vi "IRF measurement.vi"() -> ()   [LabVIEW 2019]
doc: "Main VI for FLS imaging system."
uses:
  <vilib>/event_ctls.llb/usereventprio.ctl
  <instrlib>/niScope/Acquire/Fetch/niScope Multi Fetch Binary 16.vi
  <instrlib>/niScope/Controls/niScope trigger source.ctl
  LaguerreDeconLib/DeconEngineClass/LaguerreDeconEngineClass.lvclass
  SubVI/GlobalVariables.vi
  SubVI/LabJack/LJ Pin Setting.ctl
  <vilib>/Utility/error.llb/DialogType.ctl
  <vilib>/Analysis/NI_AALBase.lvlib
  <vilib>/Utility/miscctls.llb/LVMinMaxIncTypeDef.ctl
  <vilib>/Analysis/baseanly.llb/Mean (DBL).vi
  <vilib>/Utility/miscctls.llb/LVPointTypeDef.ctl
  <vilib>/Instr/_visa.llb/VISA Configure Serial Port (Instr).vi
  SubVI/DigitizerConfiguration/FLImDAQ.ctl
panel:
  out "Record Backlog":i32
  out "Fetch Record #":i32
  out "error out 2":errorcluster caption="error out"
  out "error out":errorcluster
  out "Sync Success?":bool
  out "Disclamer":picture
  out "Calibration #":i8
  out "BG #":i8
  in  "TCP Connect":bool
  out "Help":string
  in  "355nm Laser toggle":bool caption="355nm 750Hz"
  in  "Cali&iRF alignment":bool
  in  "Background":bool
  in  "Aiming beam toggle":bool caption="445nm 15Hz 20mA"
  in  "Auto gain ch3":bool=TRUE
  in  "Auto gain ch2":bool=TRUE
  in  "Auto gain ch1":bool=TRUE
  out "Run #":i8
  in  "StopButton":bool caption="Stop"
  out "Aquisition Status:":bool
  in  "StartButton":bool caption="Start"
  in  "Gain 3":dbl min=0.0 max=4.6 step=0.1
  in  "Gain 2":dbl min=0.0 max=4.6 step=0.1
  in  "Gain 1":dbl min=0.0 max=4.6 step=0.1 format="%#_4g"
  in  "Video Source":enum32{"Camera", "FrameGrabber"}(radio)
  out "Case #":string
  out "System Hardware Connection Status":T1
  out "Channel 3":dbl[][](graph)
  out "Channel 2":dbl[][](graph)
  out "Channel 1":dbl[][](graph)
  in  "Tab Control":T2(tab)
  out "Aq L?":bool
  out "ML?":bool
  out "display loop timing(ms)":u32
  out "Aquisition loop timing(ms)":u32
  out "DisplayLoop":i32
  out "processing loop":i32
  out "processing loop timing(ms)":dbl
  in  "V target(1.5)":dbl=1.3 format="%#_13g"
  out "laser EM lamp V":dbl format="%0.6f"
  in  "Show BG":bool
  out "SysConfigCluster":T3
  out "LJ Pinout":T4={"Ch1 Bias"="DAC0", "Ch2 Bias"="DAC1", "Ch3 Bias"="DAC2", "355 PWM"="FIO0", "AimingBeam PWM"="FIO2", "Laser Ready"="FIO3", "Interlock"="FIO1", "Laser Start/Stop"="FIO1", "Red LED"="FIO1", "Green LED"="DIO3", "Foot Pedal"="DIO15"}
  out "FLImDAQ":T5={"Digitizer 1"="", "Digitizer 2"="", "Channel"=enum."Channel 0", "trigger source"="VAL_EXTERNAL", "trigger level"=0.5, "trigger delay"=1.35e-07, "min sample rate"=12500000000.0, "min record length"=2500, "vertical range"=1.0, "vertical offset"=-0.25, "Waveform to Avg"=2000} caption="FLIm DAQ Configuration" {"trigger delay" format="%^#.4e"; "trigger level" min=0.0 max=3.5 step=0.5 format="%.2f"; "vertical offset" format="%.4f"; "vertical range" format="%.2f"; "min sample rate" format="%#.2p"}
  out "Dig1 Temp":dbl
  out "Dig2 Temp":dbl
  in  "Sys Reconfig":bool
  out "syctimer data out":string
  out "processing Error Out":errorcluster
  out "aquisition loop Error Out":errorcluster
  out "V1":dbl[](array[numeric])
  out "V2":dbl[](array[numeric])
  out "V3":dbl[](array[numeric])
  out "V1 Size":i32
  out "V2 Size":i32
  out "V3 Size":i32
  out "data Size":i32[](array[numeric])
  out "State log":string
  in  "Quit":bool
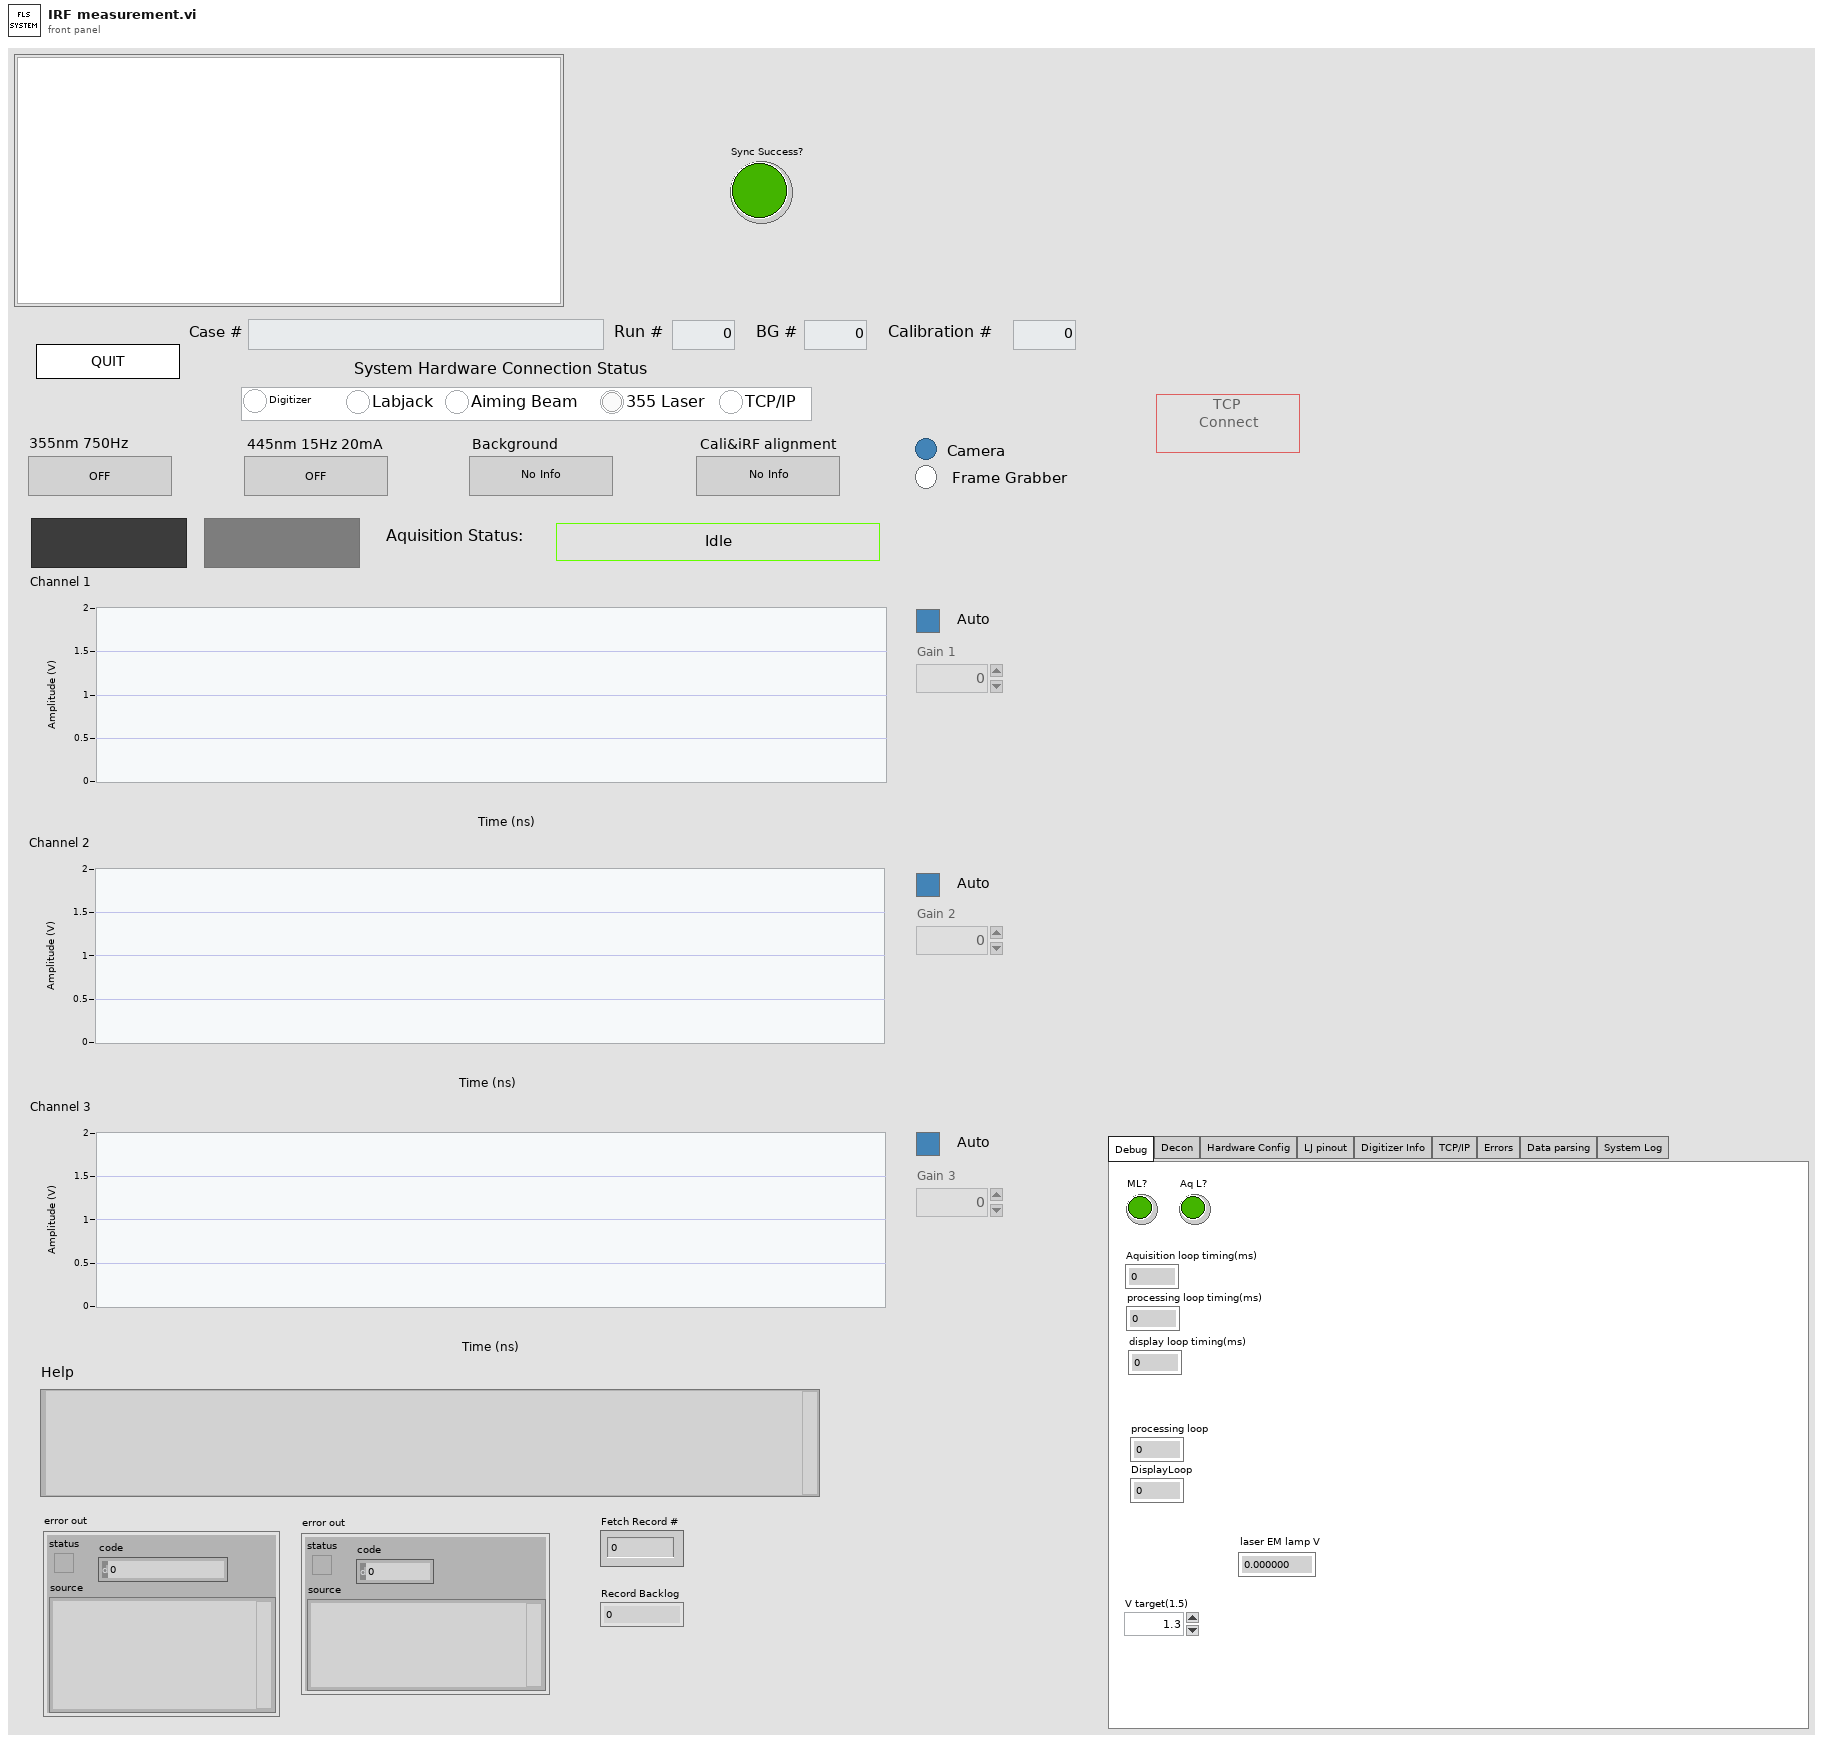
[diagram p1: front panel]
types:
  T1 = cluster{"Digitizer":bool, "Labjack":bool, "Aiming Beam":bool, "355 Laser":bool, "TCP/IP":bool}
  T2 = enum32{"Debug", "Decon", "Hardware Config", "LJ pinout", "Digitizer Info", "TCP/IP", "Errors", "Data parsing", "System Log"}
  T3 = cluster{"Ch1Enable?":bool, "Ch2Enable?":bool, "Ch3Enable?":bool, "Ch1AutoGain?":bool, "Ch2AutoGain?":bool, "Ch3AutoGain?":bool, "AimingBeamEnable?":bool}
  T4 = typedef "LJ Pin Setting.ctl" = cluster{"Ch1 Bias":string, "Ch2 Bias":string, "Ch3 Bias":string, "355 PWM":string, "AimingBeam PWM":string, "Laser Ready":string, "Interlock":string, "Laser Start/Stop":string, "Red LED":string, "Green LED":string, "Foot Pedal":string}
  T5 = typedef "FLImDAQ.ctl" = cluster{"Digitizer 1":refnum<k15>, "Digitizer 2":refnum<k15>, "Channel":enum16{"Channel 0", "Channel 1", "Channel 0&1"}, "trigger source":T6, "trigger level":dbl, "trigger delay":dbl, "min sample rate":dbl, "min record length":i32, "vertical range":dbl, "vertical offset":dbl, "Waveform to Avg":i32}
  T6 = typedef "niScope trigger source.ctl" = string
  T7 = enum8{"Enabled", "Disabled", "Disabled and Grayed Out"}
  T8 = typedef "LVPointTypeDef.ctl" = cluster{"Horizontal":i16, "Vertical":i16}
  T9 = cluster{"CH1":dbl[][], "CH2":dbl[][], "CH3":dbl[][]}
  T10 = cluster{"idx":i32, "CH1&2":dbl[][], "CH3":dbl[][]}
  T11 = enum16{"open", "open or create", "create or replace", "create", "open (read-only)"}
  T12 = enum32{"Invalid", "Standard", "Closed", "Hidden", "Minimized", "Maximized"}
  T13 = enum32{"invalid app kind", "Development System", "Run Time System", "Student Edition", "Embedded LabVIEW", "Evaluation", "Custom"}
  T14 = typedef "usereventprio.ctl" = enum32{"high priority", "normal priority"}
  T15 = enum16{"Standard", "Buffered", "CRLF", "Immediate"}
  T16 = cluster{"Core":cluster{"Current VI Reference":refnum<vi>, "Close Panel on Exit?":bool}, "SysConfigCluster":cluster{"Ch1Enable?":bool, "Ch2Enable?":bool, "Ch3Enable?":bool, "Ch1AutoGain?":bool, "Ch2AutoGain?":bool, "Ch3AutoGain?":bool, "AimingBeamEnable?":bool}, "System Status":cluster{"Digitizer":bool, "Labjack":bool, "Aiming Beam":bool, "355 Laser":bool, "TCP/IP":bool}, "IDs":cluster{"RunID":i8, "BG ID":i8, "Cali ID":i8}, "CaseID":string, "DefaultPath":path, "Pathes":cluster{"DataPath":path, "BG Path":path, "iRFPath":path, "CaliPath":path}, "FLImDAQ":cluster{"resource name":refnum<k15>, "resource name 2":refnum<k15>, "Channel":enum16{"Channel 0", "Channel 1", "Channel 0&1"}, "trigger source":T6, "trigger level":dbl, "trigger delay":dbl, "min sample rate":dbl, "min record length":i32, "vertical range":dbl, "vertical offset":dbl, "Waveform to Avg":i32}, "SysRunning?":bool, "AB Cluster":cluster{"Aiming Beam COM Port":refnum<visa-resource-name>, "Min Current":dbl, "Max Current":dbl, "Default Current":dbl, i32}, "LJ Pinout":T4, "355 PWM setting":cluster{"DIO_EF_CLOCK1_DIVISOR":i16, "DIO_EF_CLOCK1_ROLL_VALUE":i32, "DIO#_EF_INDEX":i16, "DIO#_EF_OPTIONS":i16, "DIO#_EF_CONFIG_A":i32}, "AB PWM setting":cluster{"DIO_EF_CLOCK1_DIVISOR":i16, "DIO_EF_CLOCK1_ROLL_VALUE":i32, "DIO#_EF_INDEX":i16, "DIO#_EF_OPTIONS":i16, "DIO#_EF_CONFIG_A":i32}, "Last Trigger":u32, "niTClk sessions":refnum<k20>[], "Laser start tic":u32, "TCP attempt count":i32, "Ch1Data":dbl[][], "Ch2Data":dbl[][], "Ch3Data":dbl[][], "V1":dbl[], "V2":dbl[], "V3":dbl[], "SlowTimer":u32, "FastTimer":u32, "listener ID":refnum<k5>, "TempPath":path, "LED vi reference":refnum<vi>}
  T17 = typedef "LVCursorListTypeDef.ctl" = cluster{"Name":string, "Color":u32, "Style":u8, "Point Style":u8, "Name Visible":bool, "Allow Drag":bool, "Cursor Mode":u32, "Plot":i32, "Index":i32, "Position":cluster{"X":dbl, "Y":dbl}, "X Scale":u32, "Y Scale":u32, "Watch Plots":i32[], "Watch All Plots":bool, "Plot Area":i32, "Label Offset":cluster{"X":dbl, "Y":dbl}}[]
  T18 = cluster{"Name":string, "Color":u32, "Style":u8, "Point Style":u8, "Name Visible":bool, "Allow Drag":bool, "Cursor Mode":u32, "Plot":i32, "Index":i32, "Position":cluster{"X":dbl, "Y":dbl}, "X Scale":u32, "Y Scale":u32, "Watch Plots":i32[], "Watch All Plots":bool, "Plot Area":i32, "Label Offset":cluster{"X":dbl, "Y":dbl}}
  T19 = cluster{"DataPath":path, "BG Path":path, "iRFPath":path, "CaliPath":path}
  T20 = cluster{"DIO_EF_CLOCK1_DIVISOR":i16, "DIO_EF_CLOCK1_ROLL_VALUE":i32, "DIO#_EF_INDEX":i16, "DIO#_EF_OPTIONS":i16, "DIO#_EF_CONFIG_A":i32}
  T21 = cluster{"Aiming Beam COM Port":refnum<visa-resource-name>, "Min Current":dbl, "Max Current":dbl, "Default Current":dbl, i32}
  T22 = cluster{"resource name":refnum<k15>, "resource name 2":refnum<k15>, "Channel":enum16{"Channel 0", "Channel 1", "Channel 0&1"}, "trigger source":T6, "trigger level":dbl, "trigger delay":dbl, "min sample rate":dbl, "min record length":i32, "vertical range":dbl, "vertical offset":dbl, "Waveform to Avg":i32}
  T23 = cluster{"Current VI Reference":refnum<vi>, "Close Panel on Exit?":bool}
  T24 = cluster{"1D Avg":dbl[], "1D Avg":dbl[], "1D Avg":dbl[]}
  T25 = typedef "DialogType.ctl" = u16
  T26 = cluster{"Ch1 iRF":dbl[], "Ch2 iRF":dbl[], "Ch3 iRF":dbl[]}
  T27 = typedef "LJ PWM Setting.ctl" = cluster{"DIO_EF_CLOCK1_DIVISOR":i16, "DIO_EF_CLOCK1_ROLL_VALUE":i32, "DIO#_EF_INDEX":i16, "DIO#_EF_OPTIONS":i16, "DIO#_EF_CONFIG_A":i32}
  T28 = typedef "AimingBeam.ctl" = cluster{"Aiming Beam COM Port":refnum<visa-resource-name>, "Min Current":dbl, "Max Current":dbl, "Default Current":dbl, "Frequency(Hz)":u32}
  T29 = typedef "LVMinMaxIncTypeDef.ctl" = cluster{"Minimum":dbl, "Maximum":dbl, "Increment":dbl}
  T30 = typedef "LVBoundsTypeDef.ctl" = cluster{"Width":u32, "Height":u32}
  T31 = typedef "imagedata.ctl" = cluster{"image type":i32, "image depth":i32, "image":u8[], "mask":u8[], "colors":u32[], "Rectangle":cluster{"left":i16, "top":i16, "right":i16, "bottom":i16}}
  T32 = cluster{"V1 out":dbl, "V2 out":dbl, "V3 out":dbl}
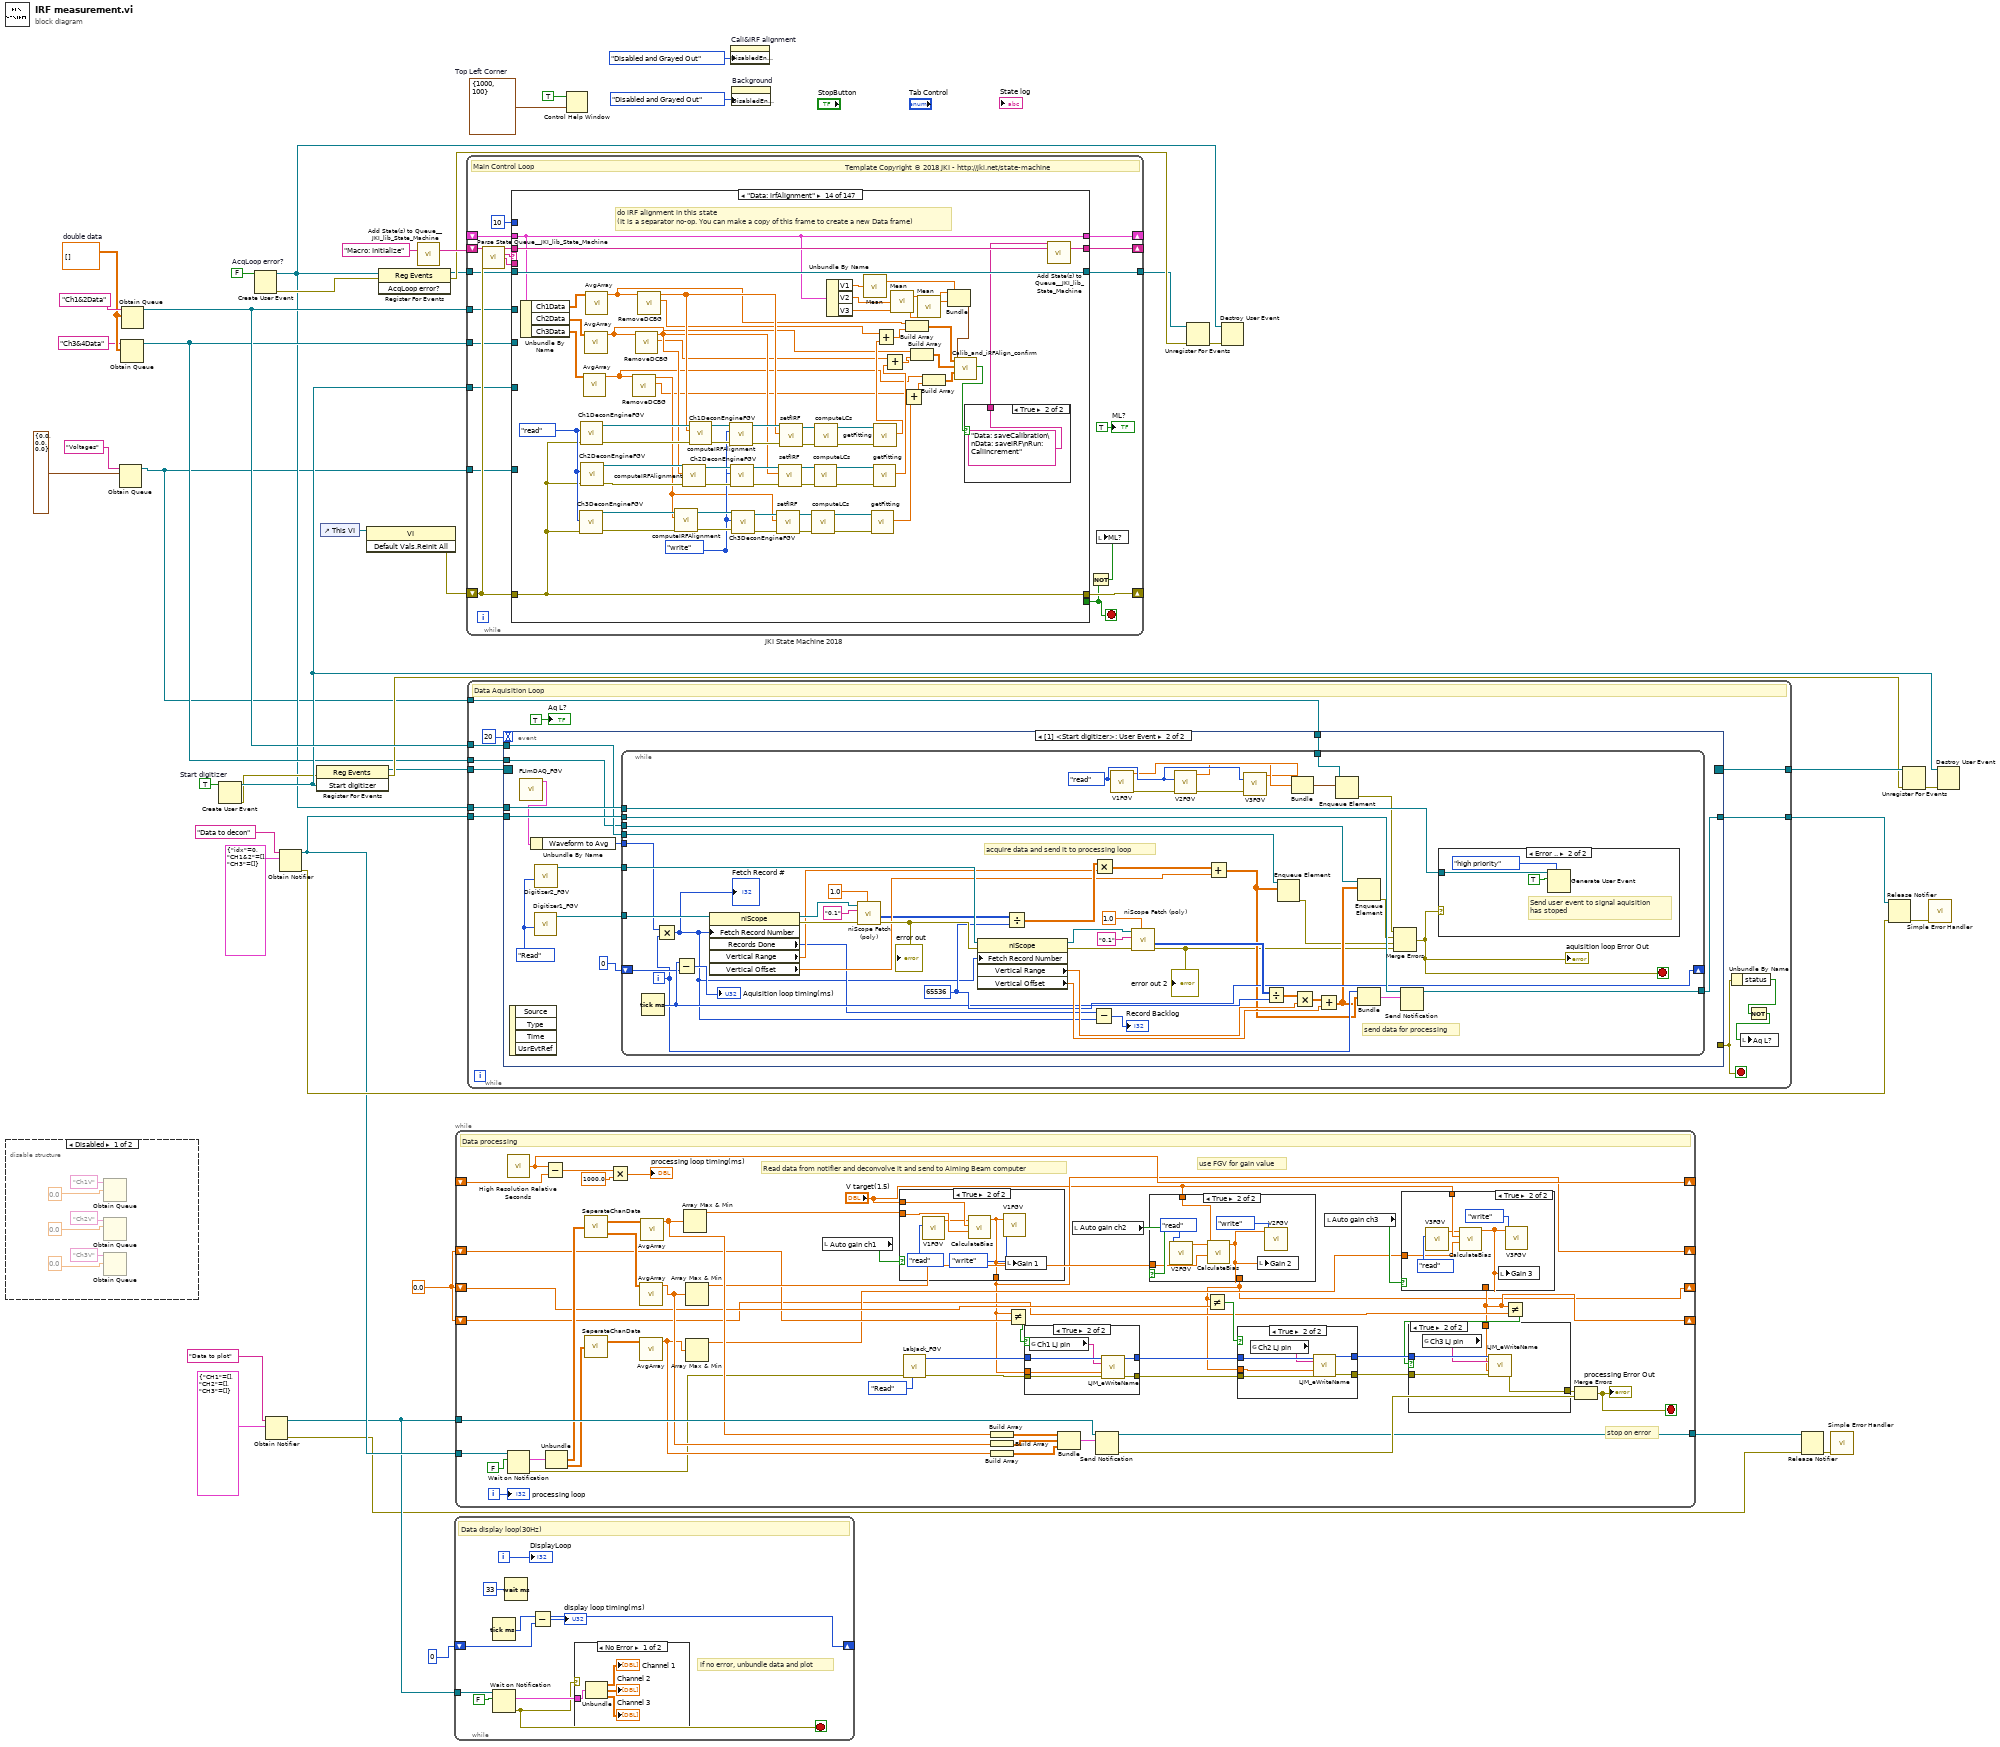
[diagram p0: block diagram]
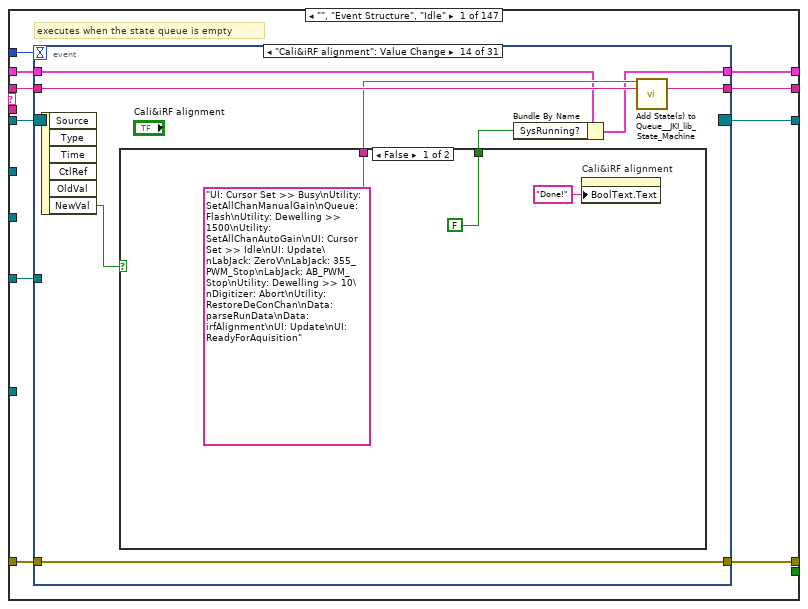
[diagram p3: hidden frame]
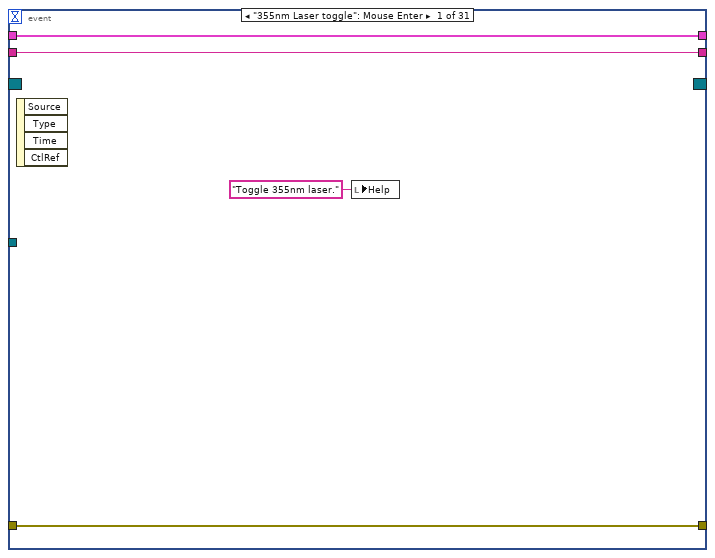
[diagram p4: hidden frame]
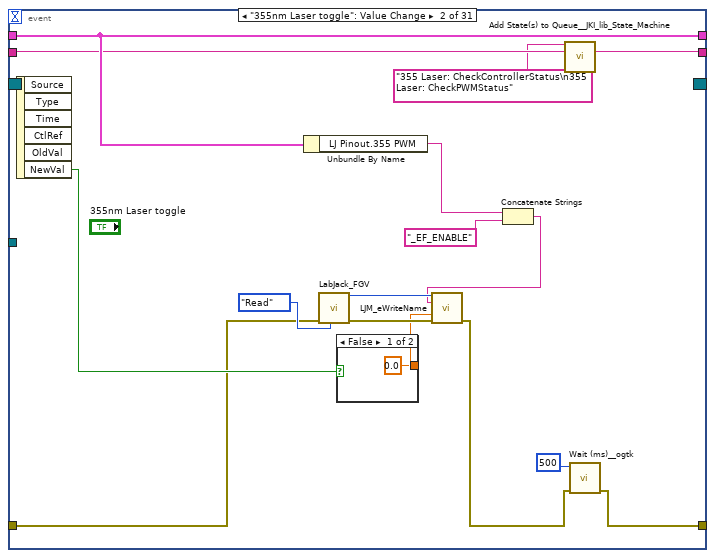
[diagram p5: hidden frame]
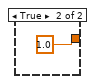
[diagram p6: hidden frame]
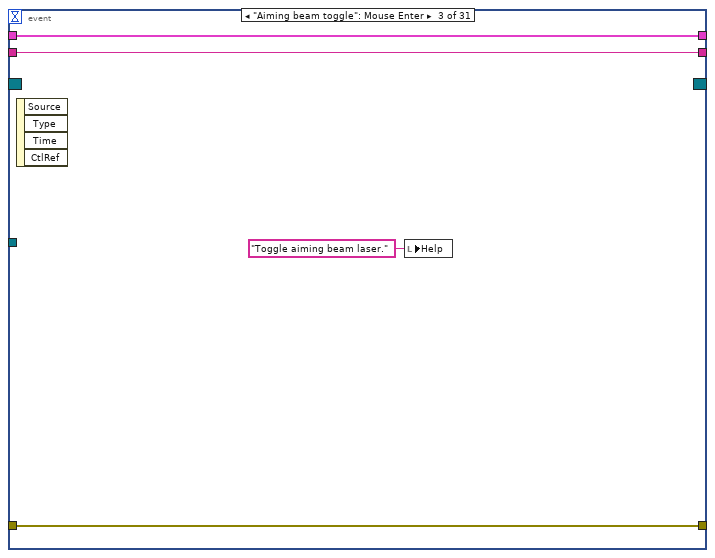
[diagram p7: hidden frame]
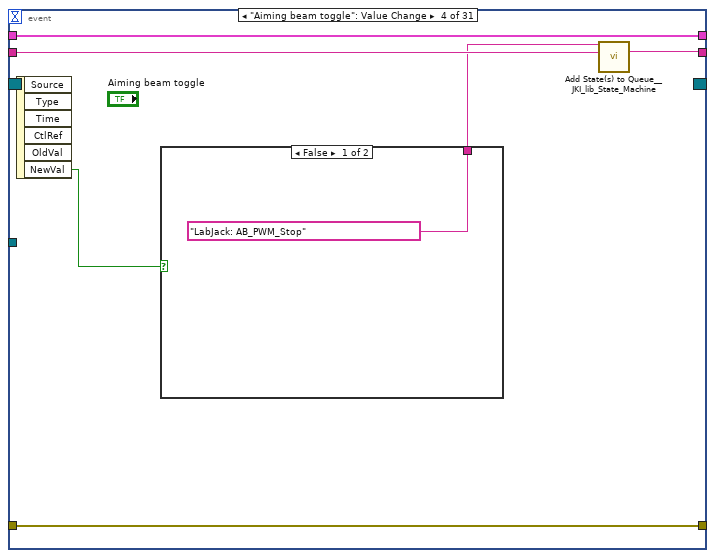
[diagram p8: hidden frame]
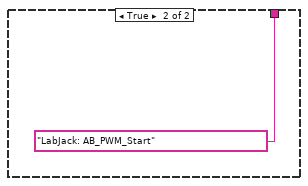
[diagram p9: hidden frame]
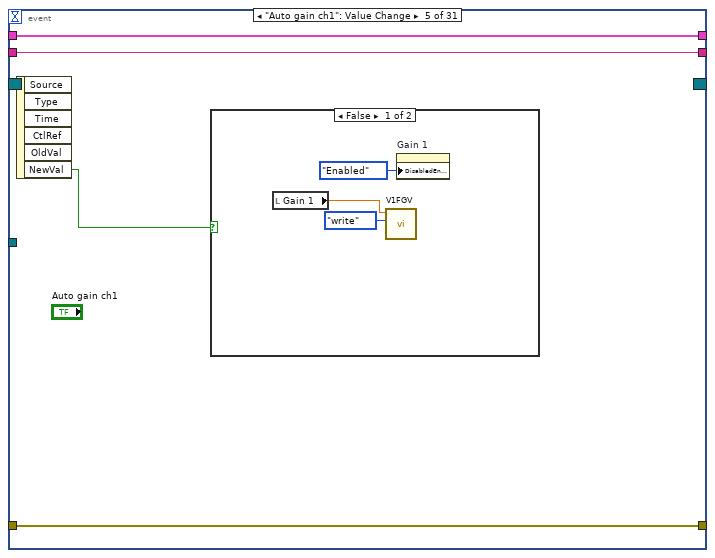
[diagram p10: hidden frame]
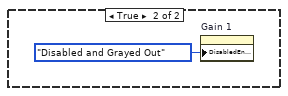
[diagram p11: hidden frame]
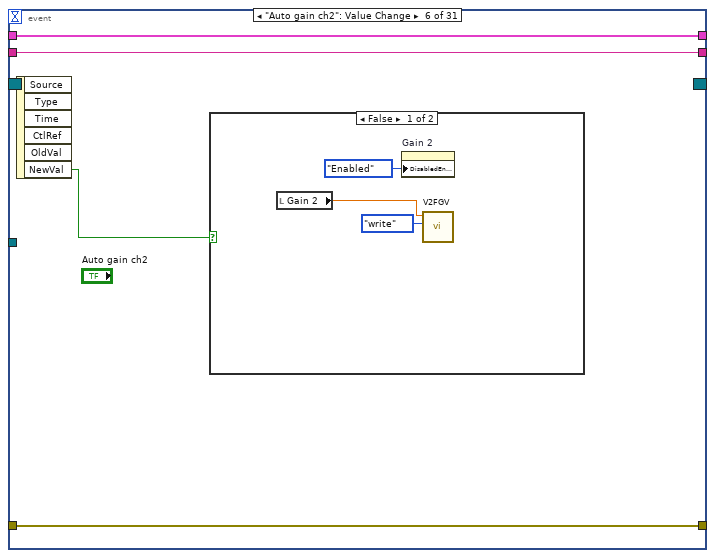
[diagram p12: hidden frame]
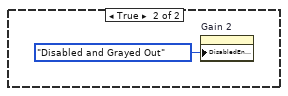
[diagram p13: hidden frame]
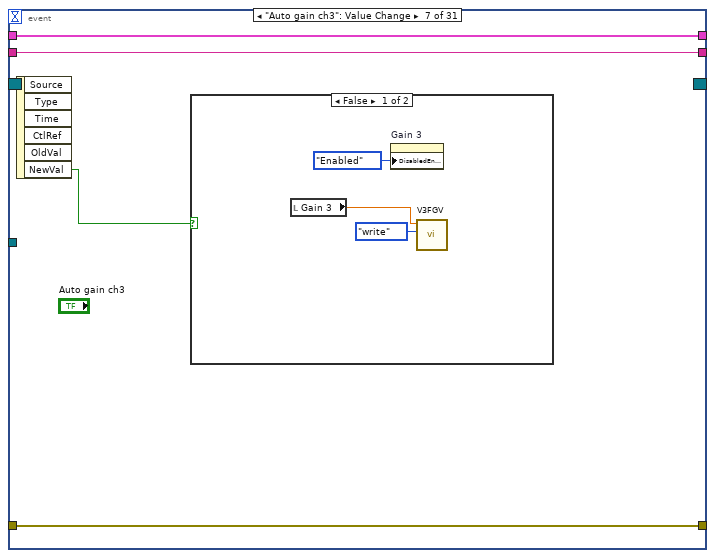
[diagram p14: hidden frame]
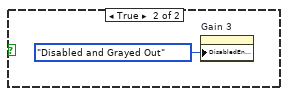
[diagram p15: hidden frame]
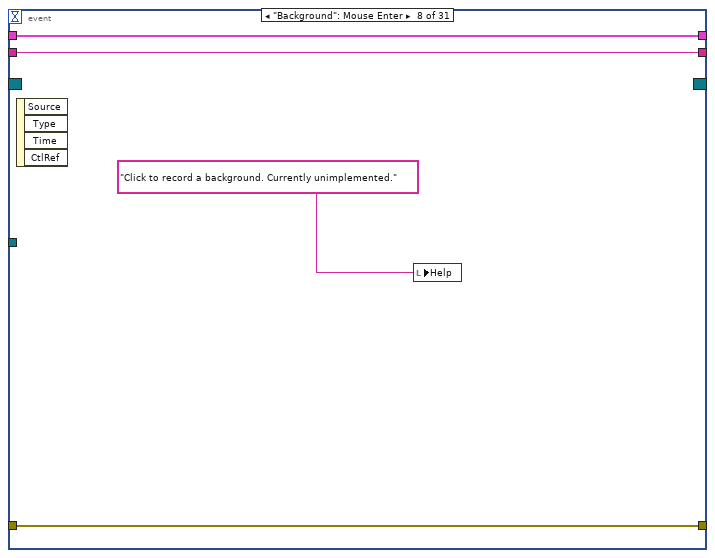
[diagram p16: hidden frame]
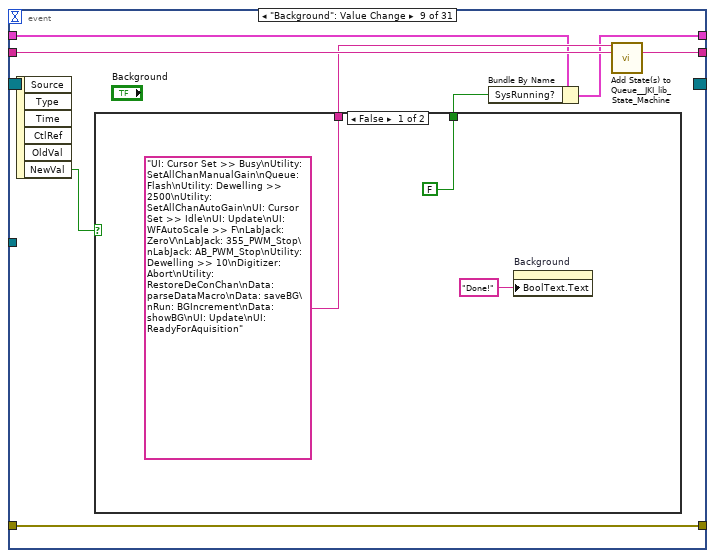
[diagram p17: hidden frame]
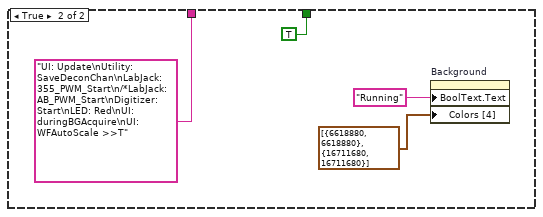
[diagram p18: hidden frame]
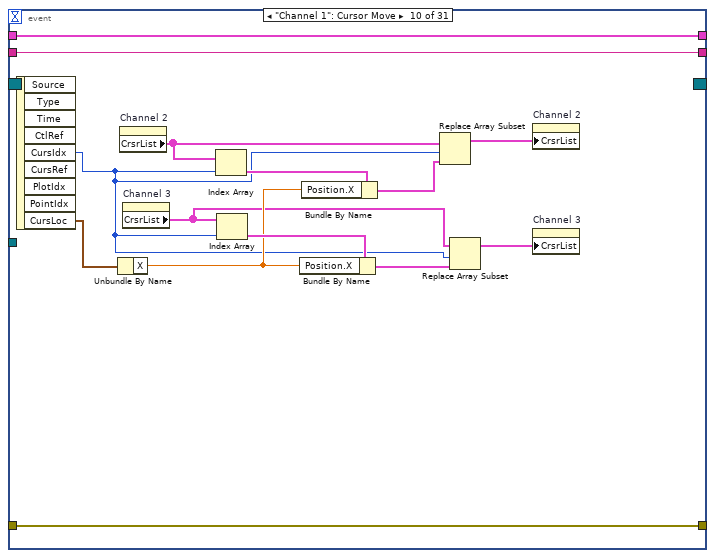
[diagram p19: hidden frame]
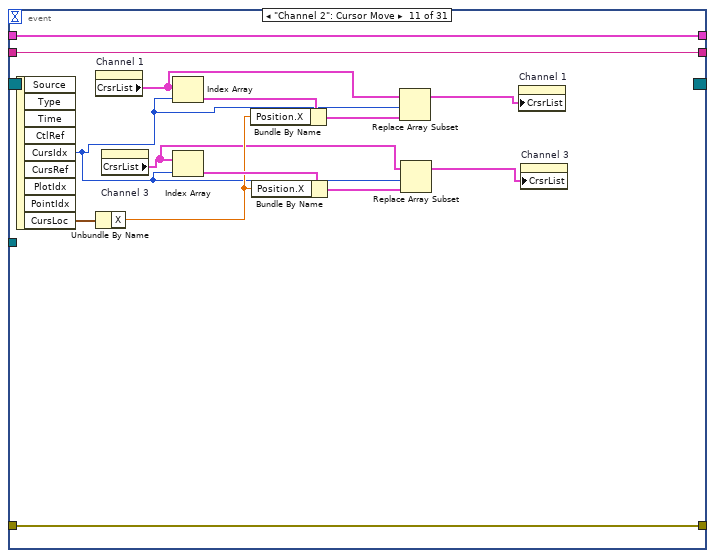
[diagram p20: hidden frame]
diagram:
  w3 = T8 {"Horizontal"=1000, "Vertical"=100}  # Top Left Corner
  w8 = 0.0
  w26 = FALSE  # AcqLoop error?
  w37 = TRUE  # Start digitizer
  w40 = dbl[][] []  # double data
  n1 = disable-structure shown="Disabled" {
    frame Disabled {
      n2 = Obtain Queue(name (unnamed)="Ch1V", element data type=0.0) -> ()  [unwired: 3 in, 3 out]
      n3 = Obtain Queue(name (unnamed)="Ch2V", element data type=0.0) -> ()  [unwired: 3 in, 3 out]
      n4 = Obtain Queue(name (unnamed)="Ch3V", element data type=0.0) -> ()  [unwired: 3 in, 3 out]
    }
    frame Enabled {
    }
  }
  n5 = Obtain Queue(name (unnamed)="Voltages", element data type=cluster{"V1":dbl, "V2":dbl, "V3":dbl} {"V1"=0.0, "V2"=0.0, "V3"=0.0}) -> (queue out=w5:refnum<queue>)  [unwired: 3 in, 2 out]
  n6 = Obtain Queue(name (unnamed)="Ch3&4Data", element data type=w40) -> (queue out=w14:refnum<queue>)  [unwired: 3 in, 2 out]
  n7 = Obtain Queue(name (unnamed)="Ch1&2Data", element data type=w40) -> (queue out=w38:refnum<queue>)  [unwired: 3 in, 2 out]
  n8 = Create User Event(user event datatype=w37) -> (user event=w25:refnum<user-event>, error out=w10:errorcluster)  [unwired: 1 in]
  n9 = Create User Event(user event datatype=w26) -> (user event=w9:refnum<user-event>, error out=w11:errorcluster)  [unwired: 1 in]
  n10 = Obtain Notifier(name (unnamed)="Data to plot", notification data type=T9 {"CH1"=[], "CH2"=[], "CH3"=[]}) -> (notifier out=w18:refnum<notifier>, error out=w15:errorcluster)  [unwired: 2 in, 1 out]
  n11 = Obtain Notifier(name (unnamed)="Data to decon", notification data type=T10 {"idx"=0, "CH1&2"=[], "CH3"=[]}) -> (notifier out=w21:refnum<notifier>, error out=w31:errorcluster)  [unwired: 2 in, 1 out]
  n12 = register-events(error in=w10, w25) -> (reference out=w27:refnum<event-registration>, error out=w34:errorcluster)  [unwired: 1 in]
  n13 = control-ref of="This VI"() -> (w42:refnum<vi>)
  n14 = invoke class="VI" method="Default Vals.Reinit All"(reference=w42) -> (error out=w28:errorcluster)  [unwired: 2 in, 2 out]
  n15 = register-events(error in=w11, w9) -> (reference out=w13:refnum<event-registration>, error out=w23:errorcluster)  [unwired: 1 in]
  n16 = call <vilib>:"Add State(s) to Queue__JKI_lib_State_Machine.vi"("State(s) in (\"\")"="Macro: Initialize") -> ("States Out"=w44:string)  [unwired: 14 in]
  n17 = while {
    tunnel: w18 -> [w59]
    shift-right: [w53] -> _
    shift-left: u32 0 ("millisecond timer value") -> [w57]
    i -> [w51]
    stop <- w52 stop-if-true
    # "if no error, unbundle data and plot"
    # "Data display loop(30Hz)"
    n18 = Tick Count (ms)() -> (millisecond timer value=w53:u32)
    n19 = Wait on Notification(notifier=w59, ignore previous (F)=FALSE) -> (notification=w54:T9, error out=w52:errorcluster)  [unwired: 2 in, 2 out]
    n20 = Wait (ms)(milliseconds to wait=u32 33) -> ()  [unwired: 1 out]
    n21 = Subtract(x=w53, y=w57) -> (x-y=→"display loop timing(ms)":u32)
    n22 = case shown="No Error" w52 {
      tunnel: w54 -> [w63 _]
      frame No Error {
        n23 = Unbundle(w63) -> ("CH1"=→"Channel 1":dbl[][], "CH2"=→"Channel 2":dbl[][], "CH3"=→"Channel 3":dbl[][])
      }
      frame Error {
      }
    }
    "DisplayLoop" <- w51
  }
  n24 = while {
    tunnel: w21 -> [w113]
    shift-right: [w66] -> _
    shift-left: w8 -> [w73]
    tunnel: w18 -> [w105]
    tunnel: [w102] -> w17
    shift-right: [w101] -> _
    shift-left: _ -> [w100]
    shift-right: [w67] -> _
    shift-left: w8 -> [w74]
    shift-right: [w68] -> _
    shift-left: w8 -> [w70]
    i -> [w81]
    stop <- w64 stop-if-true
    # "use FGV for gain value"
    # "stop on error"
    # "Read data from notifier and deconvolve it and send to Aiming Beam computer"
    # "Data processing"
    n25 = call <vilib>:"High Resolution Relative Seconds.vi"() -> ("relative seconds"=w101:dbl)
    n26 = Wait on Notification(notifier=w113, ignore previous (F)=FALSE) -> (notification=w111:T10, error out=w84:errorcluster)  [unwired: 2 in, 2 out]
    n27 = Subtract(x=w101, y=w100) -> (x-y=w99:dbl)
    n28 = Unbundle(w111) -> ("CH1&2"=w83:dbl[][], "CH3"=w82:dbl[][])  [unwired: 1 out]
    n29 = call "SeperateChanData.vi"("Input (Ch1&2)"=w83) -> ("Ch1"=w85:dbl[][], "Ch2"=w90:dbl[][])
    n30 = call "SeperateChanData.vi"("Input (Ch1&2)"=w82) -> ("Ch1"=w110:dbl[][])  [unwired: 1 out]
    n31 = Multiply(x=w99, y=1000.0) -> (x*y=→"processing loop timing(ms)":dbl)
    n32 = call "AvgArray.vi"("2D array"=w90) -> ("1D Avg"=w96:dbl[])  [unwired: 10 in]
    n33 = call "AvgArray.vi"("2D array"=w110) -> ("1D Avg"=w89:dbl[])  [unwired: 10 in]
    n34 = call "AvgArray.vi"("2D array"=w85) -> ("1D Avg"=w103:dbl[])  [unwired: 10 in]
    n35 = Array Max & Min(array=w103) -> (max value=w77:dbl)  [unwired: 3 out]
    n36 = Array Max & Min(array=w96) -> (max value=w75:dbl)  [unwired: 3 out]
    n37 = Array Max & Min(array=w89) -> (max value=w71:dbl)  [unwired: 3 out]
    n38 = local read "Auto gain ch1"() -> (w80:bool)
    n39 = case shown="True" w80 {
      tunnel: [w152 w156] -> w66
      tunnel: w77 -> [_ w158]
      tunnel: "V target(1.5)" -> [_ w157]
      frame False {
        n40 = call "V1FGV.vi"("action"=enum16{"write", "read"}."read") -> ("V1 out"=w152:dbl)  [unwired: 9 in, 1 out]
      }
      frame True {
        n41 = call "V1FGV.vi"("action"=enum16{"write", "read"}."read") -> ("V1 out"=w154:dbl)  [unwired: 9 in, 1 out]
        n42 = call "CalculateBias.vi"("GainV Last"=w158, "Sig Current(V)"=w157, "GainV current"=w154) -> ("V new"=w156:dbl)  [unwired: 8 in]
        n43 = call "V1FGV.vi"("action"=enum16{"write", "read"}."write", "V1 in"=w156) -> ()  [unwired: 8 in, 2 out]
        n44 = local write "Gain 1"(w156) -> ()
      }
    }
    n45 = call "LabJack_FGV.vi"("Operation(Read)"=enum16{"Write", "Read"}."Read" ("Operation"), "error in (no error)"=w84) -> ("error out"=w109:errorcluster, "Read data"=w108:i32)  [unwired: 8 in]
    n46 = Build Array(w103) -> (w88:dbl[][])
    n47 = Build Array(w96) -> (w87:dbl[][])
    n48 = Build Array(w89) -> (w86:dbl[][])
    n49 = Not Equal?(x=w66, y=w73) -> (x != y?=w76:bool)
    n50 = case shown="True" w76 {
      tunnel: w109 -> [w129 w135]
      tunnel: w108 -> [w128 w134]
      tunnel: [w129 w133] -> w95
      tunnel: [w128 w132] -> w92
      tunnel: w66 -> [_ w130]
      frame False {
      }
      frame True {
        n51 = global read "GlobalVariables.vi" "Ch1 LJ pin"() -> (w131:string)
        n52 = call <vilib>:"LJM_eWriteName.vi"("Handle In"=w134, "Name"=w131, "Value"=w130, "error in"=w135) -> ("Handle Out"=w132:i32, "error out"=w133:errorcluster)  [unwired: 10 in]
      }
    }
    n53 = Bundle(w88, w87, w86) -> (w106:cluster{dbl[][], dbl[][], dbl[][]})  [unwired: 1 in]
    n54 = local read "Auto gain ch2"() -> (w79:bool)
    n55 = Send Notification(notification=w106, notifier=w105) -> (notifier out=w102:refnum<notifier>, error out=w104:errorcluster)  [unwired: 1 in]
    n56 = case shown="True" w79 {
      tunnel: [w144 w146] -> w67
      tunnel: w75 -> [_ w151]
      tunnel: "V target(1.5)" -> [_ w150]
      frame False {
        n57 = call "V2FGV.vi"("action"=enum16{"write", "read"}."read") -> ("V2 out"=w144:dbl)  [unwired: 9 in, 1 out]
      }
      frame True {
        n58 = call "V2FGV.vi"("action"=enum16{"write", "read"}."read") -> ("V2 out"=w148:dbl)  [unwired: 9 in, 1 out]
        n59 = call "CalculateBias.vi"("GainV Last"=w151, "Sig Current(V)"=w150, "GainV current"=w148) -> ("V new"=w146:dbl)  [unwired: 8 in]
        n60 = local write "Gain 2"(w146) -> ()
        n61 = call "V2FGV.vi"("action"=enum16{"write", "read"}."write", "V2 in"=w146) -> ()  [unwired: 8 in, 2 out]
      }
    }
    n62 = Not Equal?(x=w67, y=w74) -> (x != y?=w72:bool)
    n63 = case shown="True" w72 {
      tunnel: w95 -> [w120 w127]
      tunnel: [w120 w126] -> w94
      tunnel: w92 -> [w121 w125]
      tunnel: [w121 w124] -> w91
      tunnel: w67 -> [_ w122]
      frame False {
      }
      frame True {
        n64 = global read "GlobalVariables.vi" "Ch2 LJ pin"() -> (w123:string)
        n65 = call <vilib>:"LJM_eWriteName.vi"("Handle In"=w125, "Name"=w123, "Value"=w122, "error in"=w127) -> ("Handle Out"=w124:i32, "error out"=w126:errorcluster)  [unwired: 10 in]
      }
    }
    n66 = local read "Auto gain ch3"() -> (w78:bool)
    n67 = case shown="True" w78 {
      tunnel: w71 -> [_ w142]
      tunnel: "V target(1.5)" -> [_ w141]
      tunnel: [w136 w138] -> w68
      frame False {
        n68 = call "V3FGV.vi"("action"=enum16{"write", "read"}."read") -> ("V3 out"=w136:dbl)  [unwired: 9 in, 1 out]
      }
      frame True {
        n69 = call "V3FGV.vi"("action"=enum16{"write", "read"}."read") -> ("V3 out"=w140:dbl)  [unwired: 9 in, 1 out]
        n70 = call "CalculateBias.vi"("GainV Last"=w142, "Sig Current(V)"=w141, "GainV current"=w140) -> ("V new"=w138:dbl)  [unwired: 8 in]
        n71 = local write "Gain 3"(w138) -> ()
        n72 = call "V3FGV.vi"("action"=enum16{"write", "read"}."write", "V3 in"=w138) -> ()  [unwired: 8 in, 2 out]
      }
    }
    n73 = Not Equal?(x=w68, y=w70) -> (x != y?=w69:bool)
    n74 = case shown="True" w69 {
      tunnel: w94 -> [w114 w119]
      tunnel: [w114 w118] -> w93
      tunnel: w91 -> [_ w117]
      tunnel: w68 -> [_ w115]
      frame False {
      }
      frame True {
        n75 = global read "GlobalVariables.vi" "Ch3 LJ pin"() -> (w116:string)
        n76 = call <vilib>:"LJM_eWriteName.vi"("Handle In"=w117, "Name"=w116, "Value"=w115, "error in"=w119) -> ("error out"=w118:errorcluster)  [unwired: 10 in, 1 out]
      }
    }
    n77 = Merge Errors(w93, w104) -> (w64:errorcluster)
    "processing Error Out" <- w64
    "processing loop" <- w81
  }
  n78 = while "JKI State Machine 2018" {
    shift-right: [w173] -> _
    shift-left: _ -> [w172]
    shift-right: [w175] -> _
    shift-left: w28 -> [w170]
    shift-right: [w174] -> _
    shift-left: w44 -> [w176]
    tunnel: w38 -> [w169]
    tunnel: w14 -> [w168]
    tunnel: w25 -> [w167]
    tunnel: w13 -> [w166]
    tunnel: [w165] -> w12
    tunnel: w5 -> [w161]
    stop <- w164 stop-if-true
    # "Template Copyright © 2018 JKI - http://jki.net/state-machine"
    # "Main Control Loop"
    n79 = call <vilib>:"Parse State Queue__JKI_lib_State_Machine.vi"("State Queue"=w176, "Error In (no error)"=w170) -> ("Remaining States"=w178:string, "Current State"=w160:string, "Arguments"=w177:string)  [unwired: 11 in]
    n80 = case shown="\"Data: irfAlignment\"" w160 {
      selector: w160 -> [_ _ _ _ _ _ _ _ _ _ _ _ _ _ _ _ _ w846 _ _ _ _ _ _ _ _ _ _ _ _ _ _ _ _ _ _ _ _ _ _ _ _ _ _ _ _ _ _ _ _ _ _ _ _ _ _ _ _ _ _ _ _ _ _ _ _ _ _ _ _ _ _ _ _ _ _ _ _ _ _ _ _ _ _ _ _ _ _ _ _ _ _ _ _ _ _ _ _ _ _ _ _ _ _ _ _ _ _ _ _ _ _ _ _ _ _ _ _ _ _ _ _ _ _ _ _ _ _ _ _ _ _ _ _ _ _ _ _ _ _ _ _ _ _ _ _ _]
      tunnel: w178 -> [w188 w464 w497 w503 w529 w555 w579 w602 w618 w653 w681 w716 w721 w788 w830 w839 w844 w850 w875 w883 w906 w911 w920 w926 w949 w964 w976 w985 w1007 w1016 w1038 w1045 w1059 w1079 w1102 w1128 w1166 w1171 w1177 w1204 w1231 w1258 w1263 w1268 w1286 w1336 w1358 w1374 w1386 w1402 w1407 w1419 w1461 w1472 w1510 w1521 w1527 w1538 w1550 w1581 w1612 w1625 w1638 w1652 w1666 w1671 w1680 w1687 w1695 w1720 w1735 w1750 w1765 w1770 w1775 w1784 w1796 w1801 w1809 w1817 w1825 w1833 w1838 w1847 w1864 w1880 w1900 w1921 w1929 w1934 w1942 w1950 w1955 w1981 w2014 w2054 w2070 w2084 w2096 w2106 w2119 w2139 w2149 w2165 w2175 w2185 w2195 w2205 w2215 w2225 w2235 w2240 w2247 w2254 w2264 w2282 w2300 w2308 w2315 w2323 w2328 w2335 w2341 w2347 w2355 w2368 w2375 w2387 w2457 w2468 w2489 w2497 w2503 w2509 w2524 w2569 w2577 w2583 w2588 w2596 w2604 w2612 w2617 w2622 w2627 w2640 w2653]
      tunnel: w177 -> [_ _ _ _ _ _ _ _ _ _ _ _ _ _ _ _ _ _ _ _ _ _ _ _ _ _ _ _ _ w1013 _ _ _ _ _ _ _ _ _ _ _ _ _ _ _ _ _ _ _ _ _ _ _ _ _ _ _ _ w1548 _ _ _ _ _ _ _ _ _ w1688 _ _ _ _ _ _ _ _ _ _ _ _ _ _ _ _ _ _ _ _ _ _ _ _ _ _ _ _ _ _ _ _ _ _ _ _ _ _ _ _ _ _ _ _ _ w2255 _ _ _ _ _ _ _ _ _ _ _ w2370 w2381 _ _ _ w2493 _ _ _ _ _ _ _ w2591 _ _ _ _ _ _ _]
      tunnel: w172 -> [w186 w461 _ w500 w521 w545 w570 w594 w614 w650 w671 w713 w718 w746 w827 w834 w841 w848 w868 w880 w904 w908 w916 w923 w946 w961 w966 w979 w1005 w1014 w1025 w1042 w1047 w1066 w1091 w1120 w1162 w1168 w1174 w1181 w1209 w1235 w1260 w1265 w1279 w1326 w1355 w1359 w1383 w1399 w1404 w1408 w1450 w1465 w1489 w1519 w1524 w1531 w1546 w1564 w1595 w1620 w1633 w1644 w1657 w1668 w1675 w1681 w1692 w1708 w1723 w1739 w1754 w1767 w1772 w1782 w1794 w1798 w1803 w1810 w1820 w1828 w1835 w1844 w1849 w1867 w1895 w1903 w1926 w1931 w1935 w1943 w1952 w1961 w2012 w2050 w2060 w2082 w2094 w2104 w2117 w2135 w2141 w2161 w2173 w2183 w2193 w2203 w2213 w2223 w2233 w2237 w2244 w2251 w2261 w2280 w2297 w2305 w2312 w2320 w2325 w2333 w2339 w2344 w2353 w2365 w2373 w2383 w2454 w2465 w2473 w2494 w2500 w2506 w2517 w2565 w2574 w2580 w2585 w2593 w2601 w2609 w2614 w2619 w2624 w2637 w2650]
      tunnel: [w185 w462 w495 w501 w518 w553 w568 w591 w616 w631 w658 w694 w719 w781 w796 w835 w842 w852 w872 errorcluster {"status"=FALSE, "code"=0, "source"=""} ("error out") w903 w909 w918 w924 w947 w962 w970 w982 w997 w1010 w1026 w1043 w1057 w1077 w1100 w1119 w1164 w1169 w1175 w1182 w1210 w1236 w1261 w1266 w1276 w1317 w1349 w1363 w1384 w1390 w1405 w1411 w1441 w1463 w1477 w1513 w1525 w1536 w1540 w1555 w1586 w1615 w1628 w1643 w1656 w1669 w1673 w1683 w1690 w1710 w1725 w1740 w1755 w1768 w1773 w1776 w1791 w1799 w1807 w1815 w1823 w1831 w1836 w1840 w1852 w1875 w1894 w1915 w1924 w1932 w1940 w1948 w1953 w1963 w2009 w2052 w2058 w2072 w2088 w2098 w2107 w2137 w2140 w2155 w2167 w2178 w2187 w2198 w2207 w2217 w2227 w2238 w2245 w2252 w2262 w2279 w2298 w2306 w2313 w2321 w2326 w2331 w2338 w2345 w2351 w2366 w2371 w2384 w2455 w2464 w2475 w2495 w2501 w2507 w2513 w2559 w2575 w2581 w2586 w2594 w2602 w2610 w2615 w2620 w2625 w2638 w2651] -> w175
      tunnel: w170 -> [w184 w462 w495 w501 w519 w553 w568 w591 w616 w619 w667 w683 w719 w781 w798 w836 w842 w851 w872 w876 w903 w909 w918 w924 w947 w962 w971 w981 w993 w1009 w1027 w1043 w1057 w1077 w1100 w1118 w1164 w1169 w1175 w1186 w1214 w1240 w1261 w1266 w1274 w1320 w1348 w1362 w1384 w1392 w1405 w1410 w1444 w1470 w1482 w1512 w1525 w1533 w1543 w1554 w1585 w1614 w1627 w1642 w1655 w1669 w1672 w1684 w1689 w1709 w1724 w1741 w1756 w1768 w1773 w1778 w1786 w1799 w1807 w1815 w1823 w1831 w1836 w1841 w1859 w1874 w1893 w1914 w1923 w1932 w1940 w1948 w1953 w1979 w2009 w2052 w2057 w2071 w2087 w2097 w2112 w2137 w2144 w2154 w2166 w2177 w2186 w2197 w2206 w2216 w2226 w2238 w2245 w2252 w2262 w2279 w2298 w2306 w2313 w2321 w2326 w2331 w2338 w2345 w2351 w2366 w2372 w2385 w2455 w2464 w2487 w2495 w2501 w2507 w2519 w2558 w2575 w2581 w2586 w2594 w2602 w2610 w2615 w2620 w2625 w2638 w2651]
      tunnel: [w187 w463 w496 w502 w528 w554 w578 w601 w617 w652 w680 w715 w720 w787 w829 w838 w843 w849 w874 w882 w905 w910 w919 w925 w948 w963 w975 w984 w1006 w1015 w1037 w1044 w1058 w1078 w1101 w1127 w1165 w1170 w1176 w1203 w1230 w1257 w1262 w1267 w1285 w1335 w1357 w1373 w1385 w1401 w1406 w1418 w1460 w1471 w1509 w1520 w1526 w1537 w1549 w1580 w1611 w1624 w1637 w1651 w1665 w1670 w1679 w1686 w1694 w1719 w1734 w1749 w1764 w1769 w1774 w1783 w1795 w1800 w1808 w1816 w1824 w1832 w1837 w1846 w1863 w1879 w1899 w1920 w1928 w1933 w1941 w1949 w1954 w1980 w2013 w2053 w2069 w2083 w2095 w2105 w2118 w2138 w2148 w2164 w2174 w2184 w2194 w2204 w2214 w2224 w2234 w2239 w2246 w2253 w2263 w2281 w2299 w2307 w2314 w2322 w2327 w2334 w2340 w2346 w2354 w2367 w2374 w2386 w2456 w2467 w2488 w2496 w2502 w2508 w2523 w2568 w2576 w2582 w2587 w2595 w2603 w2611 w2616 w2621 w2626 w2639 w2652] -> w174
      tunnel: [_ _ _ _ _ _ _ _ _ _ _ _ _ _ _ _ _ _ _ _ TRUE _ _ _ _ _ _ _ _ _ _ _ _ _ _ _ _ _ _ _ _ _ _ _ _ _ _ _ _ _ _ _ _ _ _ _ _ _ _ _ _ _ _ _ _ _ _ _ _ _ _ _ _ _ _ _ _ _ _ _ _ _ _ _ _ _ _ _ _ _ _ _ _ _ _ _ _ _ _ _ _ _ _ _ _ _ _ _ _ _ _ _ _ _ _ _ _ _ _ _ _ _ _ _ _ _ _ _ _ _ _ _ _ _ _ _ _ _ _ _ _ _ _ _ _ _ _] -> w164
      tunnel: [w183 w461 w469 w500 w522 w545 w570 w594 w614 w650 w671 w713 w718 w746 w827 w834 w841 w848 w873 w880 w904 w908 w916 w923 w946 w961 w967 w980 w1005 w1014 w1025 w1042 w1048 w1067 w1092 w1121 w1163 w1168 w1174 w1181 w1209 w1235 w1260 w1265 w1279 w1327 w1355 w1360 w1383 w1400 w1404 w1409 w1450 w1469 w1489 w1519 w1524 w1534 w1546 w1564 w1595 w1620 w1633 w1644 w1657 w1668 w1676 w1681 w1692 w1708 w1723 w1739 w1754 w1767 w1772 w1782 w1794 w1798 w1804 w1811 w1821 w1829 w1835 w1845 w1850 w1873 w1882 w1916 w1927 w1931 w1936 w1944 w1952 w1962 w2012 w2050 w2060 w2082 w2094 w2104 w2117 w2135 w2142 w2161 w2173 w2183 w2193 w2203 w2213 w2223 w2233 w2237 w2244 w2251 w2261 w2280 w2297 w2305 w2312 w2320 w2325 w2333 w2339 w2344 w2353 w2365 w2373 w2383 w2454 w2465 w2474 w2494 w2500 w2506 w2518 w2565 w2574 w2580 w2585 w2593 w2601 w2609 w2614 w2619 w2624 w2637 w2650] -> w173
      tunnel: 10 ("Timeout") -> [w182 _ _ _ _ _ _ _ _ _ _ _ _ _ _ _ _ _ _ _ _ _ _ _ _ _ _ _ _ _ _ _ _ _ _ _ _ _ _ _ _ _ _ _ _ _ _ _ _ _ _ _ _ _ _ _ _ _ _ _ _ _ _ _ _ _ _ _ _ _ _ _ _ _ _ _ _ _ _ _ _ _ _ _ _ _ _ _ _ _ _ _ _ _ _ _ _ _ _ _ _ _ _ _ _ _ _ _ _ _ _ _ _ _ _ _ _ _ _ _ _ _ _ _ _ _ _ _ _ _ _ _ _ _ _ _ _ _ _ _ _ _ _ _ _ _ _]
      tunnel: w169 -> [_ _ _ _ w526 _ _ _ _ _ _ _ _ _ _ _ _ _ _ _ _ _ _ _ _ _ _ _ _ _ _ _ _ _ _ _ _ _ _ _ _ _ _ _ _ _ _ _ _ _ _ _ _ _ _ _ _ _ _ _ _ _ _ _ _ _ _ _ _ _ _ _ _ _ _ w1779 w1790 _ _ _ _ _ _ _ _ _ _ _ _ _ _ _ _ _ _ _ _ _ _ _ _ _ _ _ _ _ _ _ _ _ _ _ _ _ _ _ _ _ _ _ _ _ _ _ _ _ _ _ _ _ _ _ _ _ _ _ _ _ _ _ _ _ _ _ _ _ _]
      tunnel: w168 -> [_ _ _ _ w525 _ _ _ _ _ _ _ _ _ _ _ _ _ _ _ _ _ _ _ _ _ _ _ _ _ _ _ _ _ _ _ _ _ _ _ _ _ _ _ _ _ _ _ _ _ _ _ _ _ _ _ _ _ _ _ _ _ _ _ _ _ _ _ _ _ _ _ _ _ _ w1780 w1789 _ _ _ _ _ _ _ _ _ _ _ _ _ _ _ _ _ _ _ _ _ _ _ _ _ _ _ _ _ _ _ _ _ _ _ _ _ _ _ _ _ _ _ _ _ _ _ _ _ _ _ _ _ _ _ _ _ _ _ _ _ _ _ _ _ _ _ _ _ _]
      tunnel: w167 -> [w181 _ _ _ _ _ _ _ _ _ _ _ _ _ _ _ _ _ _ _ _ _ _ _ _ _ _ _ _ _ _ _ _ _ _ _ _ _ _ _ _ _ _ _ _ _ w1351 _ _ _ _ _ _ _ _ _ _ _ _ _ _ _ _ _ _ _ _ _ _ _ _ _ _ _ _ _ _ _ _ _ _ _ _ _ _ _ _ _ _ _ _ _ _ _ _ _ _ _ _ _ _ _ _ _ _ _ _ _ _ _ _ _ _ _ _ _ _ _ _ _ _ _ _ _ _ _ _ _ _ _ _ _ _ _ _ _ _ _ _ _ _ _ _ _ _ _ _]
      tunnel: w166 -> [w180 w460 w480 w499 w527 w552 w577 w600 w615 w651 w679 w714 w717 w786 w828 w833 w840 w845 w860 w879 w902 w907 w917 w922 w938 w960 w965 w977 w992 w1008 w1036 w1041 w1056 w1076 w1099 w1117 w1161 w1167 w1173 w1180 w1208 w1234 w1259 w1264 w1269 w1297 w1356 w1372 w1382 w1387 w1403 w1417 w1459 w1462 w1508 w1511 w1523 w1530 w1539 w1551 w1582 w1613 w1626 w1641 w1654 w1667 w1678 w1685 w1693 w1718 w1733 w1736 w1751 w1766 w1771 w1781 w1788 w1797 w1806 w1814 w1818 w1826 w1834 w1839 w1848 w1868 w1883 w1904 w1922 w1930 w1938 w1946 w1951 w1959 w2011 w2051 w2068 w2081 w2093 w2103 w2116 w2136 w2143 w2163 w2172 w2182 w2192 w2202 w2212 w2222 w2232 w2236 w2243 w2250 w2260 w2278 w2296 w2304 w2311 w2316 w2324 w2330 w2337 w2343 w2349 w2360 w2369 w2380 w2453 w2466 w2477 w2490 w2498 w2504 w2516 w2567 w2572 w2578 w2584 w2592 w2600 w2608 w2613 w2618 w2623 w2636 w2649]
      tunnel: [w179 w460 w480 w499 w527 w552 w577 w600 w615 w651 w679 w714 w717 w786 w828 w833 w840 w845 w860 w879 w902 w907 w917 w922 w938 w960 w965 w977 w992 w1008 w1036 w1041 w1056 w1076 w1099 w1117 w1161 w1167 w1173 w1180 w1208 w1234 w1259 w1264 w1269 w1297 w1356 w1372 w1382 w1387 w1403 w1417 w1459 w1462 w1508 w1511 w1523 w1530 w1539 w1551 w1582 w1613 w1626 w1641 w1654 w1667 w1678 w1685 w1693 w1718 w1733 w1736 w1751 w1766 w1771 w1781 w1788 w1797 w1806 w1814 w1818 w1826 w1834 w1839 w1848 w1868 w1883 w1904 w1922 w1930 w1938 w1946 w1951 w1959 w2011 w2051 w2068 w2081 w2093 w2103 w2116 w2136 w2143 w2163 w2172 w2182 w2192 w2202 w2212 w2222 w2232 w2236 w2243 w2250 w2260 w2278 w2296 w2304 w2311 w2316 w2324 w2330 w2337 w2343 w2349 w2360 w2369 w2380 w2453 w2466 w2477 w2490 w2498 w2504 w2516 w2567 w2572 w2578 w2584 w2592 w2600 w2608 w2613 w2618 w2623 w2636 w2649] -> w165
      tunnel: w161 -> [_ _ _ _ w520 _ _ _ _ _ _ _ _ _ _ _ _ _ _ _ _ _ _ _ _ _ _ _ _ _ _ _ _ _ _ _ _ _ _ _ _ _ _ _ _ _ _ _ _ _ _ _ _ _ _ _ _ _ _ _ _ _ _ _ _ _ _ _ _ _ _ _ _ _ _ _ w1787 _ _ _ _ _ _ _ _ _ _ _ _ _ _ _ _ _ _ _ _ _ _ _ _ _ _ _ _ _ _ _ _ _ _ _ _ _ _ _ _ _ _ _ _ _ _ _ _ _ _ _ _ _ _ _ _ _ _ _ _ _ _ _ _ _ _ _ _ _ _]
      frame "", "Event Structure", "Idle" {
        # "executes when the state queue is empty"
        n81 = event shown="[13] \"Cali&iRF alignment\": Value Change" {
          selector: w180 -> [_ _ _ _ _ _ _ _ _ _ _ _ _ _ _ _ _ _ _ _ _ _ _ _ _ _ _ _ _ _ _]
          dyn-events: [_ _ _ _ _ _ _ _ _ _ _ _ _ _ _ _ _ _ _ _ _ _ _ _ _ _ _ _ _ _ _] -> w179
          timeout: w182 -> [_ _ _ _ _ _ _ _ _ _ _ _ _ _ _ _ _ _ _ _ _ _ _ _ _ _ _ _ _ _ _]
          tunnel: w188 -> [w192 w198 w214 w217 w226 w232 w240 w250 w257 w279 w293 w307 w311 w318 w331 w336 w341 w346 w349 w355 w365 w372 w380 w396 w408 w415 w419 w423 w430 w438 w454]
          tunnel: [w192 w197 w214 w216 w226 w232 w240 w250 w256 w279 w293 w307 w311 w317 w331 w336 w341 w345 w348 w355 w366 w372 w381 w396 w409 w415 w419 w422 w431 w437 w455] -> w187
          tunnel: w186 -> [w190 w201 w212 w219 w225 w233 w241 w248 w252 w277 w291 w305 w309 w313 w329 w334 w339 w342 w350 w353 w361 w370 w373 w394 w403 w413 w417 w424 w429 w435 w452]
          tunnel: [w191 w194 w213 w220 w224 w231 w239 w249 w258 w278 w292 w306 w310 w319 w330 w335 w340 w344 w351 w354 w362 w371 w379 w395 w404 w414 w418 w425 w432 w436 w453] -> w185
          tunnel: w184 -> [w191 w199 w213 w220 w224 w231 w239 w249 w258 w278 w292 w306 w310 w319 w330 w335 w340 w344 w351 w354 w362 w371 w379 w395 w407 w414 w418 w425 w432 w436 w453]
          tunnel: [w190 w201 w212 w219 w225 w233 w241 w248 w253 w277 w291 w305 w309 w314 w329 w334 w339 w342 w350 w353 w363 w370 w374 w394 w410 w413 w417 w424 w429 w435 w452] -> w183
          tunnel: w181 -> [_ _ _ _ _ _ _ _ _ _ _ _ _ _ _ _ _ _ _ _ _ _ _ _ _ _ _ _ _ _ _]
          event "355nm Laser toggle": Mouse Enter {
            n82 = event-data() -> ()  [unwired: 1 in, 4 out]
            n83 = local write "Help"("Toggle 355nm laser." ("Help")) -> ()
          }
          event "355nm Laser toggle": Value Change {
            n84 = event-data() -> ("NewVal"=w200:bool)  [unwired: 1 in, 5 out]
            n85 = Unbundle By Name(w201) -> ("LJ Pinout.355 PWM"=w205:string)
            n86 = call "LabJack_FGV.vi"("Operation(Read)"=enum16{"Write", "Read"}."Read" ("Operation"), "error in (no error)"=w199) -> ("error out"=w206:errorcluster, "Read data"=w207:i32)  [unwired: 8 in]
            n87 = case shown="False" w200 {
              tunnel: [0.0 ("Value") 1.0 ("Value")] -> w203
              frame False {
              }
              frame True {
              }
            }
            n88 = Concatenate Strings(w205, "_EF_ENABLE" ("string")) -> (w202:string)
            n89 = call <vilib>:"LJM_eWriteName.vi"("Handle In"=w207, "Name"=w202, "Value"=w203, "error in"=w206) -> ("error out"=w195:errorcluster)  [unwired: 10 in, 1 out]
            n90 = call <vilib>:"Add State(s) to Queue__JKI_lib_State_Machine.vi"("State(s) in Front (\"\")"="355 Laser: CheckControllerStatus\n355 Laser: CheckPWMStatus" ("State(s) in Front (\"\")"), "State(s) in (\"\")"=w198) -> ("States Out"=w197:string)  [unwired: 13 in]
            n91 = call <userlib>:"Wait (ms)__ogtk.vi"("error in (no error)"=w195, "milliseconds to wait"=u32 500) -> ("error out"=w194:errorcluster)  [unwired: 8 in, 1 out]
          }
          event "Aiming beam toggle": Mouse Enter {
            n92 = event-data() -> ()  [unwired: 1 in, 4 out]
            n93 = local write "Help"("Toggle aiming beam laser." ("Help")) -> ()
          }
          event "Aiming beam toggle": Value Change {
            n94 = event-data() -> ("NewVal"=w218:bool)  [unwired: 1 in, 5 out]
            n95 = case shown="False" w218 {
              tunnel: ["LabJack: AB_PWM_Stop" ("State(s) in Front (\"\")") "LabJack: AB_PWM_Start" ("State(s) in Front (\"\")")] -> w215
              frame False {
              }
              frame True {
              }
            }
            n96 = call <vilib>:"Add State(s) to Queue__JKI_lib_State_Machine.vi"("State(s) in Front (\"\")"=w215, "State(s) in (\"\")"=w217) -> ("States Out"=w216:string)  [unwired: 13 in]
          }
          event "Auto gain ch1": Value Change {
            n97 = event-data() -> ("NewVal"=w223:bool)  [unwired: 1 in, 5 out]
            n98 = case shown="False" w223 {
              frame False {
                n99 = local read "Gain 1"() -> (w227:dbl)
                n100 = call "V1FGV.vi"("action"=enum16{"write", "read"}."write", "V1 in"=w227) -> ()  [unwired: 8 in, 2 out]
                n101 = property on="Gain 1" class="DigNum (strict)"("DisabledEnum"=T7."Enabled" ("Disabled")) -> ()  [unwired: 2 in, 2 out]
              }
              frame True {
                n102 = property on="Gain 1" class="DigNum (strict)"("DisabledEnum"=T7."Disabled and Grayed Out" ("Disabled")) -> ()  [unwired: 2 in, 2 out]
              }
            }
          }
          event "Auto gain ch2": Value Change {
            n103 = event-data() -> ("NewVal"=w234:bool)  [unwired: 1 in, 5 out]
            n104 = case shown="False" w234 {
              frame False {
                n105 = local read "Gain 2"() -> (w235:dbl)
                n106 = property on="Gain 2" class="DigNum (strict)"("DisabledEnum"=T7."Enabled" ("Disabled")) -> ()  [unwired: 2 in, 2 out]
                n107 = call "V2FGV.vi"("action"=enum16{"write", "read"}."write", "V2 in"=w235) -> ()  [unwired: 8 in, 2 out]
              }
              frame True {
                n108 = property on="Gain 2" class="DigNum (strict)"("DisabledEnum"=T7."Disabled and Grayed Out" ("Disabled")) -> ()  [unwired: 2 in, 2 out]
              }
            }
          }
          event "Auto gain ch3": Value Change {
            n109 = event-data() -> ("NewVal"=w242:bool)  [unwired: 1 in, 5 out]
            n110 = case shown="False" w242 {
              frame False {
                n111 = local read "Gain 3"() -> (w243:dbl)
                n112 = property on="Gain 3" class="DigNum (strict)"("DisabledEnum"=T7."Enabled" ("Disabled")) -> ()  [unwired: 2 in, 2 out]
                n113 = call "V3FGV.vi"("action"=enum16{"write", "read"}."write", "V3 in"=w243) -> ()  [unwired: 8 in, 2 out]
              }
              frame True {
                n114 = property on="Gain 3" class="DigNum (strict)"("DisabledEnum"=T7."Disabled and Grayed Out" ("Disabled")) -> ()  [unwired: 2 in, 2 out]
              }
            }
          }
          event "Background": Mouse Enter {
            n115 = event-data() -> ()  [unwired: 1 in, 4 out]
            n116 = local write "Help"("Click to record a background. Currently unimplemented." ("Help")) -> ()
          }
          event "Background": Value Change {
            n117 = event-data() -> ("NewVal"=w254:bool)  [unwired: 1 in, 5 out]
            n118 = case shown="False" w254 {
              tunnel: ["UI: Cursor Set >> Busy\nUtility: SetAllChanManualGain\nQueue: Flash\nUtility: Dewelling >> 2500\nUtility: SetAllChanAutoGain\nUI: Cursor Set >> Idle\nUI: Update\nUI: WFAutoScale >> F\nLabJack: ZeroV\nLabJack: 355_PWM_Stop\nLabJack: AB_PWM_Stop\nUtility: Dewelling >> 10\nDigitizer: Abort\nUtility: RestoreDeConChan\nData: parseDataMacro\nData: saveBG\nRun: BGIncrement\nData: showBG\nUI: Update\nUI: ReadyForAquisition" "UI: Update\nUtility: SaveDeconChan\nLabJack: 355_PWM_Start\n/*LabJack: AB_PWM_Start\nDigitizer: Start\nLED: Red\nUI: duringBGAcquire\nUI: WFAutoScale >>T"] -> w255
              tunnel: [FALSE TRUE] -> w251
              frame False {
                n119 = property on="Background" class="Bool (strict)"("BoolText.Text"="Done!" ("Boolean Text.Text")) -> ()  [unwired: 2 in, 2 out]
              }
              frame True {
                n120 = property on="Background" class="Bool (strict)"("BoolText.Text"="Running" ("Boolean Text.Text"), "Colors [4]"=cluster{u32, u32}[] [{6618880, 6618880}, {16711680, 16711680}]) -> ()  [unwired: 2 in, 2 out]
              }
            }
            n121 = Bundle By Name(cluster=w252, "SysRunning?"=w251) -> (w253:T16)
            n122 = call <vilib>:"Add State(s) to Queue__JKI_lib_State_Machine.vi"("State(s) in Front (\"\")"=w255, "State(s) in (\"\")"=w257) -> ("States Out"=w256:string)  [unwired: 13 in]
          }
          event "Channel 1": Cursor Move {
            n123 = event-data() -> ("CursIdx"=w268:i32, "CursLoc"=w275:cluster{"X":dbl, "Y":dbl})  [unwired: 1 in, 7 out]
            n124 = Unbundle By Name(w275) -> ("X"=w273:dbl)
            n125 = property on="Channel 2" class="WFGraph (strict)"() -> ("CrsrList"=w272:T17)  [unwired: 2 in, 2 out]
            n126 = property on="Channel 3" class="WFGraph (strict)"() -> ("CrsrList"=w269:T17)  [unwired: 2 in, 2 out]
            n127 = Index Array(array=w272, index=w268) -> (element=w276:T18)
            n128 = Index Array(array=w269, index=w268) -> (element=w274:T18)
            n129 = Bundle By Name(cluster=w274, "Position.X"=w273) -> (w267:T18)
            n130 = Bundle By Name(cluster=w276, "Position.X"=w273) -> (w271:T18)
            n131 = Replace Array Subset(array=w272, new element=w271, index=w268) -> (w270:T17)
            n132 = Replace Array Subset(array=w269, new element=w267, index=w268) -> (w266:T17)
            n133 = property on="Channel 2" class="WFGraph (strict)"("CrsrList"=w270) -> ()  [unwired: 2 in, 2 out]
            n134 = property on="Channel 3" class="WFGraph (strict)"("CrsrList"=w266) -> ()  [unwired: 2 in, 2 out]
          }
          event "Channel 2": Cursor Move {
            n135 = event-data() -> ("CursIdx"=w284:i32, "CursLoc"=w290:cluster{"X":dbl, "Y":dbl})  [unwired: 1 in, 7 out]
            n136 = property on="Channel 1" class="WFGraph (strict)"() -> ("CrsrList"=w282:T17)  [unwired: 2 in, 2 out]
            n137 = Unbundle By Name(w290) -> ("X"=w287:dbl)
            n138 = property on="Channel 3" class="WFGraph (strict)"() -> ("CrsrList"=w285:T17)  [unwired: 2 in, 2 out]
            n139 = Index Array(array=w282, index=w284) -> (element=w289:T18)
            n140 = Index Array(array=w285, index=w284) -> (element=w288:T18)
            n141 = Bundle By Name(cluster=w289, "Position.X"=w287) -> (w286:T18)
            n142 = Bundle By Name(cluster=w288, "Position.X"=w287) -> (w283:T18)
            n143 = Replace Array Subset(array=w282, new element=w286, index=w284) -> (w281:T17)
            n144 = Replace Array Subset(array=w285, new element=w283, index=w284) -> (w280:T17)
            n145 = property on="Channel 1" class="WFGraph (strict)"("CrsrList"=w281) -> ()  [unwired: 2 in, 2 out]
            n146 = property on="Channel 3" class="WFGraph (strict)"("CrsrList"=w280) -> ()  [unwired: 2 in, 2 out]
          }
          event "Channel 3": Cursor Move {
            n147 = event-data() -> ("CursIdx"=w297:i32, "CursLoc"=w304:cluster{"X":dbl, "Y":dbl})  [unwired: 1 in, 7 out]
            n148 = Unbundle By Name(w304) -> ("X"=w301:dbl)
            n149 = property on="Channel 1" class="WFGraph (strict)"() -> ("CrsrList"=w300:T17)  [unwired: 2 in, 2 out]
            n150 = property on="Channel 2" class="WFGraph (strict)"() -> ("CrsrList"=w298:T17)  [unwired: 2 in, 2 out]
            n151 = Index Array(array=w300, index=w297) -> (element=w303:T18)
            n152 = Index Array(array=w298, index=w297) -> (element=w302:T18)
            n153 = Bundle By Name(cluster=w303, "Position.X"=w301) -> (w299:T18)
            n154 = Bundle By Name(cluster=w302, "Position.X"=w301) -> (w296:T18)
            n155 = Replace Array Subset(array=w300, new element=w299, index=w297) -> (w295:T17)
            n156 = Replace Array Subset(array=w298, new element=w296, index=w297) -> (w294:T17)
            n157 = property on="Channel 1" class="WFGraph (strict)"("CrsrList"=w295) -> ()  [unwired: 2 in, 2 out]
            n158 = property on="Channel 2" class="WFGraph (strict)"("CrsrList"=w294) -> ()  [unwired: 2 in, 2 out]
          }
          event "Cali&iRF alignment": Mouse Enter {
            n159 = event-data() -> ()  [unwired: 1 in, 4 out]
            n160 = local write "Help"("Click to run system intensity calibration and irf alignment" ("Help")) -> ()
          }
          event "Cali&iRF alignment": Value Change {
            n161 = event-data() -> ("NewVal"=w315:bool)  [unwired: 1 in, 5 out]
            n162 = case shown="False" w315 {
              tunnel: ["UI: Cursor Set >> Busy\nUtility: SetAllChanManualGain\nQueue: Flash\nUtility: Dewelling >> 1500\nUtility: SetAllChanAutoGain\nUI: Cursor Set >> Idle\nUI: Update\nLabJack: ZeroV\nLabJack: 355_PWM_Stop\nLabJack: AB_PWM_Stop\nUtility: Dewelling >> 10\nDigitizer: Abort\nUtility: RestoreDeConChan\nData: parseRunData\nData: irfAlignment\nUI: Update\nUI: ReadyForAquisition" "UI: Update\nUtility: SaveDeconChan\nLabJack: 355_PWM_Start\n/*LabJack: AB_PWM_Start\nDigitizer: Start\nLED: Red\nUI: duringIRFAlign"] -> w316
              tunnel: [FALSE TRUE] -> w312
              frame False {
                n163 = property on="Cali&iRF alignment" class="Bool (strict)"("BoolText.Text"="Done!" ("Boolean Text.Text")) -> ()  [unwired: 2 in, 2 out]
              }
              frame True {
                n164 = property on="Cali&iRF alignment" class="Bool (strict)"("BoolText.Text"="Running" ("Boolean Text.Text"), "Colors [4]"=cluster{u32, u32}[] [{6618880, 6618880}, {16711680, 16711680}]) -> ()  [unwired: 2 in, 2 out]
              }
            }
            n165 = Bundle By Name(cluster=w313, "SysRunning?"=w312) -> (w314:T16)
            n166 = call <vilib>:"Add State(s) to Queue__JKI_lib_State_Machine.vi"("State(s) in Front (\"\")"=w316, "State(s) in (\"\")"=w318) -> ("States Out"=w317:string)  [unwired: 13 in]
          }
          event "Gain 1": Value Change {
            n167 = event-data() -> ()  [unwired: 1 in, 6 out]
            n168 = call "V1FGV.vi"("action"=enum16{"write", "read"}."write", "V1 in"="Gain 1") -> ()  [unwired: 8 in, 2 out]
          }
          event "Gain 2": Value Change {
            n169 = event-data() -> ()  [unwired: 1 in, 6 out]
            n170 = call "V2FGV.vi"("action"=enum16{"write", "read"}."write", "V2 in"="Gain 2") -> ()  [unwired: 8 in, 2 out]
          }
          event "Gain 3": Value Change {
            n171 = event-data() -> ()  [unwired: 1 in, 6 out]
            n172 = call "V3FGV.vi"("action"=enum16{"write", "read"}."write", "V3 in"="Gain 3") -> ()  [unwired: 8 in, 2 out]
          }
          event "Quit": Value Change {
            # "Exit Button Value Change (pressed) Event\n(when pressed.  quite)"
            n173 = event-data() -> ()  [unwired: 1 in, 1 out]
            n174 = call <vilib>:"Add State(s) to Queue__JKI_lib_State_Machine.vi"("State(s) in Front (\"\")"="LED: Off\nMacro: Exit", "State(s) in (\"\")"=w346) -> ("States Out"=w345:string)  [unwired: 13 in]
          }
          event "Show BG": Value Change {
            n175 = event-data() -> ()  [unwired: 1 in, 6 out]
            n176 = call <vilib>:"Add State(s) to Queue__JKI_lib_State_Machine.vi"("State(s) in Front (\"\")"="Data: showBG" ("State(s) in Front (\"\")"), "State(s) in (\"\")"=w349) -> ("States Out"=w348:string)  [unwired: 13 in]
          }
          event "StartButton": Mouse Enter {
            n177 = event-data() -> ()  [unwired: 1 in, 4 out]
            n178 = local write "Help"("Press to start aquisition." ("Help")) -> ()
          }
          event "StartButton": Value Change {
            # "start PWM before acquisition"
            # "Initialize both digitizer aquisition and\n send user event to trigger aquisition loop"
            n179 = event-data() -> ()  [unwired: 1 in, 6 out]
            n180 = Unbundle By Name(w361) -> ("System Status.TCP/IP"=w360:bool)
            n181 = case shown="True" w360 {
              tunnel: ["" "TCP: sendRunNum\nTCP: sendVideoSource\nTCP: startRun"] -> w358
              frame False {
              }
              frame True {
              }
            }
            n182 = local write "StartButton"(FALSE ("StartButton")) -> ()
            n183 = Bundle By Name(cluster=w361, "SysRunning?"=TRUE) -> (w363:T16)
            n184 = call <vilib>:"Add State(s) to Queue__JKI_lib_State_Machine.vi"("State(s) in Front (\"\")"="UI: Update\nLabJack: 355_PWM_Start\n/*LabJack: AB_PWM_Start\nDigitizer: Start\nUI: DuringAquisition\nLED: Red", "State(s) in (\"\")"=w358) -> ("States Out"=w357:string)  [unwired: 13 in]
            n185 = call <vilib>:"Add State(s) to Queue__JKI_lib_State_Machine.vi"("State(s) in Front (\"\")"=w357, "State(s) in (\"\")"=w365) -> ("States Out"=w366:string)  [unwired: 13 in]
          }
          event "StopButton": Mouse Enter {
            n186 = event-data() -> ()  [unwired: 1 in, 4 out]
            n187 = local write "Help"("Press to stop data aquisition." ("Help")) -> ()
          }
          event "StopButton": Value Change {
            # "if system is running, send stop command, if not do nothing."
            # "stop aquisition\nupdate UI"
            n188 = event-data() -> ()  [unwired: 1 in, 6 out]
            n189 = Unbundle By Name(w373) -> ("SysRunning?"=w375:bool, "System Status.TCP/IP"=w378:bool)
            n190 = case shown="True" w375 {
              tunnel: w378 -> [_ w390]
              tunnel: ["" w389] -> w377
              tunnel: w373 -> [w382 w386]
              tunnel: [w382 w385] -> w374
              frame False {
              }
              frame True {
                n191 = case shown="True" w390 {
                  tunnel: ["" "TCP: stopRun"] -> w388
                  frame False {
                  }
                  frame True {
                  }
                }
                n192 = Bundle By Name(cluster=w386, "SysRunning?"=FALSE) -> (w385:T16)
                n193 = call <vilib>:"Add State(s) to Queue__JKI_lib_State_Machine.vi"("State(s) in Front (\"\")"=w388, "State(s) in (\"\")"="UI: Cursor Set >> Busy\nUI: Update\nUI: ReadyForAquisition\nLabJack: 355_PWM_Stop\n/*LabJack: AB_PWM_Stop\nDigitizer: Abort\nData: parseDataMacro\nData: saveRunData\nUI: Cursor Set>>Idle") -> ("States Out"=w389:string)  [unwired: 13 in]
              }
            }
            n194 = local write "StopButton"(FALSE ("StopButton")) -> ()
            n195 = call <vilib>:"Add State(s) to Queue__JKI_lib_State_Machine.vi"("State(s) in Front (\"\")"=w377, "State(s) in (\"\")"=w380) -> ("States Out"=w381:string)  [unwired: 13 in]
          }
          event "Sys Reconfig": Mouse Enter {
            n196 = event-data() -> ()  [unwired: 1 in, 4 out]
            n197 = local write "Help"("Click to reconfig digitizer settings." ("Help")) -> ()
          }
          event "Sys Reconfig": Value Change {
            # "everytime the user change data aquisition setting, need to reinitilize decon engine and realign iRF.\ncheck whether data length has changed, if changed, reinitialize Decon engine\nreset BG ready, need a new BG"
            # "update DAQ FGV"
            n198 = event-data() -> ()  [unwired: 1 in, 6 out]
            n199 = call "SystemConfigEditorV6.vi"("error in"=w407) -> ("error out"=w405:errorcluster, "FLImDAQ out"=w400:T5)  [unwired: 1 in]
            n200 = Unbundle By Name(w403) -> ("FLImDAQ.min record length"=w402:i32)
            n201 = Unbundle By Name(w400) -> ("min record length"=w401:i32)
            n202 = call "FLImDAQ_FGV.vi"(6:enum16{"Write", "Read"}."Write" ("Operation"), "error in (no error)"=w405, "Write data"=w400) -> ("error out"=w404:errorcluster, "Read data"=w399:T5)  [unwired: 7 in]
            n203 = Equal?(x=w402, y=w401) -> (x = y?=w398:bool)
            n204 = case shown="False" w398 {
              tunnel: ["UI: Cursor Set >> Busy\nDigitizer: Config\nDeconEngine: InitializeCh1\nDeconEngine: InitializeCh2\nDeconEngine: InitializeCh3\nUI: CaliAndiRFNotReady\n/*UI iRF not ready\nUI: Update\nUI: Cursor Set >> Idle" "UI: Cursor Set >> Busy\nDigitizer: Config\nUI: Update\nUI: Cursor Set >> Idle"] -> w397
              frame False {
              }
              frame True {
              }
            }
            n205 = Bundle By Name(cluster=w403, "FLImDAQ"=w399) -> (w410:T16)
            n206 = call <vilib>:"Add State(s) to Queue__JKI_lib_State_Machine.vi"("State(s) in Front (\"\")"=w397, "State(s) in (\"\")"=w408) -> ("States Out"=w409:string)  [unwired: 13 in]
          }
          event "System Hardware Connection Status", "StartButton", "StopButton", "355nm Laser toggle", "Aiming beam toggle", "Cali&iRF alignment", "Background", "Sys Reconfig": Mouse Leave {
            n207 = event-data() -> ()  [unwired: 1 in, 4 out]
            n208 = invoke on="Help" class="Str" method="Reinit To Default"() -> ()  [unwired: 3 in, 3 out]
          }
          event "System Hardware Connection Status.Digitizer": Mouse Enter {
            n209 = event-data() -> ()  [unwired: 1 in, 4 out]
            n210 = local write "Help"("Status of hardware connections. TCP/IP is optional." ("Help")) -> ()
          }
          event "TCP Connect": Value Change {
            n211 = event-data() -> ("NewVal"=w420:bool)  [unwired: 1 in, 5 out]
            n212 = case shown="False" w420 {
              tunnel: ["TCP: Close\nUI: Update" ("State(s) in Front (\"\")") "TCP: Initialize\nTCP: SendSettingMacro\nUI: Update" ("State(s) in Front (\"\")")] -> w421
              frame False {
              }
              frame True {
              }
            }
            n213 = call <vilib>:"Add State(s) to Queue__JKI_lib_State_Machine.vi"("State(s) in Front (\"\")"=w421, "State(s) in (\"\")"=w423) -> ("States Out"=w422:string)  [unwired: 13 in]
          }
          event User Event {
            # "if aquisition loop is error out. Stop digitizer, update front panel indicator, stop both laser and parse and save data"
            n214 = event-data() -> ()  [unwired: 1 in, 5 out]
            n215 = property on="StopButton" class="Bool (strict)"("Val(Sgnl)"=TRUE ("Value (Signaling)")) -> ()  [unwired: 2 in, 2 out]
            n216 = call <vilib>:"Add State(s) to Queue__JKI_lib_State_Machine.vi"("State(s) in (\"\")"=w430) -> ("States Out"=w431:string)  [unwired: 14 in]
          }
          event Panel Close? {
            # "Discard the event because we'll close the front panel ourselves in Macro: Exit"
            # "Close Panel button (pressed) Event\n(this executes Macro: Exit to terminate the VI)"
            n217 = event-data() -> ()  [unwired: 1 in, 1 out]
            n218 = event-data("Discard?"=TRUE) -> ()  [unwired: 1 in, 1 out]
            n219 = call <vilib>:"Add State(s) to Queue__JKI_lib_State_Machine.vi"("State(s) in Front (\"\")"="Macro: Exit", "State(s) in (\"\")"=w438) -> ("States Out"=w437:string)  [unwired: 13 in]
          }
          event Timeout {
            # "check system status every 2s"
            n220 = event-data() -> ()  [unwired: 1 in, 1 out]
            n221 = Unbundle By Name(w452) -> ("SlowTimer"=w451:u32, "FastTimer"=w439:u32)
            n222 = Tick Count (ms)() -> (millisecond timer value=w440:u32)
            n223 = Subtract(x=w440, y=w451) -> (x-y=w445:u32)
            n224 = Subtract(x=w440, y=w439) -> (x-y=w441:u32)
            n225 = Greater?(x=w445, y=u32 2000) -> (0:w446:bool)
            n226 = Greater?(x=w441, y=u32 100) -> (0:w443:bool)
            n227 = case shown="True" w446 {
              tunnel: ["" "SystemStatus: SlowSysStatusMacro" ("State(s) in Front (\"\")")] -> w447
              frame False {
              }
              frame True {
              }
            }
            n228 = case shown="True" w443 {
              tunnel: ["" "SystemStatus: FastSysStatusMacro" ("State(s) in Front (\"\")")] -> w442
              frame False {
              }
              frame True {
              }
            }
            n229 = call <vilib>:"Add State(s) to Queue__JKI_lib_State_Machine.vi"("State(s) in Front (\"\")"="LabJack: checkPedal" ("State(s) in Front (\"\")"), "State(s) in (\"\")"=w447, "State(s) at Back (\"\")"=w442) -> ("States Out"=w449:string)  [unwired: 12 in]
            n230 = call <vilib>:"Add State(s) to Queue__JKI_lib_State_Machine.vi"("State(s) in Front (\"\")"=w449, "State(s) in (\"\")"=w454) -> ("States Out"=w455:string)  [unwired: 13 in]
          }
        }
      }
      frame "---------- Data ----------" {
        # "Do not put any code in this frame.\n(It is a separator no-op. You can make a copy of this frame to create a new Data frame)"
        n231 = call <vilib>:"Add State(s) to Queue__JKI_lib_State_Machine.vi"("State(s) in (\"\")"=w464) -> ("States Out"=w463:string)  [unwired: 14 in]
      }
      frame "Data: Initialize" {
        w465 = cluster{"RunID":i8, "BG ID":i8, "Cali ID":i8} {"RunID"=1, "BG ID"=1, "Cali ID"=1}  # IDs
        w466 = refnum<vi> refnum  # LED vi reference
        w467 = path ""  # TempPath
        w468 = T19 {"DataPath"=path "", "BG Path"=path "", "iRFPath"=path "", "CaliPath"=path ""}  # Pathes
        w470 = dbl[] []  # V3
        w471 = dbl[] []  # V2
        w472 = dbl[] []  # V1
        w474 = u32 0  # FastTimer
        w475 = u32 0  # SlowTimer
        w476 = dbl[][] []  # Ch3Data
        w477 = dbl[][] []  # Ch2Data
        w478 = dbl[][] []  # Ch1Data
        w481 = T1 {"Digitizer"=FALSE, "Labjack"=FALSE, "Aiming Beam"=FALSE, "355 Laser"=FALSE, "TCP/IP"=FALSE}  # System Status
        w482 = T20 {"DIO_EF_CLOCK1_DIVISOR"=16, "DIO_EF_CLOCK1_ROLL_VALUE"=25000, "DIO#_EF_INDEX"=0, "DIO#_EF_OPTIONS"=1, "DIO#_EF_CONFIG_A"=6250}  # AB PWM setting
        w483 = T4 {"Ch1 Bias"="TDA11", "Ch2 Bias"="DAC10", "Ch3 Bias"="DAC0", "355 PWM"="FIO0", "AimingBeam PWM"="FIO2", "Laser Ready"="FIO3", "Interlock"="FIO1", "Laser Start/Stop"="FIO1", "Red LED"="FIO1", "Green LED"="FIO1", "Foot Pedal"="DIO15"}  # LJ Pinout
        w484 = 0  # TCP attempt count
        w485 = u32 0  # Laser start tic
        w486 = refnum<k20>[] []  # niTClk sessions
        w487 = u32 0  # Last Trigger
        w488 = T20 {"DIO_EF_CLOCK1_DIVISOR"=16, "DIO_EF_CLOCK1_ROLL_VALUE"=25000, "DIO#_EF_INDEX"=0, "DIO#_EF_OPTIONS"=1, "DIO#_EF_CONFIG_A"=6250}  # 355 PWM setting
        w489 = T21 {"Aiming Beam COM Port"="COM3", "Min Current"=0.0, "Max Current"=63.0, "Default Current"=20.0, 0}  # AB Cluster
        w490 = T22 {"resource name"="", "resource name 2"="", "Channel"=enum."Channel 0", "trigger source"="VAL_EXTERNAL", "trigger level"=0.5, "trigger delay"=1.35e-07, "min sample rate"=12500000000.0, "min record length"=2500, "vertical range"=1.0, "vertical offset"=-0.25, "Waveform to Avg"=2000}  # FLImDAQ
        w491 = FALSE  # SysRunning?
        w479 = path ""  # DefaultPath
        w492 = ""  # CaseID
        w493 = T3 {"Ch1Enable?"=FALSE, "Ch2Enable?"=FALSE, "Ch3Enable?"=FALSE, "Ch1AutoGain?"=FALSE, "Ch2AutoGain?"=FALSE, "Ch3AutoGain?"=FALSE, "AimingBeamEnable?"=FALSE}  # SysConfigCluster
        w494 = T23 {"Current VI Reference"=refnum, "Close Panel on Exit?"=FALSE}  # Core
        # "Initialize the shift-register data, here.\n(data names are defined by what you wire into the bundle function)"
        n232 = Bundle("Core"=w494, "SysConfigCluster"=w493, "System Status"=w481, "IDs"=w465, "CaseID"=w492, "DefaultPath"=w479, "Pathes"=w468, "FLImDAQ"=w490, "SysRunning?"=w491, "AB Cluster"=w489, "LJ Pinout"=w483, "355 PWM setting"=w488, "AB PWM setting"=w482, "Last Trigger"=w487, "niTClk sessions"=w486, "Laser start tic"=w485, "TCP attempt count"=w484, "Ch1Data"=w478, "Ch2Data"=w477, "Ch3Data"=w476, "V1"=w472, "V2"=w471, "V3"=w470, "SlowTimer"=w475, "FastTimer"=w474, "listener ID"=refnum<k5> refnum, "TempPath"=w467, "LED vi reference"=w466) -> (w469:T16)  [unwired: 1 in]
        n233 = call <vilib>:"Add State(s) to Queue__JKI_lib_State_Machine.vi"("State(s) in (\"\")"=w497) -> ("States Out"=w496:string)  [unwired: 14 in]
      }
      frame "Data: parseDataMacro" {
        # "Sometimes it takes some time to parse run data"
        # "Parse data macro.\n(Set curse busy, parse data, then set cursor idle)"
        n234 = call <vilib>:"Add State(s) to Queue__JKI_lib_State_Machine.vi"("State(s) in Front (\"\")"="UI: Cursor Set >> Busy\nData: parseRunData\nUI: Cursor Set >> Idle" ("State(s) in Front (\"\")"), "State(s) in (\"\")"=w503) -> ("States Out"=w502:string)  [unwired: 13 in]
      }
      frame "Data: parseRunData" {
        # "flash queue"
        # "Ch3&4"
        # "Ch1&2"
        # "Flash data from queue and save it in structure\n()"
        n235 = Flush Queue(queue=w526, error in (no error)=w519) -> (remaining elements=w524:cluster{"double data":dbl[][]}[], error out=w517:errorcluster)  [unwired: 1 out]
        n236 = Flush Queue(queue=w520, error in (no error)=w519) -> (remaining elements=w514:cluster{"V1":dbl, "V2":dbl, "V3":dbl}[], error out=w515:errorcluster)  [unwired: 1 out]
        n237 = Flush Queue(queue=w525, error in (no error)=w519) -> (remaining elements=w523:cluster{"double data":dbl[][]}[], error out=w516:errorcluster)  [unwired: 1 out]
        n238 = for {
          tunnel: w523 -> [w536] mode=indexing
          tunnel: [w535] -> w504 mode=concatenating
          n239 = Unbundle By Name(w536) -> ("double data"=w534:dbl[][])
          n240 = call "SeperateChanData.vi"("Input (Ch1&2)"=w534) -> ("Ch1"=w535:dbl[][])  [unwired: 1 out]
        }
        n241 = for {
          tunnel: w514 -> [w533] mode=indexing
          tunnel: [w532] -> w509 mode=indexing
          tunnel: [w531] -> w508 mode=indexing
          tunnel: [w530] -> w507 mode=indexing
          n242 = Unbundle By Name(w533) -> ("V1"=w532:dbl, "V2"=w531:dbl, "V3"=w530:dbl)
        }
        "V1" <- w509
        "V2" <- w508
        "V3" <- w507
        n243 = for {
          tunnel: w524 -> [w540] mode=indexing
          tunnel: [w538] -> w506 mode=concatenating
          tunnel: [w537] -> w505 mode=concatenating
          n244 = Unbundle By Name(w540) -> ("double data"=w539:dbl[][])
          n245 = call "SeperateChanData.vi"("Input (Ch1&2)"=w539) -> ("Ch1"=w538:dbl[][], "Ch2"=w537:dbl[][])
        }
        n246 = Array Size(array=w509) -> (size(s)=→"V1 Size":i32)
        n247 = Array Size(array=w508) -> (size(s)=→"V2 Size":i32)
        n248 = Array Size(array=w507) -> (size(s)=→"V3 Size":i32)
        n249 = Bundle By Name(cluster=w521, "Ch1Data"=w506, "Ch2Data"=w505, "Ch3Data"=w504, "V1"=w509, "V2"=w508, "V3"=w507) -> (w522:T16)
        n250 = Array Size(array=w504) -> (size(s)=→"data Size":i32[])
        n251 = Merge Errors(w517, w516, w515) -> (w518:errorcluster)
        n252 = call <vilib>:"Add State(s) to Queue__JKI_lib_State_Machine.vi"("State(s) in (\"\")"=w529) -> ("States Out"=w528:string)  [unwired: 14 in]
      }
      frame "Data: loadLastUseiRF" {
        # "Load last use iRF.\n()"
        n253 = Unbundle By Name(w545) -> ("TempPath"=w544:path)
        n254 = Build Path(base path=w544, name or relative path="iRF.tdms") -> (appended path=w550:path)
        n255 = TDMS Open(11:w550) -> (0:w548:errorcluster, 3:w549:refnum<k34>)  [unwired: 6 in]
        n256 = TDMS Read(0:w549, 11:w548, 12:dbl[][] []) -> (4:w542:refnum<k34>, 10:w546:dbl[][], 15:w541:errorcluster)  [unwired: 5 in, 3 out]
        n257 = case shown="No Error" w541 {
          tunnel: w546 -> [w558 _]
          tunnel: ["UI: CaliAndiRFLoaded" ("State(s) in Front (\"\")") ""] -> w543
          frame No Error {
            n258 = Index Array(array=w558, index (row)=0) -> (element=w561:dbl[])  [unwired: 1 in]
            n259 = Index Array(array=w558, index (row)=1) -> (element=w560:dbl[])  [unwired: 1 in]
            n260 = Index Array(array=w558, index (row)=2) -> (element=w559:dbl[])  [unwired: 1 in]
            n261 = Bundle(w561, w560, w559) -> (w557:cluster{dbl[], dbl[], dbl[]})  [unwired: 1 in]
            n262 = global write "GlobalVariables.vi" "LastUseiRF"(w557) -> ()
          }
          frame Error {
          }
        }
        n263 = TDMS Close(8:w541, 11:w542) -> ()  [unwired: 2 out]
        n264 = call <vilib>:"Add State(s) to Queue__JKI_lib_State_Machine.vi"("State(s) in Front (\"\")"=w543, "State(s) in (\"\")"=w555) -> ("States Out"=w554:string)  [unwired: 13 in]
      }
      frame "Data: loadLastUseCali" {
        # "Load last use calibration.\n()"
        n265 = Unbundle By Name(w570) -> ("TempPath"=w569:path)
        n266 = Build Path(base path=w569, name or relative path="Calibration.tdms") -> (appended path=w575:path)
        n267 = TDMS Open(11:w575) -> (0:w573:errorcluster, 3:w574:refnum<k34>)  [unwired: 6 in]
        n268 = TDMS Read(0:w574, 11:w573, 12:dbl[][] []) -> (4:w566:refnum<k34>, 10:w571:dbl[][], 15:w567:errorcluster)  [unwired: 5 in, 3 out]
        n269 = TDMS Close(8:w567, 11:w566) -> ()  [unwired: 2 out]
        n270 = case shown="Error .." w567 {
          tunnel: w571 -> [w584 _]
          frame No Error {
            n271 = Index Array(array=w584, index (row)=0) -> (element=w583:dbl[])  [unwired: 1 in]
            n272 = Index Array(array=w584, index (row)=1) -> (element=w582:dbl[])  [unwired: 1 in]
            n273 = Index Array(array=w584, index (row)=2) -> (element=w580:dbl[])  [unwired: 1 in]
            n274 = Bundle(w583, w582, w580) -> (w581:cluster{dbl[], dbl[], dbl[]})  [unwired: 1 in]
            n275 = global write "GlobalVariables.vi" "LastUseCaliData"(w581) -> ()
          }
          frame Error {
          }
        }
        n276 = call <vilib>:"Add State(s) to Queue__JKI_lib_State_Machine.vi"("State(s) in (\"\")"=w579) -> ("States Out"=w578:string)  [unwired: 14 in]
      }
      frame "Data: loadLastUseBG" {
        # "check data size here. If not the same as current setting, return error."
        # "Load last use BG.\n()"
        n277 = Unbundle By Name(w594) -> ("TempPath"=w593:path)
        n278 = Build Path(base path=w593, name or relative path="Background.tdms") -> (appended path=w598:path)
        n279 = TDMS Open(11:w598) -> (0:w596:errorcluster, 3:w597:refnum<k34>)  [unwired: 6 in]
        n280 = TDMS Read(0:w597, 11:w596, 12:dbl[][] []) -> (4:w589:refnum<k34>, 10:w592:dbl[][], 15:w588:errorcluster)  [unwired: 5 in, 3 out]
        n281 = TDMS Close(8:w588, 11:w589) -> ()  [unwired: 2 out]
        n282 = case shown="Error .." w588 {
          tunnel: w592 -> [w604 _]
          tunnel: ["UI: BGLoaded" ("State(s) in Front (\"\")") ""] -> w590
          frame No Error {
            w605 = enum16{"write", "read"}."write" ("action")
            # "If no error, check size match"
            n283 = Index Array(array=w604, index (row)=0) -> (element=w608:dbl[])  [unwired: 1 in]
            n284 = Index Array(array=w604, index (row)=1) -> (element=w607:dbl[])  [unwired: 1 in]
            n285 = Index Array(array=w604, index (row)=2) -> (element=w606:dbl[])  [unwired: 1 in]
            n286 = call "BG3FGV.vi"("action"=w605, "BG1 in"=w606) -> ()  [unwired: 8 in, 2 out]
            n287 = call "BG1FGV.vi"("action"=w605, "BG1 in"=w608) -> ()  [unwired: 8 in, 2 out]
            n288 = call "BG2FGV.vi"("action"=w605, "BG1 in"=w607) -> ()  [unwired: 8 in, 2 out]
          }
          frame Error {
            # "If error set BG all 0, update UI"
          }
        }
        n289 = call <vilib>:"Add State(s) to Queue__JKI_lib_State_Machine.vi"("State(s) in Front (\"\")"=w590, "State(s) in (\"\")"=w602) -> ("States Out"=w601:string)  [unwired: 13 in]
      }
      frame "Data: loadLastUseMacro" {
        # "Load last use BG and Cali and iRF.\n(It is a separator no-op. You can make a copy of this frame to create a new Data frame)"
        n290 = call <vilib>:"Add State(s) to Queue__JKI_lib_State_Machine.vi"("State(s) in Front (\"\")"="Data: loadLastUseBG\nData: loadLastUseCali\nData: loadLastUseiRF" ("State(s) in Front (\"\")"), "State(s) in (\"\")"=w618) -> ("States Out"=w617:string)  [unwired: 13 in]
      }
      frame "Data: saveCalibration" {
        w630 = T11."create or replace" ("operation (0:open)")
        w635 = string[] ["Ch1", "Ch2", "Ch3"] ("channel name(s) in (Untitled)")
        w634 = "Calibration" ("group name in (Untitled)")
        w620 = "Calibration" ("default name")
        # "Average data and save calibration file\n(It is a separator no-op. You can make a copy of this frame to create a new Data frame)"
        n291 = Unbundle By Name(w650) -> ("Ch1Data"=w649:dbl[][], "Ch2Data"=w648:dbl[][], "Ch3Data"=w647:dbl[][], "Pathes.CaliPath"=w622:path, "TempPath"=w642:path, "IDs.Cali ID"=w621:i8)
        n292 = Build Path(base path=w642, name or relative path=w620) -> (appended path=w639:path)
        n293 = Format Value(string ("")=w620, format string="%02d", value (0)=w621) -> (output string=w625:string)
        n294 = call "AvgArray.vi"("2D array"=w649) -> ("1D Avg"=w629:dbl[])  [unwired: 10 in]
        n295 = call "AvgArray.vi"("2D array"=w648) -> ("1D Avg"=w628:dbl[])  [unwired: 10 in]
        n296 = call "AvgArray.vi"("2D array"=w647) -> ("1D Avg"=w627:dbl[])  [unwired: 10 in]
        n297 = Build Path(base path=w622, name or relative path=w625) -> (appended path=w623:path)
        n298 = TDMS Open(8:w619, 10:w630, 11:w639) -> (0:w641:errorcluster, 3:w638:refnum<k34>)  [unwired: 4 in]
        n299 = TDMS Open(8:w619, 10:w630, 11:w623) -> (0:w645:errorcluster, 3:w646:refnum<k34>)  [unwired: 4 in]
        n300 = Build Array(w629, w628, w627) -> (w636:dbl[][])
        n301 = Bundle("1D Avg"=w629, "1D Avg"=w628, "1D Avg"=w627) -> (w626:T24)  [unwired: 1 in]
        n302 = TDMS Write(0:w638, 5:w634, 7:w635, 9:w636, 11:w641) -> (4:w637:refnum<k34>, 15:w640:errorcluster)  [unwired: 1 in, 2 out]
        n303 = TDMS Write(0:w646, 5:w634, 7:w635, 9:w636, 11:w645) -> (4:w644:refnum<k34>, 15:w643:errorcluster)  [unwired: 1 in, 2 out]
        n304 = global write "GlobalVariables.vi" "LastUseCaliData"(w626) -> ()
        n305 = TDMS Close(8:w640, 11:w637) -> (0:w632:errorcluster)  [unwired: 1 out]
        n306 = TDMS Close(8:w643, 11:w644) -> (0:w633:errorcluster)  [unwired: 1 out]
        n307 = Merge Errors(w633, w632) -> (w631:errorcluster)
        n308 = call <vilib>:"Add State(s) to Queue__JKI_lib_State_Machine.vi"("State(s) in (\"\")"=w653) -> ("States Out"=w652:string)  [unwired: 14 in]
      }
      frame "Data: saveiRF" {
        w678 = enum16{"write", "read"}."read" ("action")
        # "Get iRF from decon stracture and save it on disk.\n(It is a separator no-op. You can make a copy of this frame to create a new Data frame)"
        n309 = Unbundle By Name(w671) -> ("TempPath"=w670:path)
        n310 = call "Ch1DeconEngineFGV.vi"("action"=w678) -> ("Error Out"=w676:errorcluster, "Ch1DeconEngine out"=w677:refnum<class "LaguerreDeconEngineClass.lvclass">)  [unwired: 9 in]
        n311 = call "Ch2DeconEngineFGV.vi"("action"=w678) -> ("Error Out"=w674:errorcluster, "Ch2DeconEngine out"=w675:refnum<class "LaguerreDeconEngineClass.lvclass">)  [unwired: 9 in]
        n312 = call "Ch3DeconEngineFGV.vi"("action"=w678) -> ("Error Out"=w672:errorcluster, "Ch3DeconEngine out"=w673:refnum<class "LaguerreDeconEngineClass.lvclass">)  [unwired: 9 in]
        n313 = Build Path(base path=w670, name or relative path="iRF" ("default name")) -> (appended path=w668:path)
        n314 = call "getIRF.vi"("error in (no error)"=w676, "LaguerreDeconEngineClass in"=w677) -> ("iRF"=w657:dbl[])  [unwired: 7 in, 2 out]
        n315 = call "getIRF.vi"("error in (no error)"=w674, "LaguerreDeconEngineClass in"=w675) -> ("iRF"=w656:dbl[])  [unwired: 7 in, 2 out]
        n316 = call "getIRF.vi"("error in (no error)"=w672, "LaguerreDeconEngineClass in"=w673) -> ("iRF"=w655:dbl[])  [unwired: 7 in, 2 out]
        n317 = Build Array(w657, w656, w655) -> (w663:dbl[][])
        n318 = TDMS Open(8:w667, 10:T11."create or replace" ("operation (0:open)"), 11:w668) -> (0:w664:errorcluster, 3:w665:refnum<k34>)  [unwired: 4 in]
        n319 = Bundle("iRF"=w657, "iRF"=w656, "iRF"=w655) -> (w654:cluster{"iRF":dbl[], "iRF":dbl[], "iRF":dbl[]})  [unwired: 1 in]
        n320 = global write "GlobalVariables.vi" "LastUseiRF"(w654) -> ()
        n321 = TDMS Write(0:w665, 5:"iRF" ("group name in (Untitled)"), 7:string[] ["Ch1", "Ch2", "Ch3"] ("channel name(s) in (Untitled)"), 9:w663, 11:w664) -> (4:w660:refnum<k34>, 15:w659:errorcluster)  [unwired: 1 in, 2 out]
        n322 = TDMS Close(8:w659, 11:w660) -> (0:w658:errorcluster)  [unwired: 1 out]
        n323 = call <vilib>:"Add State(s) to Queue__JKI_lib_State_Machine.vi"("State(s) in (\"\")"=w681) -> ("States Out"=w680:string)  [unwired: 14 in]
      }
      frame "Data: saveBG" {
        w687 = "Background" ("name or relative path")
        w697 = T11."create or replace" ("operation (0:open)")
        w692 = string[] ["Ch1", "Ch2", "Ch3"] ("channel name(s) in (Untitled)")
        w690 = "Background" ("group name in (Untitled)")
        w710 = enum16{"write", "read"}."write" ("action")
        # "Save BG and pass it to FGV.\n(save BG to disk and set it to FGV)"
        n324 = Unbundle By Name(w713) -> ("Ch1Data"=w712:dbl[][], "Ch2Data"=w711:dbl[][], "Ch3Data"=w709:dbl[][], "Pathes.BG Path"=w682:path, "TempPath"=w685:path, "IDs.BG ID"=w688:i8)
        n325 = Format Value(string ("")=w687, format string="%02d", value (0)=w688) -> (output string=w686:string)
        n326 = Build Path(base path=w682, name or relative path=w686) -> (appended path=w684:path)
        n327 = Build Path(base path=w685, name or relative path=w687) -> (appended path=w693:path)
        n328 = call "AvgArray.vi"("2D array"=w712) -> ("1D Avg"=w706:dbl[])  [unwired: 10 in]
        n329 = call "AvgArray.vi"("2D array"=w711) -> ("1D Avg"=w705:dbl[])  [unwired: 10 in]
        n330 = call "AvgArray.vi"("2D array"=w709) -> ("1D Avg"=w704:dbl[])  [unwired: 10 in]
        n331 = TDMS Open(8:w683, 10:w697, 11:w684) -> (0:w707:errorcluster, 3:w708:refnum<k34>)  [unwired: 4 in]
        n332 = call "BG1FGV.vi"("action"=w710, "BG1 in"=w706) -> ()  [unwired: 8 in, 2 out]
        n333 = call "BG2FGV.vi"("action"=w710, "BG1 in"=w705) -> ()  [unwired: 8 in, 2 out]
        n334 = call "BG3FGV.vi"("action"=w710, "BG1 in"=w704) -> ()  [unwired: 8 in, 2 out]
        n335 = TDMS Open(8:w683, 10:w697, 11:w693) -> (0:w700:errorcluster, 3:w701:refnum<k34>)  [unwired: 4 in]
        n336 = Build Array(w706, w705, w704) -> (w691:dbl[][])
        n337 = TDMS Write(0:w708, 5:w690, 7:w692, 9:w691, 11:w707) -> (4:w703:refnum<k34>, 15:w702:errorcluster)  [unwired: 1 in, 2 out]
        n338 = TDMS Write(0:w701, 5:w690, 7:w692, 9:w691, 11:w700) -> (4:w699:refnum<k34>, 15:w698:errorcluster)  [unwired: 1 in, 2 out]
        n339 = TDMS Close(8:w702, 11:w703) -> (0:w696:errorcluster)  [unwired: 1 out]
        n340 = TDMS Close(8:w698, 11:w699) -> (0:w695:errorcluster)  [unwired: 1 out]
        n341 = Merge Errors(w696, w695) -> (w694:errorcluster)
        n342 = call <vilib>:"Add State(s) to Queue__JKI_lib_State_Machine.vi"("State(s) in (\"\")"=w716) -> ("States Out"=w715:string)  [unwired: 14 in]
      }
      frame "Data: showBG" {
        # "Show BG in seperate window.\n()"
        n343 = call "showBG.vi"() -> ()  [unwired: 12 in]
        n344 = call <vilib>:"Add State(s) to Queue__JKI_lib_State_Machine.vi"("State(s) in (\"\")"=w721) -> ("States Out"=w720:string)  [unwired: 14 in]
      }
      frame "Data: irfAlignment" {
        w768 = enum16{"write", "read"}."write" ("action")
        w782 = enum16{"write", "read"}."read" ("action")
        # "do iRF alignment in this state\n(It is a separator no-op. You can make a copy of this frame to create a new Data frame)"
        n345 = Unbundle By Name(w746) -> ("Ch1Data"=w785:dbl[][], "Ch2Data"=w784:dbl[][], "Ch3Data"=w783:dbl[][])
        n346 = call "Ch3DeconEngineFGV.vi"("Error In"=w781, "action"=w782) -> ("Error Out"=w775:errorcluster, "Ch3DeconEngine out"=w776:refnum<class "LaguerreDeconEngineClass.lvclass">)  [unwired: 8 in]
        n347 = call "Ch1DeconEngineFGV.vi"("Error In"=w781, "action"=w782) -> ("Error Out"=w779:errorcluster, "Ch1DeconEngine out"=w780:refnum<class "LaguerreDeconEngineClass.lvclass">)  [unwired: 8 in]
        n348 = call "Ch2DeconEngineFGV.vi"("Error In"=w781, "action"=w782) -> ("Error Out"=w777:errorcluster, "Ch2DeconEngine out"=w778:refnum<class "LaguerreDeconEngineClass.lvclass">)  [unwired: 8 in]
        n349 = call "AvgArray.vi"("2D array"=w783) -> ("1D Avg"=w722:dbl[])  [unwired: 10 in]
        n350 = call "AvgArray.vi"("2D array"=w784) -> ("1D Avg"=w723:dbl[])  [unwired: 10 in]
        n351 = call "AvgArray.vi"("2D array"=w785) -> ("1D Avg"=w724:dbl[])  [unwired: 10 in]
        n352 = call "RemoveDCBG.vi"("WF in"=w722) -> ("DC"=w727:dbl, "WF out"=w734:dbl[])  [unwired: 8 in, 1 out]
        n353 = call "RemoveDCBG.vi"("WF in"=w723) -> ("DC"=w729:dbl, "WF out"=w735:dbl[])  [unwired: 8 in, 1 out]
        n354 = call "RemoveDCBG.vi"("WF in"=w724) -> ("DC"=w732:dbl, "WF out"=w736:dbl[])  [unwired: 8 in, 1 out]
        n355 = call "computeIRFAlignment.vi"("error in (no error)"=w775, "fIRF temp"=w734, "LaguerreDeconEngineClass in"=w776) -> ("error out"=w773:errorcluster, "LaguerreDeconEngineClass out"=w774:refnum<class "LaguerreDeconEngineClass.lvclass">)  [unwired: 6 in, 1 out]
        n356 = call "computeIRFAlignment.vi"("error in (no error)"=w777, "fIRF temp"=w735, "LaguerreDeconEngineClass in"=w778) -> ("error out"=w769:errorcluster, "LaguerreDeconEngineClass out"=w770:refnum<class "LaguerreDeconEngineClass.lvclass">)  [unwired: 6 in, 1 out]
        n357 = call "computeIRFAlignment.vi"("error in (no error)"=w779, "fIRF temp"=w736, "LaguerreDeconEngineClass in"=w780) -> ("error out"=w771:errorcluster, "LaguerreDeconEngineClass out"=w772:refnum<class "LaguerreDeconEngineClass.lvclass">)  [unwired: 6 in, 1 out]
        n358 = call "Ch1DeconEngineFGV.vi"("Error In"=w771, "action"=w768, "Ch1DeconEngine in"=w772) -> ("Error Out"=w766:errorcluster, "Ch1DeconEngine out"=w767:refnum<class "LaguerreDeconEngineClass.lvclass">)  [unwired: 7 in]
        n359 = call "Ch2DeconEngineFGV.vi"("Error In"=w769, "action"=w768, "Ch2DeconEngine in"=w770) -> ("Error Out"=w756:errorcluster, "Ch2DeconEngine out"=w757:refnum<class "LaguerreDeconEngineClass.lvclass">)  [unwired: 7 in]
        n360 = call "Ch3DeconEngineFGV.vi"("Error In"=w773, "action"=w768, "Ch3DeconEngine in"=w774) -> ("Error Out"=w750:errorcluster, "Ch3DeconEngine out"=w751:refnum<class "LaguerreDeconEngineClass.lvclass">)  [unwired: 7 in]
        n361 = call "setfIRF.vi"("error in (no error)"=w750, "fIRF"=w734, "LaguerreDeconEngineClass in"=w751) -> ("error out"=w754:errorcluster, "LaguerreDeconEngineClass out"=w755:refnum<class "LaguerreDeconEngineClass.lvclass">)  [unwired: 7 in]
        n362 = call "setfIRF.vi"("error in (no error)"=w756, "fIRF"=w735, "LaguerreDeconEngineClass in"=w757) -> ("error out"=w760:errorcluster, "LaguerreDeconEngineClass out"=w761:refnum<class "LaguerreDeconEngineClass.lvclass">)  [unwired: 7 in]
        n363 = call "setfIRF.vi"("error in (no error)"=w766, "fIRF"=w736, "LaguerreDeconEngineClass in"=w767) -> ("error out"=w764:errorcluster, "LaguerreDeconEngineClass out"=w765:refnum<class "LaguerreDeconEngineClass.lvclass">)  [unwired: 7 in]
        n364 = call "computeLCs.vi"("error in (no error)"=w754, "LaguerreDeconClass in"=w755) -> ("error out"=w752:errorcluster, "LaguerreDeconClass out"=w753:refnum<class "LaguerreDeconEngineClass.lvclass">)  [unwired: 8 in]
        n365 = call "computeLCs.vi"("error in (no error)"=w760, "LaguerreDeconClass in"=w761) -> ("error out"=w758:errorcluster, "LaguerreDeconClass out"=w759:refnum<class "LaguerreDeconEngineClass.lvclass">)  [unwired: 8 in]
        n366 = call "computeLCs.vi"("error in (no error)"=w764, "LaguerreDeconClass in"=w765) -> ("error out"=w762:errorcluster, "LaguerreDeconClass out"=w763:refnum<class "LaguerreDeconEngineClass.lvclass">)  [unwired: 8 in]
        n367 = Unbundle By Name(w746) -> ("V1"=w745:dbl[], "V2"=w744:dbl[], "V3"=w743:dbl[])
        n368 = call-poly <vilib>:"Mean.vi"("X"=w745) -> ("mean"=w742:dbl)  [unwired: 1 out]
        n369 = call "getFitting.vi"("error in (no error)"=w752, "LaguerreDeconEngineClass in"=w753) -> ("Fitting"=w725:dbl[])  [unwired: 7 in, 2 out]
        n370 = call "getFitting.vi"("error in (no error)"=w758, "LaguerreDeconEngineClass in"=w759) -> ("Fitting"=w728:dbl[])  [unwired: 7 in, 2 out]
        n371 = call "getFitting.vi"("error in (no error)"=w762, "LaguerreDeconEngineClass in"=w763) -> ("Fitting"=w731:dbl[])  [unwired: 7 in, 2 out]
        n372 = Add(x=w732, y=w731) -> (x+y=w733:dbl[])
        n373 = Add(x=w729, y=w728) -> (x+y=w730:dbl[])
        n374 = call-poly <vilib>:"Mean.vi"("X"=w744) -> ("mean"=w741:dbl)  [unwired: 1 out]
        n375 = Add(x=w727, y=w725) -> (x+y=w726:dbl[])
        n376 = Build Array(w724, w733) -> (w749:dbl[][])
        n377 = Build Array(w723, w730) -> (w748:dbl[][])
        n378 = call-poly <vilib>:"Mean.vi"("X"=w743) -> ("mean"=w740:dbl)  [unwired: 1 out]
        n379 = Build Array(w722, w726) -> (w747:dbl[][])
        n380 = Bundle("mean"=w742, "mean"=w741, "mean"=w740) -> (w739:cluster{"mean":dbl, "mean":dbl, "mean":dbl})  [unwired: 1 in]
        n381 = call "Calib_and_iRFAlign_confirm.vi"("Cluster"=w739, "Ch3 Data"=w747, "Ch2 Data"=w748, "Ch1 Data"=w749) -> ("Save?"=w738:bool)  [unwired: 7 in]
        n382 = case shown="True" w738 {
          tunnel: ["" "Data: saveCalibration\nData: saveiRF\nRun: CaliIncrement"] -> w737
          frame False {
          }
          frame True {
          }
        }
        n383 = call <vilib>:"Add State(s) to Queue__JKI_lib_State_Machine.vi"("State(s) in Front (\"\")"=w737, "State(s) in (\"\")"=w788) -> ("States Out"=w787:string)  [unwired: 13 in]
      }
      frame "Data: saveRunData" {
        (unwired) i16 0 ("width (-)")
        # "Save FLIm data to disk.\n(Save to LV tdms file format)"
        n384 = Unbundle By Name(w827) -> ("Pathes.DataPath"=w826:path, "CaseID"=w794:string, "IDs.RunID"=w793:i8, "Ch1Data"=w820:dbl[][], "Ch2Data"=w816:dbl[][], "Ch3Data"=w812:dbl[][], "V1"=w808:dbl[], "V2"=w805:dbl[], "V3"=w803:dbl[])
        n385 = Format Value(string ("")=w794, format string="%02d", value (0)=w793) -> (output string=w791:string)
        n386 = Build Path(base path=w826, name or relative path=w791) -> (appended path=w825:path)
        n387 = TDMS Open(8:w798, 10:T11."open or create" ("operation (0:open)"), 11:w825) -> (0:w822:errorcluster, 3:w823:refnum<k34>)  [unwired: 4 in]
        n388 = TDMS Write(0:w823, 5:"CH1Data" ("group name in (Untitled)"), 9:w820, 11:w822) -> (4:w819:refnum<k34>, 15:w818:errorcluster)  [unwired: 2 in, 2 out]
        n389 = TDMS Write(0:w819, 5:"Ch2Data" ("group name in (Untitled)"), 9:w816, 11:w818) -> (4:w814:refnum<k34>, 15:w813:errorcluster)  [unwired: 2 in, 2 out]
        n390 = TDMS Write(0:w814, 5:"Ch3Data" ("group name in (Untitled)"), 9:w812, 11:w813) -> (4:w811:refnum<k34>, 15:w810:errorcluster)  [unwired: 2 in, 2 out]
        n391 = TDMS Write(0:w811, 5:"Ch1V" ("group name in (Untitled)"), 9:w808, 11:w810) -> (4:w797:refnum<k34>, 15:w807:errorcluster)  [unwired: 2 in, 2 out]
        n392 = TDMS Write(0:w797, 5:"Ch2V" ("group name in (Untitled)"), 9:w805, 11:w807) -> (4:w802:refnum<k34>, 15:w801:errorcluster)  [unwired: 2 in, 2 out]
        n393 = TDMS Write(0:w802, 5:"Ch3V" ("group name in (Untitled)"), 9:w803, 11:w801) -> (4:w800:refnum<k34>, 15:w799:errorcluster)  [unwired: 2 in, 2 out]
        n394 = TDMS Close(8:w799, 11:w800) -> (0:w796:errorcluster)  [unwired: 1 out]
        n395 = case shown="No Error" w796 {
          tunnel: [w831 ""] -> w795
          frame No Error {
            w831 = "Run: Increment"  # Run: Increment
          }
          frame Error {
          }
        }
        n396 = call <vilib>:"Add State(s) to Queue__JKI_lib_State_Machine.vi"("State(s) in Front (\"\")"=w795, "State(s) in (\"\")"=w830) -> ("States Out"=w829:string)  [unwired: 13 in]
      }
      frame "Data: Cleanup" {
        # "Cleanup any data and references, here.\n(this is called automatically, by the Macro: Exit)"
        n397 = Unbundle By Name(w834) -> ("Core.Current VI Reference"=w837:refnum<vi>)
        n398 = Close Reference(reference=w837, error in (no error)=w836) -> (error out=w835:errorcluster)
        n399 = call <vilib>:"Add State(s) to Queue__JKI_lib_State_Machine.vi"("State(s) in (\"\")"=w839) -> ("States Out"=w838:string)  [unwired: 14 in]
      }
      frame "---------- Core ----------" {
        # "Do not put any code in this frame.\n(it is a separator no-op)"
        n400 = call <vilib>:"Add State(s) to Queue__JKI_lib_State_Machine.vi"("State(s) in (\"\")"=w844) -> ("States Out"=w843:string)  [unwired: 14 in]
      }
      frame Default {
        w855 = 42 items=["No error", "Argument error", "Memory is full", "Out of zone", "End of file", "File already open", "Generic file I/O error", "File not found", "File permission error", "Disk is full", "Duplicate path", "Too many files open", "System feature not enabled", "Resource file not found", "Cannot add resource", "Resource not found", "Image not found", "Image memory error", "Pen does not exist", "Config type invalid", "Config token not found", "Config parse error", "Config memory error", "Bad external code format", "Bad external code offset", "External code not present", "Null window", "Destroy window error", "Null menu", "Print aborted", "Bad print record", "Print driver error", "Windows error during printing", "Memory error during printing", "Print dialog error", "Generic print error", "Invalid device refnum", "Device not found", "Device parameter error", "Device unit error", "Cannot open device", "Device call aborted", "Generic error", "Cancelled by user", "Object ID too low", "Object ID too high", "Object not in heap", "Unknown heap", "Unknown object (invalid DefProc)", "Unknown object (DefProc not in table)", "Message out of range", "Invalid (null) method", "Unknown message", "Manager call not supported", "Bad address", "Network operation in progress", "Network operation timed out", "Connection is busy", "Network attribute not supported", "Network error", "Address in use", "System out of memory", "Connection aborted", "Connection refused", "Not connected", "Already connected", "Connection closed", "Initialization error (interapplication manager)", "Bad occurrence", "Wait on unbound occurrence handler", "Occurrence queue overflow", "Datalog type conflict", "Unused", "Unrecognized type (interapplication manager)", "Memory corrupt", "Failed to make temporary DLL", "Old CIN version", "Drag socket not found", "Failed to load drop-object", "Failed to register OLE object", "Failed to release OLE object", "Format specifier type mismatch", "Unknown format specifier", "Too few format specifiers", "Too many format specifiers", "Scan failed", "Newer CIN version", "Error converting to variant", "Runtime menu error", "Password tampered", "Variant attribute not found", "Incompatible variant data type", "Event data is not available", "Event Store is not present", "Occurrence is not found", "Event Queue is not created", "Event info is not available", "Refnum passed is NULL", "Error retrieving Class GUID", "Error retrieving CoClass GUID", "Error retrieving TypeLib GUID.", "Bad built application magic bytes.", "Specific driver is different from the specific driver associated with the Logical Name.", "There is no session opened to the class driver.", "Max Error", "MAX - Error with config objects", "MAX - Error loading configuration", "MAX - Group not supported"]
        # "Current State"
        # "Do not delete, rename, or modify this frame.\n(this is used to capture unhandled states and typos)"
        # "Handle mistyped state name (developer tool)"
        n401 = Format Into String(format string="Software Exception: Unhandled State \"%s\"." ("message"), error in=w851, w846) -> (resulting string=w854:string, error out=w853:errorcluster)  [unwired: 1 in]
        n402 = call <vilib>:"Error Cluster From Error Code.vi"("show call chain? (False)"=TRUE, "error in (no error)"=w853, "error message (\"\")"=w854, "error code (0)"=w855) -> ("error out"=w852:errorcluster)  [unwired: 5 in]
        n403 = call <vilib>:"Add State(s) to Queue__JKI_lib_State_Machine.vi"("State(s) in (\"\")"=w850) -> ("States Out"=w849:string)  [unwired: 14 in]
      }
      frame "Initialize Core Data" {
        # "Build default path based on the location of project"
        # "Do not delete, rename, or modify this frame.\n(this is used to determine panel behavior on exit)"
        # "originally closed?"
        # "exe?"
        # "If panel starts closed or is an EXE, then close it when we exit"
        n404 = call <vilib>:"Application Directory.vi"() -> ("Application Directory"=w857:path)
        n405 = property class="App"() -> ("App.Kind"=w871:T13)  [unwired: 2 in, 2 out]
        n406 = property class="VI"() -> ("FP.State"=w865:T12)  [unwired: 2 in, 2 out]
        n407 = control-ref of="Current VI Reference"() -> (w866:refnum<vi>)
        n408 = Equal?(x=w865, y=T12."Closed" ("Front Panel Window:State")) -> (x = y?=w863:bool)
        n409 = Equal?(x=w871, y=T13."Run Time System" ("Application:Kind")) -> (x = y?=w869:bool)
        n410 = Build Path(base path=w857, name or relative path="Data") -> (appended path=w861:path)
        n411 = Build Path(base path=w857, name or relative path="SystemTemp") -> (appended path=w858:path)
        n412 = Or(x=w863, y=w869) -> (x .or. y?=w867:bool)
        n413 = Bundle By Name(cluster=w868, "Core.Current VI Reference"=w866, "Core.Close Panel on Exit?"=w867, "DefaultPath"=w861, "TempPath"=w858) -> (w873:T16)
        n414 = call <vilib>:"Add State(s) to Queue__JKI_lib_State_Machine.vi"("State(s) in (\"\")"=w875) -> ("States Out"=w874:string)  [unwired: 14 in]
      }
      frame "Error Handler" {
        # "Unhandled Error -- Display it"
        # "Handle any errors here.\nYou can also output any states to clean-up after errors occur"
        # "Clear error"
        n415 = Unbundle By Name(w876) -> ("code"=w878:i32)
        n416 = case shown="5002" w878 {
          tunnel: ["Macro: Exit" w888 w894] -> w877
          tunnel: w876 -> [w884 _ _]
          frame Default {
            w886 = T25 2 items=["no dialog", "OK message", "continue or stop message", "OK message + warnings", "continue/stop + warnings"] ("type of dialog (OK msg:1)")
            n417 = call <vilib>:"General Error Handler.vi"("type of dialog (OK msg:1)"=w886, "error in (no error)"=w884) -> ()  [unwired: 9 in, 5 out]
          }
          frame 5002 {
            n418 = Two Button Dialog(message="Laser interlock open! Please close interlock and try again! ", 1:"Safely Shutdown" ("F button name (\"Cancel\")"), 2:"OK" ("T button name (\"OK\")")) -> (T button?=w889:bool)
            n419 = case shown="False" w889 {
              tunnel: ["Macro: Exit" "355 Laser: CheckControllerStatus"] -> w888
              frame False {
              }
              frame True {
              }
            }
          }
          frame 5001 {
            n420 = Two Button Dialog(message="Unable to connect to imaging computer, do you want to run data aquisiton along? ", 1:"No" ("F button name (\"Cancel\")"), 2:"Yes" ("T button name (\"OK\")")) -> (T button?=w895:bool)
            n421 = case shown="True" w895 {
              tunnel: ["Macro: Exit" ""] -> w894
              frame False {
              }
              frame True {
              }
            }
          }
        }
        n422 = call <vilib>:"Add State(s) to Queue__JKI_lib_State_Machine.vi"("State(s) in Front (\"\")"=w877, "State(s) in (\"\")"=w883) -> ("States Out"=w882:string)  [unwired: 13 in]
      }
      frame "Exit" {
        # "Do not put any code in this frame.\n(No errors that occur here will be handled.)"
        n423 = call <vilib>:"Add State(s) to Queue__JKI_lib_State_Machine.vi"("State(s) in (\"\")"=w906) -> ("States Out"=w905:string)  [unwired: 14 in]
      }
      frame "---------- Macro ----------" {
        # "Do not put any code in this frame.\n(It is a separator no-op. You can make a copy of this frame to create a new Macro frame)"
        n424 = call <vilib>:"Add State(s) to Queue__JKI_lib_State_Machine.vi"("State(s) in (\"\")"=w911) -> ("States Out"=w910:string)  [unwired: 14 in]
      }
      frame "Macro: Initialize" {
        # "load Labjack setting 1st as it contaisn laser pin infortmation"
        # "start laser 1st, need 7.5s for laser to get ready"
        # "Initialization Macro\n(This is called once, when the VI starts)"
        n425 = call <vilib>:"Add State(s) to Queue__JKI_lib_State_Machine.vi"("State(s) in Front (\"\")"="UI: showDisclaimer\nUI: Cursor Set >> Busy\nGraph: AddCursors\nData: Initialize\nInitialize Core Data\nUI: Initialize\nUI: Front Panel State >> Open\nUI: Update\nMacro: LoadSysConfig\nLabJack: Open\nLabJack: SetDefaultSub\nLED: Yellow\nLED: OpenVIRef\nLED: Breath >> True\nUI: Update\n355 Laser: Laser enable/disable\n355 Laser: Dewelling>>500\n355 Laser: CheckControllerStatus\nUI: Update\nLabJack: 355_PWM_Config\n/*LabJack: AB_PWM_Config\n/*TCP: Initialize\n/*TCP: SyncTime\nUI: Update\n", "State(s) in (\"\")"="Digitizer: Initialize\nDigitizer: Config\nUI: Update\n/*AimingBeam: Initialize\n/*AimingBeam: Set Status>>Enable\n/*AimingBeam: Set Current\nUI: Update\n355 Laser: Check Dewelling\nUI: Cursor Set >> Idle\n/*Case: GetID\nUI: Update\n/*TCP: SendSettingMacro\n/*Case: CreatFileStruct\nUI: Update\n/*Data: loadLastUseMacro\n/*DeconEngine: InitilizeMacro\nUI: ReadyForAquisition\nLED: Breath >> False") -> ("States Out"=w912:string)  [unwired: 13 in]
        n426 = call <vilib>:"Add State(s) to Queue__JKI_lib_State_Machine.vi"("State(s) in Front (\"\")"=w912, "State(s) in (\"\")"=w920) -> ("States Out"=w919:string)  [unwired: 13 in]
        "Help" <- "Hover over controls to see help!" ("Help")
      }
      frame "Macro: LoadSysConfig" {
        # "System configuration Macro\n(Load configurations for different component of the system)"
        n427 = call <vilib>:"Add State(s) to Queue__JKI_lib_State_Machine.vi"("State(s) in Front (\"\")"="SysConfig: Load Sys Config\nSysConfig: Load Digitizer Setting\n/*SysConfig: Load AB setting\nSysConfig: Load LJ Pinout\nSysConfig: Load 355 PWM\n/*SysConfig: Load AB PWM", "State(s) in (\"\")"=w926) -> ("States Out"=w925:string)  [unwired: 13 in]
      }
      frame "Macro: Exit" {
        # "close LJ last"
        # "check whether hardware is initilized, if so close, if not do nothing"
        # "Exit Macro, close all hardware\n(This is called once, when the VI exits)"
        n428 = Unbundle By Name(w946) -> ("System Status.TCP/IP"=w934:bool, "System Status.Digitizer"=w942:bool, "System Status.Aiming Beam"=w941:bool, "System Status.355 Laser"=w940:bool, "System Status.Labjack"=w930:bool, "Core.Close Panel on Exit?"=w935:bool)
        n429 = case shown="True" w942 {
          tunnel: ["" "Digitizer: Close"] -> w937
          frame False {
          }
          frame True {
          }
        }
        n430 = case shown="True" w934 {
          tunnel: ["" "TCP: Close"] -> w936
          frame False {
          }
          frame True {
          }
        }
        n431 = case shown="True" w930 {
          tunnel: ["" "LabJack: SetDefaultAndClose"] -> w927
          frame False {
          }
          frame True {
          }
        }
        n432 = case shown="True" w941 {
          tunnel: ["" "AimingBeam: Set Status >> Disable\nAimingBeam: Close"] -> w929
          frame False {
          }
          frame True {
          }
        }
        n433 = case shown="True" w940 {
          tunnel: ["" "355 Laser: Close\n355 Laser: CheckControllerStatus"] -> w928
          frame False {
          }
          frame True {
          }
        }
        n434 = Select(t="UI: Front Panel State >> Close", s=w935, f="") -> (s? t:f=w931:string)
        n435 = call <vilib>:"Add State(s) to Queue__JKI_lib_State_Machine.vi"("State(s) in Front (\"\")"=w936, "State(s) in (\"\")"=w937, "State(s) at Back (\"\")"=w929) -> ("States Out"=w939:string)  [unwired: 12 in]
        n436 = call <vilib>:"Add State(s) to Queue__JKI_lib_State_Machine.vi"("State(s) in Front (\"\")"=w939, "State(s) in (\"\")"=w928, "State(s) at Back (\"\")"=w927) -> ("States Out"=w933:string)  [unwired: 12 in]
        n437 = call <vilib>:"Add State(s) to Queue__JKI_lib_State_Machine.vi"("State(s) in Front (\"\")"=w933, "State(s) in (\"\")"="UI: Update\nUI: Reset\nLED: CloseVIRef\nQueue: Destory\nData: Cleanup\nExit", "State(s) at Back (\"\")"=w931) -> ("States Out"=w943:string)  [unwired: 12 in]
        n438 = call <vilib>:"Add State(s) to Queue__JKI_lib_State_Machine.vi"("State(s) in Front (\"\")"=w943, "State(s) in (\"\")"=w949) -> ("States Out"=w948:string)  [unwired: 13 in]
      }
      frame "---------- AimingBeam ----------" {
        # "Template Separator\n(You can make a copy of, or modify, this frame)"
        n439 = call <vilib>:"Add State(s) to Queue__JKI_lib_State_Machine.vi"("State(s) in (\"\")"=w964) -> ("States Out"=w963:string)  [unwired: 14 in]
      }
      frame "AimingBeam: Initialize" {
        # "set aiming beam button color"
        # "Open COM port for Aiming Beam\n(Require USB connection)"
        n440 = Unbundle By Name(w966) -> ("AB Cluster.Aiming Beam COM Port"=w974:refnum<visa-resource-name>)
        n441 = call-poly "VISA Configure Serial Port"("VISA resource name"=w974, "Enable Termination\nChar (T)"=TRUE ("Enable Termination\nChar (T)"), "baud rate (9600)"=u32 9600, "error in (no error)"=w971) -> ("error out"=w970:errorcluster)  [unwired: 10 in, 1 out]
        n442 = Unbundle By Name(w970) -> ("status"=w969:bool)
        n443 = Not(x=w969) -> (.not. x?=w968:bool)
        n444 = Bundle By Name(cluster=w966, "System Status.Aiming Beam"=w968) -> (w967:T16)
        n445 = call <vilib>:"Add State(s) to Queue__JKI_lib_State_Machine.vi"("State(s) in (\"\")"=w976) -> ("States Out"=w975:string)  [unwired: 14 in]
      }
      frame "AimingBeam: Close" {
        # "Close Aiming Beam COM port\n(Require USB connection to Aiming Beam Laser)"
        n446 = Unbundle By Name(w979) -> ("AB Cluster.Aiming Beam COM Port"=w983:refnum<visa-resource-name>)
        n447 = VISA Close(VISA resource name=w983, error in (no error)=w981) -> (error out=w982:errorcluster)
        n448 = Bundle By Name(cluster=w979, "System Status.Aiming Beam"=FALSE) -> (w980:T16)
        n449 = call <vilib>:"Add State(s) to Queue__JKI_lib_State_Machine.vi"("State(s) in (\"\")"=w985) -> ("States Out"=w984:string)  [unwired: 14 in]
      }
      frame "AimingBeam: Set Current" {
        # "Set Aiming Beam Current\n(You can make a copy of, or modify, this frame)"
        n450 = Unbundle By Name(w1005) -> ("AB Cluster.Aiming Beam COM Port"=w998:refnum<visa-resource-name>, "AB Cluster.Max Current"=w994:dbl, "AB Cluster.Default Current"=w996:dbl, "AB Cluster.Min Current"=w995:dbl)
        n451 = In Range and Coerce(upper limit=w994, x=w996, lower limit=w995) -> (coerced(x)=w991:dbl)  [unwired: 1 out]
        n452 = property on="Aiming beam toggle" class="Bool (strict)"() -> ("Caption.Text"=w986:string)  [unwired: 2 in, 2 out]
        n453 = Number To Fractional String(number=w991, precision (6)=i16 2) -> (F-format string=w999:string)  [unwired: 2 in]
        n454 = Concatenate Strings("slc:", w999, "\r", "\n") -> (w1002:string)
        n455 = Number To Decimal String(number=w991, width (-)=i16 2) -> (decimal integer string=w990:string)
        n456 = VISA Write(VISA resource name=w998, write buffer=w1002, error in (no error)=w993) -> (error out=w997:errorcluster)  [unwired: 2 out]
        n457 = Concatenate Strings(w986, w990, "mA" ("string")) -> (w988:string)
        n458 = property on="Aiming beam toggle" class="Bool (strict)"("Caption.Text"=w988) -> ()  [unwired: 2 in, 2 out]
        n459 = call <vilib>:"Add State(s) to Queue__JKI_lib_State_Machine.vi"("State(s) in (\"\")"=w1007) -> ("States Out"=w1006:string)  [unwired: 14 in]
      }
      frame "AimingBeam: Set Status" {
        # "Enable Aiming Beam\n(Usage: \"AimingBeam: Set >> Enable|Disable\")"
        n460 = Unbundle By Name(w1014) -> ("AB Cluster.Aiming Beam COM Port"=w1011:refnum<visa-resource-name>)
        n461 = case shown="\"Enable\"" w1013 {
          tunnel: [w1017 w1021] -> w1012
          frame "Disable", Default {
            n462 = Concatenate Strings("cof", "\r", "\n") -> (w1017:string)
          }
          frame "Enable" {
            n463 = Concatenate Strings("con", "\r", "\n") -> (w1021:string)
          }
        }
        n464 = VISA Write(VISA resource name=w1011, write buffer=w1012, error in (no error)=w1009) -> (error out=w1010:errorcluster)  [unwired: 2 out]
        n465 = call <vilib>:"Add State(s) to Queue__JKI_lib_State_Machine.vi"("State(s) in (\"\")"=w1016) -> ("States Out"=w1015:string)  [unwired: 14 in]
      }
      frame "AimingBeam: GetPWMStatus" {
        # "Get aiming beam PWM status\n()"
        n466 = Unbundle By Name(w1025) -> ("LJ Pinout.AimingBeam PWM"=w1034:string)
        n467 = call "LabJack_FGV.vi"("Operation(Read)"=enum16{"Write", "Read"}."Read" ("Operation"), "error in (no error)"=w1027) -> ("error out"=w1031:errorcluster, "Read data"=w1032:i32)  [unwired: 8 in]
        n468 = Concatenate Strings(w1034, "_EF_ENABLE" ("string")) -> (w1030:string)
        n469 = call <vilib>:"LJM_eReadName.vi"("Handle In"=w1032, "Name"=w1030, "error in"=w1031) -> ("Value"=w1029:dbl, "error out"=w1026:errorcluster)  [unwired: 10 in, 1 out]
        n470 = Greater Than 0?(x=w1029) -> (x > 0?=w1028:bool)
        n471 = case shown="False" w1028 {
          frame False {
            # "PWM is off\nset color to dark green"
            n472 = local write "Aiming beam toggle"(FALSE ("Aimging beam")) -> ()
          }
          frame True {
            # "PWM is on\nset color to light green"
            n473 = local write "Aiming beam toggle"(TRUE ("Aimging beam")) -> ()
          }
        }
        n474 = call <vilib>:"Add State(s) to Queue__JKI_lib_State_Machine.vi"("State(s) in (\"\")"=w1038) -> ("States Out"=w1037:string)  [unwired: 14 in]
      }
      frame "---------- Case ----------" {
        # "Template Separator\n(You can make a copy of, or modify, this frame)"
        n475 = call <vilib>:"Add State(s) to Queue__JKI_lib_State_Machine.vi"("State(s) in (\"\")"=w1045) -> ("States Out"=w1044:string)  [unwired: 14 in]
      }
      frame "Case: getCaliID" {
        # "Get Calibration file #\n(You can make a copy of, or modify, this frame)"
        n476 = Unbundle By Name(w1047) -> ("Pathes.CaliPath"=w1050:path)
        n477 = call <vilib>:"Recursive File List.vi"("pattern"="*.tdms", "Treat LLBs as Folders?"=FALSE, "Folder Path"=w1050) -> ("All Files in Dir"=w1055:path[])  [unwired: 4 in, 4 out]
        n478 = for {
          tunnel: w1055 -> [w1065] mode=indexing
          tunnel: [w1064] -> w1054 mode=indexing
          tunnel: "Calibration" -> [w1061]
          n479 = Strip Path(path=w1065) -> (name=w1062:string)  [unwired: 1 out]
          n480 = Search and Replace String(input string=w1062, search string=w1061) -> (result string=w1060:string)  [unwired: 6 in, 3 out]
          n481 = Scan From String(format string="%d" ("string"), input string=w1060) -> (output 1=w1064:i32)  [unwired: 3 in, 3 out]
        }
        n482 = Array Max & Min(array=w1054) -> (max value=w1053:i32)  [unwired: 3 out]
        n483 = Increment(x=w1053) -> (x+1=w1046:i32)
        n484 = Bundle By Name(cluster=w1047, "IDs.Cali ID"=w1046) -> (w1048:T16)
        n485 = call <vilib>:"Add State(s) to Queue__JKI_lib_State_Machine.vi"("State(s) in (\"\")"=w1059) -> ("States Out"=w1058:string)  [unwired: 14 in]
      }
      frame "Case: getBGID" {
        # "Get background #\n(You can make a copy of, or modify, this frame)"
        n486 = Unbundle By Name(w1066) -> ("Pathes.BG Path"=w1074:path)
        n487 = call <vilib>:"Recursive File List.vi"("pattern"="*.tdms", "Treat LLBs as Folders?"=FALSE, "Folder Path"=w1074) -> ("All Files in Dir"=w1070:path[])  [unwired: 4 in, 4 out]
        n488 = for {
          tunnel: w1070 -> [w1085] mode=indexing
          tunnel: [w1084] -> w1071 mode=indexing
          tunnel: "Background" ("name or relative path") -> [w1081]
          n489 = Strip Path(path=w1085) -> (name=w1082:string)  [unwired: 1 out]
          n490 = Search and Replace String(input string=w1082, search string=w1081) -> (result string=w1080:string)  [unwired: 6 in, 3 out]
          n491 = Scan From String(format string="%d" ("string"), input string=w1080) -> (output 1=w1084:i32)  [unwired: 3 in, 3 out]
        }
        n492 = Array Max & Min(array=w1071) -> (max value=w1072:i32)  [unwired: 3 out]
        n493 = Increment(x=w1072) -> (x+1=w1068:i32)
        n494 = Bundle By Name(cluster=w1066, "IDs.BG ID"=w1068) -> (w1067:T16)
        n495 = call <vilib>:"Add State(s) to Queue__JKI_lib_State_Machine.vi"("State(s) in (\"\")"=w1079) -> ("States Out"=w1078:string)  [unwired: 14 in]
      }
      frame "Case: getRunID" {
        # "Check folder for run ID\n(You can make a copy of, or modify, this frame)"
        n496 = Unbundle By Name(w1091) -> ("Pathes.DataPath"=w1090:path, "CaseID"=w1086:string)
        n497 = Build Array("Background" ("name or relative path"), "Calibration") -> (w1098:string[])
        n498 = call <vilib>:"Recursive File List.vi"("Folders to Exclude"=w1098, "pattern"="*.tdms", "Treat LLBs as Folders?"=FALSE, "Folder Path"=w1090) -> ("All Files in Dir"=w1087:path[])  [unwired: 3 in, 4 out]
        n499 = for {
          tunnel: w1087 -> [w1108] mode=indexing
          tunnel: [w1107] -> w1094 mode=indexing
          tunnel: w1086 -> [w1104]
          n500 = Strip Path(path=w1108) -> (name=w1105:string)  [unwired: 1 out]
          n501 = Search and Replace String(input string=w1105, search string=w1104) -> (result string=w1103:string)  [unwired: 6 in, 3 out]
          n502 = Scan From String(format string="%d" ("string"), input string=w1103) -> (output 1=w1107:i32)  [unwired: 3 in, 3 out]
        }
        n503 = Array Max & Min(array=w1094) -> (max value=w1095:i32)  [unwired: 3 out]
        n504 = Increment(x=w1095) -> (x+1=w1093:i32)
        n505 = Bundle By Name(cluster=w1091, "IDs.RunID"=w1093) -> (w1092:T16)
        n506 = call <vilib>:"Add State(s) to Queue__JKI_lib_State_Machine.vi"("State(s) in (\"\")"=w1102) -> ("States Out"=w1101:string)  [unwired: 14 in]
      }
      frame "Case: CreatFileStruct" {
        # "Creat case file structure"
        n507 = Unbundle By Name(w1120) -> ("DefaultPath"=w1126:path, "CaseID"=w1111:string)
        n508 = Build Path(base path=w1126, name or relative path=w1111) -> (appended path=w1125:path)
        n509 = call <vilib>:"Check if File or Folder Exists.vi"("error in (no error)"=w1118, "path"=w1125) -> ("error out"=w1122:errorcluster, "file or folder exists?"=w1124:bool, "dup path"=w1123:path)  [unwired: 7 in]
        n510 = case shown="True" w1124 {
          tunnel: w1123 -> [w1143 w1151]
          tunnel: w1122 -> [w1141 w1146]
          tunnel: [w1135 w1151] -> w1116
          tunnel: [w1139 w1153] -> w1119
          tunnel: [u32 1 u32 0] -> w1110
          tunnel: [w1137 w1156] -> w1115
          tunnel: "Background" ("name or relative path") -> [w1136 w1148]
          tunnel: "Calibration" -> [w1134 w1147]
          tunnel: [w1130 w1149] -> w1112
          tunnel: w1111 -> [_ _]
          tunnel: ["" "Case: getRunID\nCase: getBGID\nCase: getCaliID"] -> w1109
          frame False {
            # "Folder not exist. Creat folders."
            n511 = Create Folder(path (use dialog)=w1143, error in=w1141) -> (created path=w1135:path, error out=w1132:errorcluster)  [unwired: 1 in, 1 out]
            n512 = Build Path(base path=w1135, name or relative path=w1134) -> (appended path=w1133:path)
            n513 = Build Path(base path=w1135, name or relative path=w1136) -> (appended path=w1142:path)
            n514 = Create Folder(path (use dialog)=w1142, error in=w1132) -> (created path=w1137:path, error out=w1138:errorcluster)  [unwired: 1 in, 1 out]
            n515 = Create Folder(path (use dialog)=w1133, error in=w1132) -> (created path=w1130:path, error out=w1131:errorcluster)  [unwired: 1 in, 1 out]
            n516 = Merge Errors(w1138, w1131) -> (w1139:errorcluster)
          }
          frame True {
            # "Folder exsit, check file #"
            n517 = Build Path(base path=w1151, name or relative path=w1147) -> (appended path=w1152:path)
            n518 = Build Path(base path=w1151, name or relative path=w1148) -> (appended path=w1157:path)
            n519 = call <vilib>:"Check if File or Folder Exists.vi"("path"=w1152) -> ("file or folder exists?"=w1150:bool, "dup path"=w1149:path)  [unwired: 8 in, 1 out]
            n520 = call <vilib>:"Check if File or Folder Exists.vi"("path"=w1157) -> ("file or folder exists?"=w1155:bool, "dup path"=w1156:path)  [unwired: 8 in, 1 out]
            n521 = And(x=w1155, y=w1150) -> (x .and. y?=w1154:bool)
            n522 = case shown="False" w1154 {
              tunnel: w1146 -> [_ w1159]
              tunnel: [errorcluster {"status"=TRUE, "code"=5003, "source"="File structure error."} ("error out") w1159] -> w1153
              frame False {
              }
              frame True {
              }
            }
          }
        }
        n523 = Bundle By Name(cluster=w1120, "Pathes.DataPath"=w1116, "Pathes.BG Path"=w1115, "Pathes.CaliPath"=w1112, "IDs.RunID"=w1110, "IDs.BG ID"=w1110, "IDs.Cali ID"=w1110) -> (w1121:T16)
        n524 = call <vilib>:"Add State(s) to Queue__JKI_lib_State_Machine.vi"("State(s) in Front (\"\")"=w1109, "State(s) in (\"\")"=w1128) -> ("States Out"=w1127:string)  [unwired: 13 in]
      }
      frame "Case: GetID" {
        # "Template Separator\n(You can make a copy of, or modify, this frame)"
        n525 = call "set_subjectID.vi"() -> ("subject_id"=w1160:string)  [unwired: 10 in]
        n526 = Bundle By Name(cluster=w1162, "CaseID"=w1160) -> (w1163:T16)
        n527 = call <vilib>:"Add State(s) to Queue__JKI_lib_State_Machine.vi"("State(s) in (\"\")"=w1166) -> ("States Out"=w1165:string)  [unwired: 14 in]
      }
      frame "---------- DeconEngine ----------" {
        # "start data aquisition and then set irfAligh to ture and decon channel to 1,2 and 3."
        # "Template Separator\n(You can make a copy of, or modify, this frame)"
        n528 = call <vilib>:"Add State(s) to Queue__JKI_lib_State_Machine.vi"("State(s) in (\"\")"=w1171) -> ("States Out"=w1170:string)  [unwired: 14 in]
      }
      frame "DeconEngine: InitilizeMacro" {
        # "start data aquisition and then set irfAligh to ture and decon channel to 1,2 and 3."
        # "Initilize Decon Engine for all channel\n(You can make a copy of, or modify, this frame)"
        n529 = call <vilib>:"Add State(s) to Queue__JKI_lib_State_Machine.vi"("State(s) in Front (\"\")"="DeconEngine: InitializeCh1\nDeconEngine: InitializeCh2\nDeconEngine: InitializeCh3" ("State(s) in Front (\"\")"), "State(s) in (\"\")"=w1177) -> ("States Out"=w1176:string)  [unwired: 13 in]
      }
      frame "DeconEngine: InitializeCh1" {
        w1202 = refnum<class "LaguerreDeconEngineClass.lvclass"> refnum  # Ch1DeconObj
        # "Initilize Laguerre Deconvolution engine Object\n(You can make a copy of, or modify, this frame)"
        n530 = global read "GlobalVariables.vi" "LastUseiRF"() -> (w1179:T26)
        n531 = call "FLImDAQ_FGV.vi"(6:enum16{"Write", "Read"}."Read" ("Operation"), "error in (no error)"=w1186) -> ("error out"=w1197:errorcluster, "Read data"=w1196:T5)  [unwired: 8 in]
        n532 = call "setLaguerreOrder.vi"("error in (no error)"=w1197, "LaguerreOrder"=u32 12, "LaguerreDeconClass in"=w1202) -> ("error out"=w1199:errorcluster, "LaguerreDeconClass out"=w1200:refnum<class "LaguerreDeconEngineClass.lvclass">)  [unwired: 7 in]
        n533 = Unbundle By Name(w1196) -> ("min record length"=w1195:i32)
        n534 = Unbundle By Name(w1179) -> ("Ch1 iRF"=w1178:dbl[])
        n535 = call "setDataLength.vi"("error in (no error)"=w1199, "dataLength"=w1195, "LaguerreDeconClass in"=w1200) -> ("error out"=w1194:errorcluster, "LaguerreDeconClass out"=w1193:refnum<class "LaguerreDeconEngineClass.lvclass">)  [unwired: 7 in]
        n536 = call "setIRF.vi"("error in (no error)"=w1194, "iRF"=w1178, "LaguerreDeconClass in"=w1193) -> ("error out"=w1191:errorcluster, "LaguerreDeconClass out"=w1192:refnum<class "LaguerreDeconEngineClass.lvclass">)  [unwired: 7 in]
        n537 = call "computeAlpha.vi"("error in (no error)"=w1191, "LaguerreDeconClass in"=w1192) -> ("error out"=w1189:errorcluster, "LaguerreDeconClass out"=w1190:refnum<class "LaguerreDeconEngineClass.lvclass">)  [unwired: 8 in]
        n538 = call "dataInitilize.vi"("error in (no error)"=w1189, "LaguerreDeconClass in"=w1190) -> ("error out"=w1187:errorcluster, "LaguerreDeconClass out"=w1188:refnum<class "LaguerreDeconEngineClass.lvclass">)  [unwired: 8 in]
        n539 = call "computeDeconMatrix.vi"("error in (no error)"=w1187, "LaguerreDeconClass in"=w1188) -> ("error out"=w1183:errorcluster, "LaguerreDeconClass out"=w1185:refnum<class "LaguerreDeconEngineClass.lvclass">)  [unwired: 8 in]
        n540 = call "Ch1DeconEngineFGV.vi"("Error In"=w1183, "action"=enum16{"write", "read"}."write", "Ch1DeconEngine in"=w1185) -> ("Error Out"=w1182:errorcluster)  [unwired: 7 in, 1 out]
        n541 = call <vilib>:"Add State(s) to Queue__JKI_lib_State_Machine.vi"("State(s) in (\"\")"=w1204) -> ("States Out"=w1203:string)  [unwired: 14 in]
      }
      frame "DeconEngine: InitializeCh2" {
        w1229 = refnum<class "LaguerreDeconEngineClass.lvclass"> refnum  # Ch2DeconObj
        # "Initilize Laguerre Deconvolution engine Object\n(You can make a copy of, or modify, this frame)"
        n542 = global read "GlobalVariables.vi" "LastUseiRF"() -> (w1206:T26)
        n543 = call "FLImDAQ_FGV.vi"(6:enum16{"Write", "Read"}."Read" ("Operation"), "error in (no error)"=w1214) -> ("error out"=w1207:errorcluster, "Read data"=w1224:T5)  [unwired: 8 in]
        n544 = call "setLaguerreOrder.vi"("error in (no error)"=w1207, "LaguerreOrder"=u32 12, "LaguerreDeconClass in"=w1229) -> ("error out"=w1226:errorcluster, "LaguerreDeconClass out"=w1227:refnum<class "LaguerreDeconEngineClass.lvclass">)  [unwired: 7 in]
        n545 = Unbundle By Name(w1224) -> ("min record length"=w1223:i32)
        n546 = Unbundle By Name(w1206) -> ("Ch2 iRF"=w1205:dbl[])
        n547 = call "setDataLength.vi"("error in (no error)"=w1226, "dataLength"=w1223, "LaguerreDeconClass in"=w1227) -> ("error out"=w1222:errorcluster, "LaguerreDeconClass out"=w1221:refnum<class "LaguerreDeconEngineClass.lvclass">)  [unwired: 7 in]
        n548 = call "setIRF.vi"("error in (no error)"=w1222, "iRF"=w1205, "LaguerreDeconClass in"=w1221) -> ("error out"=w1219:errorcluster, "LaguerreDeconClass out"=w1220:refnum<class "LaguerreDeconEngineClass.lvclass">)  [unwired: 7 in]
        n549 = call "computeAlpha.vi"("error in (no error)"=w1219, "LaguerreDeconClass in"=w1220) -> ("error out"=w1217:errorcluster, "LaguerreDeconClass out"=w1218:refnum<class "LaguerreDeconEngineClass.lvclass">)  [unwired: 8 in]
        n550 = call "dataInitilize.vi"("error in (no error)"=w1217, "LaguerreDeconClass in"=w1218) -> ("error out"=w1215:errorcluster, "LaguerreDeconClass out"=w1216:refnum<class "LaguerreDeconEngineClass.lvclass">)  [unwired: 8 in]
        n551 = call "computeDeconMatrix.vi"("error in (no error)"=w1215, "LaguerreDeconClass in"=w1216) -> ("error out"=w1211:errorcluster, "LaguerreDeconClass out"=w1213:refnum<class "LaguerreDeconEngineClass.lvclass">)  [unwired: 8 in]
        n552 = call "Ch2DeconEngineFGV.vi"("Error In"=w1211, "action"=enum16{"write", "read"}."write", "Ch2DeconEngine in"=w1213) -> ("Error Out"=w1210:errorcluster)  [unwired: 7 in, 1 out]
        n553 = call <vilib>:"Add State(s) to Queue__JKI_lib_State_Machine.vi"("State(s) in (\"\")"=w1231) -> ("States Out"=w1230:string)  [unwired: 14 in]
      }
      frame "DeconEngine: InitializeCh3" {
        w1256 = refnum<class "LaguerreDeconEngineClass.lvclass"> refnum  # Ch3DeconObj
        # "Initilize Laguerre Deconvolution engine Object\n(You can make a copy of, or modify, this frame)"
        n554 = call "FLImDAQ_FGV.vi"(6:enum16{"Write", "Read"}."Read" ("Operation"), "error in (no error)"=w1240) -> ("error out"=w1251:errorcluster, "Read data"=w1250:T5)  [unwired: 8 in]
        n555 = global read "GlobalVariables.vi" "LastUseiRF"() -> (w1233:T26)
        n556 = call "setLaguerreOrder.vi"("error in (no error)"=w1251, "LaguerreOrder"=u32 12, "LaguerreDeconClass in"=w1256) -> ("error out"=w1253:errorcluster, "LaguerreDeconClass out"=w1254:refnum<class "LaguerreDeconEngineClass.lvclass">)  [unwired: 7 in]
        n557 = Unbundle By Name(w1250) -> ("min record length"=w1249:i32)
        n558 = Unbundle By Name(w1233) -> ("Ch3 iRF"=w1232:dbl[])
        n559 = call "setDataLength.vi"("error in (no error)"=w1253, "dataLength"=w1249, "LaguerreDeconClass in"=w1254) -> ("error out"=w1248:errorcluster, "LaguerreDeconClass out"=w1247:refnum<class "LaguerreDeconEngineClass.lvclass">)  [unwired: 7 in]
        n560 = call "setIRF.vi"("error in (no error)"=w1248, "iRF"=w1232, "LaguerreDeconClass in"=w1247) -> ("error out"=w1245:errorcluster, "LaguerreDeconClass out"=w1246:refnum<class "LaguerreDeconEngineClass.lvclass">)  [unwired: 7 in]
        n561 = call "computeAlpha.vi"("error in (no error)"=w1245, "LaguerreDeconClass in"=w1246) -> ("error out"=w1243:errorcluster, "LaguerreDeconClass out"=w1244:refnum<class "LaguerreDeconEngineClass.lvclass">)  [unwired: 8 in]
        n562 = call "dataInitilize.vi"("error in (no error)"=w1243, "LaguerreDeconClass in"=w1244) -> ("error out"=w1241:errorcluster, "LaguerreDeconClass out"=w1242:refnum<class "LaguerreDeconEngineClass.lvclass">)  [unwired: 8 in]
        n563 = call "computeDeconMatrix.vi"("error in (no error)"=w1241, "LaguerreDeconClass in"=w1242) -> ("error out"=w1237:errorcluster, "LaguerreDeconClass out"=w1239:refnum<class "LaguerreDeconEngineClass.lvclass">)  [unwired: 8 in]
        n564 = call "Ch3DeconEngineFGV.vi"("Error In"=w1237, "action"=enum16{"write", "read"}."write", "Ch3DeconEngine in"=w1239) -> ("Error Out"=w1236:errorcluster)  [unwired: 7 in, 1 out]
        n565 = call <vilib>:"Add State(s) to Queue__JKI_lib_State_Machine.vi"("State(s) in (\"\")"=w1258) -> ("States Out"=w1257:string)  [unwired: 14 in]
      }
      frame "DeconEngine: iRFAlign" {
        # "Template Separator\n(You can make a copy of, or modify, this frame)"
        n566 = call <vilib>:"Add State(s) to Queue__JKI_lib_State_Machine.vi"("State(s) in (\"\")"=w1263) -> ("States Out"=w1262:string)  [unwired: 14 in]
      }
      frame "---------- Digitizer ----------" {
        # "Template Separator\n(You can make a copy of, or modify, this frame)"
        n567 = call <vilib>:"Add State(s) to Queue__JKI_lib_State_Machine.vi"("State(s) in (\"\")"=w1268) -> ("States Out"=w1267:string)  [unwired: 14 in]
      }
      frame "Digitizer: Initialize" {
        # "Initialize digitizer.\nInitialize both digitizer and update status."
        n568 = Unbundle By Name(w1279) -> ("SysConfigCluster.Ch1Enable?"=w1284:bool, "SysConfigCluster.Ch2Enable?"=w1283:bool, "SysConfigCluster.Ch3Enable?"=w1281:bool)
        n569 = call "FLImDAQ_FGV.vi"(6:enum16{"Write", "Read"}."Read" ("Operation"), "error in (no error)"=w1274) -> ("error out"=w1273:errorcluster, "Read data"=w1272:T5)  [unwired: 8 in]
        n570 = property on="Digitizer" class="Bool (strict)"("Blinking"=TRUE) -> ()  [unwired: 2 in, 2 out]
        n571 = Unbundle By Name(w1272) -> ("Digitizer 1"=w1271:refnum<k15>, "Digitizer 2"=w1270:refnum<k15>)
        n572 = Or(x=w1284, y=w1283) -> (x .or. y?=w1282:bool)
        n573 = case shown="True" w1281 {
          tunnel: w1273 -> [w1287 w1289]
          tunnel: [w1287 w1291] -> w1277
          tunnel: w1270 -> [_ w1290]
          frame False {
          }
          frame True {
            n574 = call <instrlib>:"niScope Initialize.vi"("resource name"=w1290, "reset device"=TRUE, "error in"=w1289) -> ("error out"=w1291:errorcluster)  [unwired: 11 in, 1 out]
          }
        }
        n575 = case shown="True" w1282 {
          tunnel: w1273 -> [w1292 w1294]
          tunnel: [w1292 w1296] -> w1278
          tunnel: w1271 -> [_ w1295]
          frame False {
          }
          frame True {
            n576 = call <instrlib>:"niScope Initialize.vi"("resource name"=w1295, "reset device"=TRUE, "error in"=w1294) -> ("error out"=w1296:errorcluster)  [unwired: 11 in, 1 out]
          }
        }
        n577 = Merge Errors(w1278, w1277) -> (w1276:errorcluster)
        n578 = call <vilib>:"Add State(s) to Queue__JKI_lib_State_Machine.vi"("State(s) in (\"\")"=w1286) -> ("States Out"=w1285:string)  [unwired: 14 in]
      }
      frame "Digitizer: Config" {
        # "Synchronize is taking time ~3s."
        # "Config  digitizer\nCall subVi to config digitizer"
        n579 = Unbundle By Name(w1326) -> ("SysConfigCluster.Ch1Enable?"=w1334:bool, "SysConfigCluster.Ch2Enable?"=w1333:bool, "SysConfigCluster.Ch3Enable?"=w1331:bool, "FLImDAQ"=w1328:T22)
        n580 = call "FLImDAQ_FGV.vi"(6:enum16{"Write", "Read"}."Read" ("Operation")) -> ("Read data"=w1316:T5)  [unwired: 9 in, 1 out]
        n581 = Unbundle By Name(w1316) -> ("Digitizer 1"=w1319:refnum<k15>, "Digitizer 2"=w1318:refnum<k15>)
        n582 = property on="Digitizer" class="Bool (strict)"(error in=w1320, "Blinking"=TRUE) -> (error out=w1322:errorcluster)  [unwired: 1 in, 1 out]
        n583 = Or(x=w1334, y=w1333) -> (x .or. y?=w1332:bool)
        n584 = case shown="True" w1332 {
          tunnel: w1328 -> [_ w1347]
          tunnel: w1322 -> [w1343 w1346]
          tunnel: [w1343 w1345] -> w1329
          tunnel: w1319 -> [_ w1344]
          frame False {
          }
          frame True {
            n585 = call "DigitizerConfig.vi"("error in (no error)"=w1346, "FLImDAQ"=w1347, "IVI Refnum in"=w1344) -> ("error out"=w1345:errorcluster)  [unwired: 7 in, 1 out]
          }
        }
        n586 = case shown="True" w1331 {
          tunnel: w1328 -> [_ w1342]
          tunnel: w1329 -> [w1337 w1341]
          tunnel: [w1337 w1340] -> w1302
          tunnel: w1318 -> [_ w1338]
          frame False {
          }
          frame True {
            n587 = call "DigitizerConfig.vi"("Config Trigge(T)r:"=FALSE, "error in (no error)"=w1341, "FLImDAQ"=w1342, "IVI Refnum in"=w1338) -> ("error out"=w1340:errorcluster)  [unwired: 6 in, 1 out]
          }
        }
        n588 = call "Digitizer1_FGV.vi"("error in (no error)"=w1302, "Operation"=enum16{"Write", "Read"}."Read") -> ("error out"=w1313:errorcluster, "Read data"=w1314:refnum<k15>)  [unwired: 8 in]
        n589 = call <instrlib>:"niScope Get Session Reference.vi"("instrument handle"=w1314, "error in"=w1313) -> ("session reference"=w1306:refnum<k20>, "error out"=w1304:errorcluster)  [unwired: 11 in, 1 out]
        n590 = call "Digitizer2_FGV.vi"("error in (no error)"=w1304, "Operation"=enum16{"Write", "Read"}."Read") -> ("error out"=w1310:errorcluster, "Read data"=w1311:refnum<k15>)  [unwired: 8 in]
        n591 = call <instrlib>:"niScope Get Session Reference.vi"("instrument handle"=w1311, "error in"=w1310) -> ("session reference"=w1305:refnum<k20>, "error out"=w1303:errorcluster)  [unwired: 11 in, 1 out]
        n592 = Build Array(w1306, w1305) -> (w1309:refnum<k20>[])
        n593 = call <instrlib>:"niTClk Configure For Homogeneous Triggers.vi"("error in (no error)"=w1303, "sessions"=w1309) -> ("error out"=w1308:errorcluster, "sessions out"=w1307:refnum<k20>[])  [unwired: 8 in]
        n594 = call <instrlib>:"niTClk Synchronize.vi"("error in (no error)"=w1308, "sessions"=w1307) -> ("error out"=w1301:errorcluster, "sessions out"=w1298:refnum<k20>[])  [unwired: 8 in]
        n595 = call <userlib>:"Wait (ms)__ogtk.vi"("error in (no error)"=w1301, "milliseconds to wait"=u32 1500) -> ("error out"=w1300:errorcluster)  [unwired: 8 in, 1 out]
        n596 = Unbundle By Name(w1300) -> ("status"=w1325:bool)
        n597 = Not(x=w1325) -> (.not. x?=w1324:bool)
        n598 = Bundle By Name(cluster=w1326, "System Status.Digitizer"=w1324, "niTClk sessions"=w1298) -> (w1327:T16)
        n599 = property on="Digitizer" class="Bool (strict)"(error in=w1300, "Blinking"=FALSE) -> (error out=w1317:errorcluster)  [unwired: 1 in, 1 out]
        n600 = call <vilib>:"Add State(s) to Queue__JKI_lib_State_Machine.vi"("State(s) in (\"\")"=w1336) -> ("States Out"=w1335:string)  [unwired: 14 in]
      }
      frame "Digitizer: Start" {
        # "send trigger to start acquisition loop"
        # "initilize aquisition"
        # "Template Separator\n(You can make a copy of, or modify, this frame)"
        n601 = Unbundle By Name(w1355) -> ("niTClk sessions"=w1354:refnum<k20>[])
        n602 = call <instrlib>:"niTClk Initiate.vi"("error in (no error)"=w1348, "sessions"=w1354) -> ("error out"=w1350:errorcluster)  [unwired: 8 in, 1 out]
        n603 = Generate User Event(priority (normal)=usereventprio."high priority", user event=w1351, event data cluster=TRUE ("event data"), error in=w1350) -> (error out=w1349:errorcluster)  [unwired: 1 out]
        n604 = call <vilib>:"Add State(s) to Queue__JKI_lib_State_Machine.vi"("State(s) in (\"\")"=w1358) -> ("States Out"=w1357:string)  [unwired: 14 in]
      }
      frame "Digitizer: Abort" {
        # "Template Separator\n(You can make a copy of, or modify, this frame)"
        n605 = call "Digitizer1_FGV.vi"("error in (no error)"=w1362, "Operation"=enum16{"Write", "Read"}."Read") -> ("error out"=w1369:errorcluster, "Read data"=w1366:refnum<k15>)  [unwired: 8 in]
        n606 = call "Digitizer2_FGV.vi"("error in (no error)"=w1362, "Operation"=enum16{"Write", "Read"}."Read") -> ("error out"=w1365:errorcluster, "Read data"=w1367:refnum<k15>)  [unwired: 8 in]
        n607 = Bundle By Name(cluster=w1359, "SysRunning?"=FALSE ("System Status")) -> (w1360:T16)
        n608 = call <instrlib>:"niScope Abort.vi"("instrument handle"=w1366, "error in"=w1369) -> ("error out"=w1371:errorcluster)  [unwired: 12 in, 1 out]
        n609 = call <instrlib>:"niScope Abort.vi"("instrument handle"=w1367, "error in"=w1365) -> ("error out"=w1370:errorcluster)  [unwired: 12 in, 1 out]
        n610 = Merge Errors(w1371, w1370) -> (w1363:errorcluster)
        n611 = call <vilib>:"Add State(s) to Queue__JKI_lib_State_Machine.vi"("State(s) in (\"\")"=w1374) -> ("States Out"=w1373:string)  [unwired: 14 in]
      }
      frame "Digitizer: checkTemp" {
        w1378 = enum16{"Write", "Read"}."Read" ("Operation")
        # "Template Separator\n(You can make a copy of, or modify, this frame)"
        n612 = call "Digitizer1_FGV.vi"("Operation"=w1378) -> ("error out"=w1380:errorcluster, "Read data"=w1381:refnum<k15>)  [unwired: 9 in]
        n613 = call "Digitizer2_FGV.vi"("Operation"=w1378) -> ("error out"=w1376:errorcluster, "Read data"=w1377:refnum<k15>)  [unwired: 9 in]
        n614 = property class="niScope"(reference=w1381, error in=w1380) -> ("Device Temperature"=→"Dig1 Temp":dbl)  [unwired: 2 out]
        n615 = property class="niScope"(reference=w1377, error in=w1376) -> ("Device Temperature"=→"Dig2 Temp":dbl)  [unwired: 2 out]
        n616 = call <vilib>:"Add State(s) to Queue__JKI_lib_State_Machine.vi"("State(s) in (\"\")"=w1386) -> ("States Out"=w1385:string)  [unwired: 14 in]
      }
      frame "Digitizer: Close" {
        # "Close Digitizer"
        n617 = call "Digitizer1_FGV.vi"("error in (no error)"=w1392, "Operation"=enum16{"Write", "Read"}."Read") -> ("error out"=w1394:errorcluster, "Read data"=w1398:refnum<k15>)  [unwired: 8 in]
        n618 = call "Digitizer2_FGV.vi"("error in (no error)"=w1392, "Operation"=enum16{"Write", "Read"}."Read") -> ("error out"=w1393:errorcluster, "Read data"=w1396:refnum<k15>)  [unwired: 8 in]
        n619 = call <instrlib>:"niScope Close.vi"("instrument handle"=w1398, "error in"=w1394) -> ("error out"=w1391:errorcluster)  [unwired: 13 in]
        n620 = call <instrlib>:"niScope Close.vi"("instrument handle"=w1396, "error in"=w1393) -> ("error out"=w1390:errorcluster)  [unwired: 13 in]
        n621 = Merge Errors(w1391, w1390) -> (w1389:errorcluster)
        n622 = Unbundle By Name(w1389) -> ("status"=w1388:bool)
        n623 = Bundle By Name(cluster=w1399, "System Status.Digitizer"=w1388) -> (w1400:T16)
        n624 = call <vilib>:"Add State(s) to Queue__JKI_lib_State_Machine.vi"("State(s) in (\"\")"=w1402) -> ("States Out"=w1401:string)  [unwired: 14 in]
      }
      frame "---------- LabJack ----------" {
        # "Template Separator\n(You can make a copy of, or modify, this frame)"
        n625 = call <vilib>:"Add State(s) to Queue__JKI_lib_State_Machine.vi"("State(s) in (\"\")"=w1407) -> ("States Out"=w1406:string)  [unwired: 14 in]
      }
      frame "LabJack: checkPedal" {
        # "Template Separator\n(You can make a copy of, or modify, this frame)"
        n626 = Unbundle By Name(w1408) -> ("LJ Pinout.Foot Pedal"=w1412:string)
        n627 = call "LabJack_FGV.vi"("Operation(Read)"=enum16{"Write", "Read"}."Read" ("Operation"), "error in (no error)"=w1410) -> ("error out"=w1414:errorcluster, "Read data"=w1415:i32)  [unwired: 8 in]
        n628 = call <vilib>:"LJM_eReadName.vi"("Handle In"=w1415, "Name"=w1412, "error in"=w1414) -> ("Value"=w1413:dbl, "error out"=w1411:errorcluster)  [unwired: 10 in, 1 out]
        n629 = case shown="1" w1413 {
          tunnel: w1408 -> [w1420 w1423]
          tunnel: [w1420 w1421] -> w1409
          frame 0, Default {
          }
          frame 1 {
            # "If Pedal pressed"
            n630 = Tick Count (ms)() -> (millisecond timer value=w1427:u32)
            n631 = Unbundle By Name(w1423) -> ("Last Trigger"=w1422:u32)
            n632 = Subtract(x=w1427, y=w1422) -> (x-y=w1426:u32)
            n633 = Greater Or Equal?(x=w1426, y=u32 2000) -> (x >= y?=w1424:bool)
            n634 = case shown="True" w1424 {
              tunnel: w1423 -> [w1428 w1429]
              tunnel: w1422 -> [_ _]
              tunnel: [w1428 w1430] -> w1421
              frame False {
              }
              frame True {
                n635 = Tick Count (ms)() -> (millisecond timer value=w1431:u32)
                n636 = Unbundle By Name(w1429) -> ("SysRunning?"=w1432:bool)
                n637 = case shown="True" w1432 {
                  frame False {
                    n638 = property on="StartButton" class="Bool (strict)"("Val(Sgnl)"=TRUE ("Value (Signaling)")) -> ()  [unwired: 2 in, 2 out]
                  }
                  frame True {
                    n639 = property on="StopButton" class="Bool (strict)"("Val(Sgnl)"=TRUE ("Value (Signaling)")) -> ()  [unwired: 2 in, 2 out]
                  }
                }
                n640 = Bundle By Name(cluster=w1429, "Last Trigger"=w1431) -> (w1430:T16)
              }
            }
          }
        }
        n641 = call <vilib>:"Add State(s) to Queue__JKI_lib_State_Machine.vi"("State(s) in (\"\")"=w1419) -> ("States Out"=w1418:string)  [unwired: 14 in]
      }
      frame "LabJack: ZeroV" {
        # "set bias to 0"
        # "Zero APD bias\n(You can make a copy of, or modify, this frame)"
        n642 = Unbundle By Name(w1450) -> ("LJ Pinout.Ch1 Bias"=w1455:string, "LJ Pinout.Ch2 Bias"=w1454:string, "LJ Pinout.Ch3 Bias"=w1453:string)
        n643 = call "V1FGV.vi"("Error In"=w1444, "action"=enum16{"write", "read"}."write", "V1 in"=0.0) -> ("Error Out"=w1443:errorcluster, "V1 out"=w1437:dbl)  [unwired: 7 in]
        n644 = Build Array(w1455, w1454, w1453) -> (w1452:string[])
        n645 = local write "Gain 1"(w1437) -> ()
        n646 = call "V2FGV.vi"("Error In"=w1443, "action"=enum16{"write", "read"}."write", "V2 in"=0.0) -> ("Error Out"=w1442:errorcluster, "V2 out"=w1436:dbl)  [unwired: 7 in]
        n647 = call "LabJack_FGV.vi"("Operation(Read)"=enum16{"Write", "Read"}."Read" ("Operation"), "error in (no error)"=w1444) -> ("error out"=w1456:errorcluster, "Read data"=w1457:i32)  [unwired: 8 in]
        n648 = local write "Gain 2"(w1436) -> ()
        n649 = call "V3FGV.vi"("Error In"=w1442, "action"=enum16{"write", "read"}."write", "V3 in"=0.0) -> ("Error Out"=w1439:errorcluster, "V3 out"=w1435:dbl)  [unwired: 7 in]
        n650 = call <vilib>:"LJM_eWriteNames.vi"("Handle In"=w1457, "aNames"=w1452, "aValuesIn"=dbl[] [0.0, 0.0, 0.0], "error in"=w1456) -> ("error out"=w1440:errorcluster)  [unwired: 9 in, 2 out]
        n651 = local write "Gain 3"(w1435) -> ()
        n652 = Merge Errors(w1439, w1440) -> (w1441:errorcluster)
        n653 = call <vilib>:"Add State(s) to Queue__JKI_lib_State_Machine.vi"("State(s) in (\"\")"=w1461) -> ("States Out"=w1460:string)  [unwired: 14 in]
      }
      frame "LabJack: Open" {
        # "Initialize LabJack T7\nEstablish connection and initialize pins"
        n654 = call "LJ_Open.vi"("error in"=w1470) -> ("error out"=w1467:errorcluster, "Success?"=w1468:bool, "Handle Out"=w1464:i32)  [unwired: 8 in]
        n655 = call "LabJack_FGV.vi"("Operation(Read)"=enum16{"Write", "Read"}."Write" ("Operation"), "error in (no error)"=w1467, "Write data"=w1464) -> ("error out"=w1463:errorcluster)  [unwired: 7 in, 1 out]
        n656 = Bundle By Name(cluster=w1465, "System Status.Labjack"=w1468) -> (w1469:T16)
        n657 = call <vilib>:"Add State(s) to Queue__JKI_lib_State_Machine.vi"("State(s) in (\"\")"=w1472) -> ("States Out"=w1471:string)  [unwired: 14 in]
      }
      frame "LabJack: SetDefaultSub" {
        w1492 = "_EF_ENABLE" ("string")
        # "1. Disable PWM\n2. Set all V to 0\n3. Set 355 relay to open\n4. Set LED to off"
        # "read once to set DIO to input"
        # "set all initila V to 0. Set footpedal to input. Set PWM to low. Set laser relay to open. Set LEDs to yellow."
        # "Set Labjack to correct input and output state and initial values"
        n658 = Unbundle By Name(w1489) -> ("LJ Pinout.355 PWM"=w1494:string, "LJ Pinout.AimingBeam PWM"=w1493:string, "LJ Pinout.Ch1 Bias"=w1501:string, "LJ Pinout.Ch2 Bias"=w1507:string, "LJ Pinout.Ch3 Bias"=w1506:string, "LJ Pinout.Laser Start/Stop"=w1505:string, "LJ Pinout.Red LED"=w1504:string, "LJ Pinout.Green LED"=w1503:string)
        n659 = call "V1FGV.vi"("Error In"=w1482, "action"=enum16{"write", "read"}."write", "V1 in"=0.0) -> ("Error Out"=w1483:errorcluster, "V1 out"=w1475:dbl)  [unwired: 7 in]
        n660 = call "LabJack_FGV.vi"("Operation(Read)"=enum16{"Write", "Read"}."Read" ("Operation"), "error in (no error)"=w1482) -> ("error out"=w1497:errorcluster, "Read data"=w1498:i32)  [unwired: 8 in]
        n661 = local write "Gain 1"(w1475) -> ()
        n662 = call "V2FGV.vi"("Error In"=w1483, "action"=enum16{"write", "read"}."write", "V2 in"=0.0) -> ("Error Out"=w1479:errorcluster, "V2 out"=w1474:dbl)  [unwired: 7 in]
        n663 = Concatenate Strings(w1494, w1492) -> (w1491:string)
        n664 = Concatenate Strings(w1493, w1492) -> (w1490:string)
        n665 = local write "Gain 2"(w1474) -> ()
        n666 = call "V3FGV.vi"("Error In"=w1479, "action"=enum16{"write", "read"}."write", "V3 in"=0.0) -> ("Error Out"=w1476:errorcluster, "V3 out"=w1473:dbl)  [unwired: 7 in]
        n667 = Build Array(w1491, w1490, w1501, w1507, w1506, w1505, w1504, w1503) -> (w1502:string[])
        n668 = Unbundle By Name(w1489) -> ("LJ Pinout.Foot Pedal"=w1488:string)
        n669 = local write "Gain 3"(w1473) -> ()
        n670 = call <vilib>:"LJM_eWriteNames.vi"("Handle In"=w1498, "aNames"=w1502, "aValuesIn"=dbl[] [0.0, 0.0, 0.0, 0.0, 0.0, 0.0, 0.0, 0.0], "error in"=w1497) -> ("Handle Out"=w1496:i32, "error out"=w1495:errorcluster)  [unwired: 9 in, 1 out]
        n671 = call <vilib>:"LJM_eReadName.vi"("Handle In"=w1496, "Name"=w1488, "error in"=w1495) -> ("error out"=w1478:errorcluster)  [unwired: 10 in, 2 out]
        n672 = Merge Errors(w1478, w1476) -> (w1477:errorcluster)
        n673 = call <vilib>:"Add State(s) to Queue__JKI_lib_State_Machine.vi"("State(s) in (\"\")"=w1510) -> ("States Out"=w1509:string)  [unwired: 14 in]
      }
      frame "LabJack: FootPedalConfig" {
        # "Setup footPedal\n(You can make a copy of, or modify, this frame)"
        n674 = call "LabJack_FGV.vi"("Operation(Read)"=enum16{"Write", "Read"}."Read" ("Operation"), "error in (no error)"=w1512) -> ("error out"=w1516:errorcluster, "Read data"=w1517:i32)  [unwired: 8 in]
        n675 = call <vilib>:"LJM_eWriteName.vi"("Handle In"=w1517, "Name"="DIO15", "Value"=1.0, "error in"=w1516) -> ("error out"=w1513:errorcluster)  [unwired: 10 in, 1 out]
        n676 = call <vilib>:"Add State(s) to Queue__JKI_lib_State_Machine.vi"("State(s) in (\"\")"=w1521) -> ("States Out"=w1520:string)  [unwired: 14 in]
      }
      frame "LabJack: SetDefaultAndClose" {
        # "Template Separator\n(You can make a copy of, or modify, this frame)"
        n677 = call <vilib>:"Add State(s) to Queue__JKI_lib_State_Machine.vi"("State(s) in Front (\"\")"="LabJack: SetDefaultSub\nLabJack: Close" ("State(s) in Front (\"\")"), "State(s) in (\"\")"=w1527) -> ("States Out"=w1526:string)  [unwired: 13 in]
      }
      frame "LabJack: Close" {
        # "Close LabJack Refnum"
        n678 = call "LabJack_FGV.vi"("Operation(Read)"=enum16{"Write", "Read"}."Read" ("Operation"), "error in (no error)"=w1533) -> ("error out"=w1528:errorcluster, "Read data"=w1529:i32)  [unwired: 8 in]
        n679 = Bundle By Name(cluster=w1531, "System Status.Labjack"=FALSE ("System Status.Gain Control")) -> (w1534:T16)
        n680 = call <vilib>:"LJM_Close.vi"("error in"=w1528, "Handle"=w1529) -> ("error out"=w1536:errorcluster)  [unwired: 9 in]
        n681 = call <vilib>:"Add State(s) to Queue__JKI_lib_State_Machine.vi"("State(s) in (\"\")"=w1538) -> ("States Out"=w1537:string)  [unwired: 14 in]
      }
      frame "LabJack: Interlock enable/disable" {
        w1547 = i8 0  # int8
        # "Interlock enable/disable\n(Usage: \"LabJack: Interlock enable/disable >> 1|0\")"
        n682 = Fract/Exp String To Number(string=w1548, default (0 dbl)=w1547) -> (number=w1544:i8)  [unwired: 2 in, 1 out]
        n683 = Unbundle By Name(w1546) -> ("LJ Pinout.Interlock"=w1545:string)
        n684 = call "LabJack_FGV.vi"("Operation(Read)"=enum16{"Write", "Read"}."Read" ("Operation")) -> ("Read data"=w1542:i32)  [unwired: 9 in, 1 out]
        n685 = call <vilib>:"LJM_eWriteName.vi"("Handle In"=w1542, "Name"=w1545, "Value"=w1544, "error in"=w1543) -> ("error out"=w1540:errorcluster)  [unwired: 10 in, 1 out]
        n686 = call <vilib>:"Add State(s) to Queue__JKI_lib_State_Machine.vi"("State(s) in (\"\")"=w1550) -> ("States Out"=w1549:string)  [unwired: 14 in]
      }
      frame "LabJack: 355_PWM_Config" {
        w1552 = 0.0 ("element")
        w1572 = "DIO_EF_CLOCK1_ENABLE"
        # "Config PWM frequency"
        n687 = Unbundle By Name(w1564) -> ("355 PWM setting.DIO_EF_CLOCK1_DIVISOR"=w1563:i16, "355 PWM setting.DIO_EF_CLOCK1_ROLL_VALUE"=w1562:i32, "355 PWM setting.DIO#_EF_INDEX"=w1559:i16, "355 PWM setting.DIO#_EF_OPTIONS"=w1558:i16, "355 PWM setting.DIO#_EF_CONFIG_A"=w1557:i32)
        n688 = Unbundle By Name(w1564) -> ("LJ Pinout.355 PWM"=w1571:string)
        n689 = Concatenate Strings(w1571, "_EF_ENABLE" ("string")) -> (w1567:string)
        n690 = Concatenate Strings(w1571, "_EF_INDEX") -> (w1570:string)
        n691 = Concatenate Strings(w1571, "_EF_OPTIONS") -> (w1569:string)
        n692 = Concatenate Strings(w1571, "_EF_CONFIG_A") -> (w1568:string)
        n693 = call "LabJack_FGV.vi"("Operation(Read)"=enum16{"Write", "Read"}."Read" ("Operation")) -> ("Read data"=w1565:i32)  [unwired: 9 in, 1 out]
        n694 = Build Array(w1552, w1552, w1563, w1562, 1.0 ("element"), 0.0 ("element"), w1559, w1558, w1557) -> (w1556:dbl[])
        n695 = Build Array("DIO_EF_CLOCK0_ENABLE", w1572, "DIO_EF_CLOCK1_DIVISOR", "DIO_EF_CLOCK1_ROLL_VALUE", w1572, w1567, w1570, w1569, w1568) -> (w1566:string[])
        n696 = call <vilib>:"LJM_eWriteNames.vi"("Handle In"=w1565, "aNames"=w1566, "aValuesIn"=w1556, "error in"=w1554) -> ("error out"=w1555:errorcluster)  [unwired: 9 in, 2 out]
        n697 = call <vilib>:"Add State(s) to Queue__JKI_lib_State_Machine.vi"("State(s) in (\"\")"=w1581) -> ("States Out"=w1580:string)  [unwired: 14 in]
      }
      frame "LabJack: AB_PWM_Config" {
        w1583 = 0.0 ("element")
        w1603 = "DIO_EF_CLOCK2_ENABLE"
        # "Config PWM frequency"
        n698 = Unbundle By Name(w1595) -> ("LJ Pinout.AimingBeam PWM"=w1602:string)
        n699 = Unbundle By Name(w1595) -> ("AB PWM setting.DIO_EF_CLOCK1_DIVISOR"=w1594:i16, "AB PWM setting.DIO_EF_CLOCK1_ROLL_VALUE"=w1593:i32, "AB PWM setting.DIO#_EF_INDEX"=w1590:i16, "AB PWM setting.DIO#_EF_OPTIONS"=w1589:i16, "AB PWM setting.DIO#_EF_CONFIG_A"=w1588:i32)
        n700 = Concatenate Strings(w1602, "_EF_ENABLE" ("string")) -> (w1598:string)
        n701 = Concatenate Strings(w1602, "_EF_INDEX") -> (w1601:string)
        n702 = Concatenate Strings(w1602, "_EF_OPTIONS") -> (w1600:string)
        n703 = Concatenate Strings(w1602, "_EF_CONFIG_A") -> (w1599:string)
        n704 = call "LabJack_FGV.vi"("Operation(Read)"=enum16{"Write", "Read"}."Read" ("Operation")) -> ("Read data"=w1596:i32)  [unwired: 9 in, 1 out]
        n705 = Build Array(w1583, w1583, w1594, w1593, 1.0 ("element"), 0.0 ("element"), w1590, w1589, w1588) -> (w1587:dbl[])
        n706 = Build Array("DIO_EF_CLOCK0_ENABLE", w1603, "DIO_EF_CLOCK2_DIVISOR", "DIO_EF_CLOCK2_ROLL_VALUE", w1603, w1598, w1601, w1600, w1599) -> (w1597:string[])
        n707 = call <vilib>:"LJM_eWriteNames.vi"("Handle In"=w1596, "aNames"=w1597, "aValuesIn"=w1587, "error in"=w1585) -> ("error out"=w1586:errorcluster)  [unwired: 9 in, 2 out]
        n708 = call <vilib>:"Add State(s) to Queue__JKI_lib_State_Machine.vi"("State(s) in (\"\")"=w1612) -> ("States Out"=w1611:string)  [unwired: 14 in]
      }
      frame "LabJack: 355_PWM_Start" {
        # "Template Separator\n(You can make a copy of, or modify, this frame)"
        n709 = Unbundle By Name(w1620) -> ("LJ Pinout.355 PWM"=w1619:string)
        n710 = call "LabJack_FGV.vi"("Operation(Read)"=enum16{"Write", "Read"}."Read" ("Operation"), "error in (no error)"=w1614) -> ("error out"=w1621:errorcluster, "Read data"=w1622:i32)  [unwired: 8 in]
        n711 = Concatenate Strings(w1619, "_EF_ENABLE" ("string")) -> (w1617:string)
        n712 = call <vilib>:"LJM_eWriteName.vi"("Handle In"=w1622, "Name"=w1617, "Value"=1.0, "error in"=w1621) -> ("error out"=w1615:errorcluster)  [unwired: 10 in, 1 out]
        n713 = call <vilib>:"Add State(s) to Queue__JKI_lib_State_Machine.vi"("State(s) in (\"\")"=w1625) -> ("States Out"=w1624:string)  [unwired: 14 in]
      }
      frame "LabJack: AB_PWM_Start" {
        # "Template Separator\n(You can make a copy of, or modify, this frame)"
        n714 = Unbundle By Name(w1633) -> ("LJ Pinout.AimingBeam PWM"=w1632:string)
        n715 = call "LabJack_FGV.vi"("Operation(Read)"=enum16{"Write", "Read"}."Read" ("Operation"), "error in (no error)"=w1627) -> ("error out"=w1634:errorcluster, "Read data"=w1635:i32)  [unwired: 8 in]
        n716 = Concatenate Strings(w1632, "_EF_ENABLE" ("string")) -> (w1630:string)
        n717 = call <vilib>:"LJM_eWriteName.vi"("Handle In"=w1635, "Name"=w1630, "Value"=1.0, "error in"=w1634) -> ("error out"=w1628:errorcluster)  [unwired: 10 in, 1 out]
        n718 = call <vilib>:"Add State(s) to Queue__JKI_lib_State_Machine.vi"("State(s) in (\"\")"=w1638) -> ("States Out"=w1637:string)  [unwired: 14 in]
      }
      frame "LabJack: 355_PWM_Stop" {
        # "Template Separator\n(You can make a copy of, or modify, this frame)"
        n719 = Unbundle By Name(w1644) -> ("LJ Pinout.355 PWM"=w1648:string)
        n720 = call "LabJack_FGV.vi"("Operation(Read)"=enum16{"Write", "Read"}."Read" ("Operation"), "error in (no error)"=w1642) -> ("error out"=w1649:errorcluster, "Read data"=w1640:i32)  [unwired: 8 in]
        n721 = Concatenate Strings(w1648, "_EF_ENABLE" ("string")) -> (w1646:string)
        n722 = call <vilib>:"LJM_eWriteName.vi"("Handle In"=w1640, "Name"=w1646, "Value"=0.0, "error in"=w1649) -> ("error out"=w1643:errorcluster)  [unwired: 10 in, 1 out]
        n723 = local write "355nm Laser toggle"(FALSE ("355nm Laser toggle")) -> ()
        n724 = call <vilib>:"Add State(s) to Queue__JKI_lib_State_Machine.vi"("State(s) in (\"\")"=w1652) -> ("States Out"=w1651:string)  [unwired: 14 in]
      }
      frame "LabJack: AB_PWM_Stop" {
        # "Template Separator\n(You can make a copy of, or modify, this frame)"
        n725 = Unbundle By Name(w1657) -> ("LJ Pinout.AimingBeam PWM"=w1661:string)
        n726 = call "LabJack_FGV.vi"("Operation(Read)"=enum16{"Write", "Read"}."Read" ("Operation"), "error in (no error)"=w1655) -> ("error out"=w1662:errorcluster, "Read data"=w1663:i32)  [unwired: 8 in]
        n727 = Concatenate Strings(w1661, "_EF_ENABLE" ("string")) -> (w1659:string)
        n728 = call <vilib>:"LJM_eWriteName.vi"("Handle In"=w1663, "Name"=w1659, "Value"=0.0, "error in"=w1662) -> ("error out"=w1656:errorcluster)  [unwired: 10 in, 1 out]
        n729 = local write "Aiming beam toggle"(FALSE ("Aiming beam toggle")) -> ()
        n730 = call <vilib>:"Add State(s) to Queue__JKI_lib_State_Machine.vi"("State(s) in (\"\")"=w1666) -> ("States Out"=w1665:string)  [unwired: 14 in]
      }
      frame "---------- LED ----------" {
        # "Template Separator\n(You can make a copy of, or modify, this frame)"
        n731 = call <vilib>:"Add State(s) to Queue__JKI_lib_State_Machine.vi"("State(s) in (\"\")"=w1671) -> ("States Out"=w1670:string)  [unwired: 14 in]
      }
      frame "LED: OpenVIRef" {
        w1677 = path "C:/Users/IntuitiveA/Desktop/V6 APD LV/SubVI/LEDBreath.vi"  # vi path
        # "Template Separator\n(You can make a copy of, or modify, this frame)"
        n732 = Open VI Reference(vi path=w1677, error in (no error)=w1672) -> (vi reference=w1674:refnum<vi>, error out=w1673:errorcluster)  [unwired: 4 in]
        n733 = Bundle By Name(cluster=w1675, "LED vi reference"=w1674) -> (w1676:T16)
        n734 = call <vilib>:"Add State(s) to Queue__JKI_lib_State_Machine.vi"("State(s) in (\"\")"=w1680) -> ("States Out"=w1679:string)  [unwired: 14 in]
      }
      frame "LED: CloseVIRef" {
        # "Template Separator\n(You can make a copy of, or modify, this frame)"
        n735 = Unbundle By Name(w1681) -> ("LED vi reference"=w1682:refnum<vi>)
        n736 = Close Reference(reference=w1682, error in (no error)=w1684) -> (error out=w1683:errorcluster)
        n737 = call <vilib>:"Add State(s) to Queue__JKI_lib_State_Machine.vi"("State(s) in (\"\")"=w1687) -> ("States Out"=w1686:string)  [unwired: 14 in]
      }
      frame "LED: Breath" {
        # "Breath system LED\n(LED: Breath >> True/False)"
        n738 = Unbundle By Name(w1692) -> ("LED vi reference"=w1691:refnum<vi>)
        n739 = case shown="\"False\", Default" w1688 {
          tunnel: w1691 -> [w1700 w1704]
          tunnel: [w1698 w1702] -> w1690
          tunnel: w1689 -> [w1699 w1701]
          frame "False", Default {
            n740 = invoke class="VI" method="Ctrl Val.Set"(reference=w1700, error in=w1699, "Control Name"="Stop", "Value"=TRUE) -> (error out=w1698:errorcluster)  [unwired: 1 in, 4 out]
          }
          frame "True" {
            n741 = invoke class="VI" method="Run VI"(reference=w1704, error in=w1701, "Wait until done"=FALSE ("Wait Until Done"), "Auto Dispose Ref"=FALSE ("Auto Dispose Reference")) -> (error out=w1702:errorcluster)  [unwired: 1 in, 4 out]
          }
        }
        n742 = call <vilib>:"Add State(s) to Queue__JKI_lib_State_Machine.vi"("State(s) in (\"\")"=w1695) -> ("States Out"=w1694:string)  [unwired: 14 in]
      }
      frame "LED: Off" {
        # "set LED to red"
        # "Template Separator\n(You can make a copy of, or modify, this frame)"
        n743 = Unbundle By Name(w1708) -> ("LJ Pinout.Red LED"=w1707:string, "LJ Pinout.Green LED"=w1706:string)
        n744 = call "LabJack_FGV.vi"("Operation(Read)"=enum16{"Write", "Read"}."Read" ("Operation"), "error in (no error)"=w1709) -> ("error out"=w1716:errorcluster, "Read data"=w1715:i32)  [unwired: 8 in]
        n745 = call <vilib>:"LJM_eWriteName.vi"("Handle In"=w1715, "Name"=w1707, "Value"=0.0, "error in"=w1716) -> ("Handle Out"=w1713:i32, "error out"=w1712:errorcluster)  [unwired: 10 in]
        n746 = call <vilib>:"LJM_eWriteName.vi"("Handle In"=w1713, "Name"=w1706, "Value"=0.0, "error in"=w1712) -> ("error out"=w1710:errorcluster)  [unwired: 10 in, 1 out]
        n747 = call <vilib>:"Add State(s) to Queue__JKI_lib_State_Machine.vi"("State(s) in (\"\")"=w1720) -> ("States Out"=w1719:string)  [unwired: 14 in]
      }
      frame "LED: Red" {
        # "set LED to red"
        # "Template Separator\n(You can make a copy of, or modify, this frame)"
        n748 = Unbundle By Name(w1723) -> ("LJ Pinout.Red LED"=w1722:string, "LJ Pinout.Green LED"=w1721:string)
        n749 = call "LabJack_FGV.vi"("Operation(Read)"=enum16{"Write", "Read"}."Read" ("Operation"), "error in (no error)"=w1724) -> ("error out"=w1731:errorcluster, "Read data"=w1730:i32)  [unwired: 8 in]
        n750 = call <vilib>:"LJM_eWriteName.vi"("Handle In"=w1730, "Name"=w1722, "Value"=9.0, "error in"=w1731) -> ("Handle Out"=w1728:i32, "error out"=w1727:errorcluster)  [unwired: 10 in]
        n751 = call <vilib>:"LJM_eWriteName.vi"("Handle In"=w1728, "Name"=w1721, "Value"=0.0, "error in"=w1727) -> ("error out"=w1725:errorcluster)  [unwired: 10 in, 1 out]
        n752 = call <vilib>:"Add State(s) to Queue__JKI_lib_State_Machine.vi"("State(s) in (\"\")"=w1735) -> ("States Out"=w1734:string)  [unwired: 14 in]
      }
      frame "LED: Green" {
        # "set LED to green"
        # "Template Separator\n(You can make a copy of, or modify, this frame)"
        n753 = Unbundle By Name(w1739) -> ("LJ Pinout.Red LED"=w1737:string, "LJ Pinout.Green LED"=w1738:string)
        n754 = call "LabJack_FGV.vi"("Operation(Read)"=enum16{"Write", "Read"}."Read" ("Operation"), "error in (no error)"=w1741) -> ("error out"=w1747:errorcluster, "Read data"=w1746:i32)  [unwired: 8 in]
        n755 = call <vilib>:"LJM_eWriteName.vi"("Handle In"=w1746, "Name"=w1737, "Value"=0.0, "error in"=w1747) -> ("Handle Out"=w1744:i32, "error out"=w1743:errorcluster)  [unwired: 10 in]
        n756 = call <vilib>:"LJM_eWriteName.vi"("Handle In"=w1744, "Name"=w1738, "Value"=9.0, "error in"=w1743) -> ("error out"=w1740:errorcluster)  [unwired: 10 in, 1 out]
        n757 = call <vilib>:"Add State(s) to Queue__JKI_lib_State_Machine.vi"("State(s) in (\"\")"=w1750) -> ("States Out"=w1749:string)  [unwired: 14 in]
      }
      frame "LED: Yellow" {
        # "set LED to yellow"
        # "set LED to yellow\n(You can make a copy of, or modify, this frame)"
        n758 = Unbundle By Name(w1754) -> ("LJ Pinout.Red LED"=w1752:string, "LJ Pinout.Green LED"=w1753:string)
        n759 = call "LabJack_FGV.vi"("Operation(Read)"=enum16{"Write", "Read"}."Read" ("Operation"), "error in (no error)"=w1756) -> ("error out"=w1762:errorcluster, "Read data"=w1761:i32)  [unwired: 8 in]
        n760 = call <vilib>:"LJM_eWriteName.vi"("Handle In"=w1761, "Name"=w1752, "Value"=9.0, "error in"=w1762) -> ("Handle Out"=w1759:i32, "error out"=w1758:errorcluster)  [unwired: 10 in]
        n761 = call <vilib>:"LJM_eWriteName.vi"("Handle In"=w1759, "Name"=w1753, "Value"=9.0, "error in"=w1758) -> ("error out"=w1755:errorcluster)  [unwired: 10 in, 1 out]
        n762 = call <vilib>:"Add State(s) to Queue__JKI_lib_State_Machine.vi"("State(s) in (\"\")"=w1765) -> ("States Out"=w1764:string)  [unwired: 14 in]
      }
      frame "---------- Queue ----------" {
        # "Template Separator\n(You can make a copy of, or modify, this frame)"
        n763 = call <vilib>:"Add State(s) to Queue__JKI_lib_State_Machine.vi"("State(s) in (\"\")"=w1770) -> ("States Out"=w1769:string)  [unwired: 14 in]
      }
      frame "Queue: Create" {
        # "Template Separator\n(You can make a copy of, or modify, this frame)"
        n764 = call <vilib>:"Add State(s) to Queue__JKI_lib_State_Machine.vi"("State(s) in (\"\")"=w1775) -> ("States Out"=w1774:string)  [unwired: 14 in]
      }
      frame "Queue: Flash" {
        # "Clear queue contnet\n(clear queue content by flash it)"
        n765 = Flush Queue(queue=w1779, error in (no error)=w1778) -> (error out=w1777:errorcluster)  [unwired: 2 out]
        n766 = Flush Queue(queue=w1780, error in (no error)=w1777) -> (error out=w1776:errorcluster)  [unwired: 2 out]
        n767 = call <vilib>:"Add State(s) to Queue__JKI_lib_State_Machine.vi"("State(s) in (\"\")"=w1784) -> ("States Out"=w1783:string)  [unwired: 14 in]
      }
      frame "Queue: Destory" {
        # "Destory Data Queue\nDistory data queue ref so the aquisition loop stop"
        n768 = Release Queue(queue=w1790, error in (no error)=w1786) -> (error out=w1793:errorcluster)  [unwired: 1 in, 2 out]
        n769 = Release Queue(queue=w1789, error in (no error)=w1786) -> (error out=w1792:errorcluster)  [unwired: 1 in, 2 out]
        n770 = Release Queue(queue=w1787, error in (no error)=w1786) -> (error out=w1785:errorcluster)  [unwired: 1 in, 2 out]
        n771 = Merge Errors(w1793, w1792, w1785) -> (w1791:errorcluster)
        n772 = call <vilib>:"Simple Error Handler.vi"("error in (no error)"=w1791) -> ()  [unwired: 4 in, 5 out]
        n773 = call <vilib>:"Add State(s) to Queue__JKI_lib_State_Machine.vi"("State(s) in (\"\")"=w1796) -> ("States Out"=w1795:string)  [unwired: 14 in]
      }
      frame "---------- Run ----------" {
        # "Template Separator\n(You can make a copy of, or modify, this frame)"
        n774 = call <vilib>:"Add State(s) to Queue__JKI_lib_State_Machine.vi"("State(s) in (\"\")"=w1801) -> ("States Out"=w1800:string)  [unwired: 14 in]
      }
      frame "Run: CaliIncrement" {
        # "Increment Calibration #\n(You can make a copy of, or modify, this frame)"
        n775 = Unbundle By Name(w1803) -> ("IDs.Cali ID"=w1805:i8)
        n776 = Increment(x=w1805) -> (x+1=w1802:i8)
        n777 = Bundle By Name(cluster=w1803, "IDs.Cali ID"=w1802) -> (w1804:T16)
        n778 = call <vilib>:"Add State(s) to Queue__JKI_lib_State_Machine.vi"("State(s) in (\"\")"=w1809) -> ("States Out"=w1808:string)  [unwired: 14 in]
      }
      frame "Run: BGIncrement" {
        # "Increment BG #\n(You can make a copy of, or modify, this frame)"
        n779 = Unbundle By Name(w1810) -> ("IDs.BG ID"=w1813:i8)
        n780 = Increment(x=w1813) -> (x+1=w1812:i8)
        n781 = Bundle By Name(cluster=w1810, "IDs.BG ID"=w1812) -> (w1811:T16)
        n782 = call <vilib>:"Add State(s) to Queue__JKI_lib_State_Machine.vi"("State(s) in (\"\")"=w1817) -> ("States Out"=w1816:string)  [unwired: 14 in]
      }
      frame "Run: Increment" {
        # "Increase Run# by 1"
        n783 = Unbundle By Name(w1820) -> ("IDs.RunID"=w1822:i8)
        n784 = Increment(x=w1822) -> (x+1=w1819:i8)
        n785 = Bundle By Name(cluster=w1820, "IDs.RunID"=w1819) -> (w1821:T16)
        n786 = call <vilib>:"Add State(s) to Queue__JKI_lib_State_Machine.vi"("State(s) in (\"\")"=w1825) -> ("States Out"=w1824:string)  [unwired: 14 in]
      }
      frame "Run: Decrement" {
        # "Increase Run# by 1"
        n787 = Unbundle By Name(w1828) -> ("IDs.RunID"=w1830:i8)
        n788 = Decrement(x=w1830) -> (x-1=w1827:i8)
        n789 = Bundle By Name(cluster=w1828, "IDs.RunID"=w1827) -> (w1829:T16)
        n790 = call <vilib>:"Add State(s) to Queue__JKI_lib_State_Machine.vi"("State(s) in (\"\")"=w1833) -> ("States Out"=w1832:string)  [unwired: 14 in]
      }
      frame "---------- SysConfig ----------" {
        # "Template Separator\n(You can make a copy of, or modify, this frame)"
        n791 = call <vilib>:"Add State(s) to Queue__JKI_lib_State_Machine.vi"("State(s) in (\"\")"=w1838) -> ("States Out"=w1837:string)  [unwired: 14 in]
      }
      frame "SysConfig: Load Sys Config" {
        # "Load System config"
        # "Load system configuration\n(Load both hardware and DAQ config)"
        n792 = call "LoadSysConfig.vi"("Error In"=w1841, "Enum"=enum16{"LastUse", "Default"}."LastUse") -> ("Error Out"=w1840:errorcluster, "SysConfigCluster"=w1843:T3)  [unwired: 8 in]
        "SysConfigCluster" <- w1843
        n793 = Bundle By Name(cluster=w1844, "SysConfigCluster"=w1843) -> (w1845:T16)
        n794 = call <vilib>:"Add State(s) to Queue__JKI_lib_State_Machine.vi"("State(s) in (\"\")"=w1847) -> ("States Out"=w1846:string)  [unwired: 14 in]
      }
      frame "SysConfig: Load Digitizer Setting" {
        w1854 = enum16{"Write", "Read"}."Write" ("Operation")
        # "Load DAQ config\nSave to FGV"
        # "Template Separator\n(You can make a copy of, or modify, this frame)"
        n795 = call <userlib>:"Current VIs Parent Directory__ogtk.vi"() -> ("Parent Directory (+ Relative)"=w1861:path)  [unwired: 5 in]
        n796 = Build Path(base path=w1861, name or relative path="SubVI\\DigitizerConfiguration\\V6_Scope_last_use.config") -> (appended path=w1862:path)
        n797 = call "ReadDigitizerConfig(SubVI).vi"("error in (no error)"=w1859, "appended path"=w1862) -> ("error out"=w1853:errorcluster, "FLImDAQ"=w1851:T5)  [unwired: 8 in]
        n798 = call "FLImDAQ_FGV.vi"(6:w1854, "error in (no error)"=w1853, "Write data"=w1851) -> ("error out"=w1857:errorcluster)  [unwired: 7 in, 1 out]
        n799 = Bundle By Name(cluster=w1849, "FLImDAQ"=w1851) -> (w1850:T16)
        n800 = Unbundle By Name(w1851) -> ("Digitizer 1"=w1855:refnum<k15>, "Digitizer 2"=w1856:refnum<k15>)
        n801 = call "Digitizer1_FGV.vi"("error in (no error)"=w1857, "Operation"=w1854, "Write data"=w1855) -> ("error out"=w1858:errorcluster)  [unwired: 7 in, 1 out]
        n802 = call "Digitizer2_FGV.vi"("error in (no error)"=w1858, "Operation"=w1854, "Write data"=w1856) -> ("error out"=w1852:errorcluster)  [unwired: 7 in, 1 out]
        n803 = call <vilib>:"Add State(s) to Queue__JKI_lib_State_Machine.vi"("State(s) in (\"\")"=w1864) -> ("States Out"=w1863:string)  [unwired: 14 in]
      }
      frame "SysConfig: Load LJ Pinout" {
        # "Template Separator\n(You can make a copy of, or modify, this frame)"
        n804 = call <userlib>:"Current VIs Parent Directory__ogtk.vi"() -> ("Parent Directory (+ Relative)"=w1878:path)  [unwired: 5 in]
        n805 = Build Path(base path=w1878, name or relative path="SubVI\\LabJack\\LJ_pin_setting.config") -> (appended path=w1876:path)
        n806 = call "ReadLabjackConfig(SubVI).vi"("error in (no error)"=w1874, "appended path"=w1876) -> ("error out"=w1875:errorcluster, "Utility"=w1872:T4)  [unwired: 8 in]
        n807 = Unbundle By Name(w1872) -> ("Ch1 Bias"=w1871:string, "Ch2 Bias"=w1870:string, "Ch3 Bias"=w1869:string, "Red LED"=w1866:string, "Green LED"=w1865:string)
        n808 = global write "GlobalVariables.vi" "LED Green pin"(w1865) -> ()
        n809 = global write "GlobalVariables.vi" "LED Red pin"(w1866) -> ()
        n810 = global write "GlobalVariables.vi" "Ch1 LJ pin"(w1871) -> ()
        n811 = global write "GlobalVariables.vi" "Ch2 LJ pin"(w1870) -> ()
        n812 = global write "GlobalVariables.vi" "Ch3 LJ pin"(w1869) -> ()
        n813 = Bundle By Name(cluster=w1867, "LJ Pinout"=w1872) -> (w1873:T16)
        n814 = call <vilib>:"Add State(s) to Queue__JKI_lib_State_Machine.vi"("State(s) in (\"\")"=w1880) -> ("States Out"=w1879:string)  [unwired: 14 in]
      }
      frame "SysConfig: Load 355 PWM" {
        # "Template Separator\n(You can make a copy of, or modify, this frame)"
        n815 = call <userlib>:"Current VIs Parent Directory__ogtk.vi"() -> ("Parent Directory (+ Relative)"=w1898:path)  [unwired: 5 in]
        n816 = Build Path(base path=w1898, name or relative path="SubVI\\LabJack\\PWM_setting_355.config") -> (appended path=w1896:path)
        n817 = call "ReadPWMConfig(SubVI).vi"("error in (no error)"=w1893, "appended path"=w1896) -> ("error out"=w1894:errorcluster, "PWM Setting"=w1892:T27)  [unwired: 8 in]
        n818 = Unbundle By Name(w1892) -> ("DIO_EF_CLOCK1_DIVISOR"=w1889:i16, "DIO_EF_CLOCK1_ROLL_VALUE"=w1888:i32)
        n819 = Multiply(x=w1889, y=w1888) -> (x*y=w1890:i32)
        n820 = Bundle By Name(cluster=w1895, "355 PWM setting"=w1892) -> (w1882:T16)
        n821 = Divide(x=80000000.0, y=w1890) -> (x/y=w1887:dbl)
        n822 = Number To Decimal String(number=w1887) -> (decimal integer string=w1886:string)  [unwired: 1 in]
        n823 = Concatenate Strings("355nm " ("string"), w1886, "Hz" ("string")) -> (w1884:string)
        n824 = property on="355nm Laser toggle" class="Bool (strict)"("Caption.Text"=w1884) -> ()  [unwired: 2 in, 2 out]
        n825 = call <vilib>:"Add State(s) to Queue__JKI_lib_State_Machine.vi"("State(s) in (\"\")"=w1900) -> ("States Out"=w1899:string)  [unwired: 14 in]
      }
      frame "SysConfig: Load AB PWM" {
        # "Template Separator\n(You can make a copy of, or modify, this frame)"
        n826 = call <userlib>:"Current VIs Parent Directory__ogtk.vi"() -> ("Parent Directory (+ Relative)"=w1919:path)  [unwired: 5 in]
        n827 = Build Path(base path=w1919, name or relative path="SubVI\\LabJack\\PWM_setting_AB.config") -> (appended path=w1917:path)
        n828 = call "ReadPWMConfig(SubVI).vi"("error in (no error)"=w1914, "appended path"=w1917) -> ("error out"=w1915:errorcluster, "PWM Setting"=w1913:T27)  [unwired: 8 in]
        n829 = Unbundle By Name(w1913) -> ("DIO_EF_CLOCK1_DIVISOR"=w1910:i16, "DIO_EF_CLOCK1_ROLL_VALUE"=w1909:i32)
        n830 = Multiply(x=w1910, y=w1909) -> (x*y=w1911:i32)
        n831 = Bundle By Name(cluster=w1903, "AB PWM setting"=w1913) -> (w1916:T16)
        n832 = Divide(x=80000000.0, y=w1911) -> (x/y=w1908:dbl)
        n833 = Number To Decimal String(number=w1908, width (-)=i16 2) -> (decimal integer string=w1907:string)
        n834 = Concatenate Strings("445nm " ("string"), w1907, "Hz " ("string")) -> (w1905:string)
        n835 = property on="Aiming beam toggle" class="Bool (strict)"("Caption.Text"=w1905) -> ()  [unwired: 2 in, 2 out]
        n836 = call <vilib>:"Add State(s) to Queue__JKI_lib_State_Machine.vi"("State(s) in (\"\")"=w1921) -> ("States Out"=w1920:string)  [unwired: 14 in]
      }
      frame "SysConfig: Load AB setting" {
        # "Template Separator\n(You can make a copy of, or modify, this frame)"
        n837 = call "ReadAimingBeamSetting.vi"("error in (no error)"=w1923) -> ("error out"=w1924:errorcluster, "Aiming Beam Setting"=w1925:T28)  [unwired: 9 in]
        n838 = Bundle By Name(cluster=w1926, "AB Cluster"=w1925) -> (w1927:T16)
        n839 = call <vilib>:"Add State(s) to Queue__JKI_lib_State_Machine.vi"("State(s) in (\"\")"=w1929) -> ("States Out"=w1928:string)  [unwired: 14 in]
      }
      frame "---------- SystemStatus ----------" {
        # "Template Separator\n(You can make a copy of, or modify, this frame)"
        n840 = call <vilib>:"Add State(s) to Queue__JKI_lib_State_Machine.vi"("State(s) in (\"\")"=w1934) -> ("States Out"=w1933:string)  [unwired: 14 in]
      }
      frame "SystemStatus: SlowSysStatusMacro" {
        # "store system check time"
        # "Template Separator\n(You can make a copy of, or modify, this frame)"
        n841 = Tick Count (ms)() -> (millisecond timer value=w1937:u32)
        n842 = Bundle By Name(cluster=w1935, "SlowTimer"=w1937) -> (w1936:T16)
        n843 = call <vilib>:"Add State(s) to Queue__JKI_lib_State_Machine.vi"("State(s) in Front (\"\")"="Digitizer: checkTemp\nTCP: CheckConnection" ("State(s) in Front (\"\")"), "State(s) in (\"\")"=w1942) -> ("States Out"=w1941:string)  [unwired: 13 in]
      }
      frame "SystemStatus: FastSysStatusMacro" {
        # "store system check time"
        # "Template Separator\n(You can make a copy of, or modify, this frame)"
        n844 = Tick Count (ms)() -> (millisecond timer value=w1945:u32)
        n845 = Bundle By Name(cluster=w1943, "FastTimer"=w1945) -> (w1944:T16)
        n846 = call <vilib>:"Add State(s) to Queue__JKI_lib_State_Machine.vi"("State(s) in Front (\"\")"="355 Laser: CheckPWMStatus\nAimingBeam: GetPWMStatus\n" ("State(s) in Front (\"\")"), "State(s) in (\"\")"=w1950) -> ("States Out"=w1949:string)  [unwired: 13 in]
      }
      frame "---------- TCP ----------" {
        # "Template Separator\n(You can make a copy of, or modify, this frame)"
        n847 = call <vilib>:"Add State(s) to Queue__JKI_lib_State_Machine.vi"("State(s) in (\"\")"=w1955) -> ("States Out"=w1954:string)  [unwired: 14 in]
      }
      frame "TCP: Initialize" {
        # "Initialize TCP connection to aimging beam computer\n(You can make a copy of, or modify, this frame)"
        n848 = call <vilib>:"TCP Listen.vi"("error in (no error)"=w1979, "timeout ms (wait forever: -1)"=1000, "port"=u16 2100, "service name"="RTLT") -> ("error out"=w1974:errorcluster, "connection ID"=w1975:refnum<k5>, "listener ID"=w1956:refnum<k5>)  [unwired: 3 in, 2 out]
        n849 = TCP Read(connection ID=w1975, bytes to read=512, error in (no error)=w1974, 7:T15."CRLF" ("mode (standard)"), 9:10000 ("timeout ms (25000)")) -> (connection ID out=w1964:refnum<k5>, data out=w1971:string, error out=w1965:errorcluster)
        n850 = Concatenate Strings("alive" ("string"), "\r\n") -> (w1968:string)
        n851 = Equal?(x=w1971, y=w1968) -> (x = y?=w1966:bool)
        n852 = case shown="True" w1966 {
          tunnel: w1965 -> [w1983 w2004]
          tunnel: w1964 -> [_ w1998]
          tunnel: [w1984 w2002] -> w1963
          tunnel: w1961 -> [w1990 _]
          tunnel: [w1986 0] -> w1960
          tunnel: [w1985 ""] -> w1958
          tunnel: [FALSE TRUE] -> w1957
          frame False {
            # "if unsuccessful and count <10, increament count \nand try again"
            n853 = Unbundle By Name(w1990) -> ("TCP attempt count"=w1987:i32)
            n854 = Less?(x=w1987, y=1) -> (x < y?=w1988:bool)
            n855 = case shown="True" w1988 {
              tunnel: w1987 -> [w1993 w1997]
              tunnel: [w1993 w1996] -> w1986
              tunnel: ["" "TCP: Initialize"] -> w1985
              tunnel: [errorcluster {"status"=TRUE, "code"=5001, "source"="TCP/IP"} ("error in (no error)") errorcluster {"status"=FALSE, "code"=5001, "source"=""} ("error in (no error)")] -> w1984
              tunnel: w1983 -> [_ _]
              frame False {
                # "send error and shut down"
              }
              frame True {
                # "try again until 10th"
                n856 = Increment(x=w1997) -> (x+1=w1996:i32)
              }
            }
          }
          frame True {
            # "if connection is successful\nwrite TCP FVG"
            n857 = call "TcpIDFGV.vi"("Error In"=w2004, "action"=enum16{"write", "read"}."write", "connection ID in"=w1998) -> ("Error Out"=w2002:errorcluster)  [unwired: 7 in, 1 out]
          }
        }
        n858 = Bundle By Name(cluster=w1961, "TCP attempt count"=w1960, "System Status.TCP/IP"=w1957, "listener ID"=w1956) -> (w1962:T16)
        n859 = global write "GlobalVariables.vi" "TCP connected?"(w1957) -> ()
        n860 = call <vilib>:"Add State(s) to Queue__JKI_lib_State_Machine.vi"("State(s) in Front (\"\")"=w1958, "State(s) in (\"\")"=w1981) -> ("States Out"=w1980:string)  [unwired: 13 in]
      }
      frame "TCP: SyncTime" {
        # "Template Separator\n(You can make a copy of, or modify, this frame)"
        n861 = call "TcpIDFGV.vi"("Error In"=w2009, "action"=enum16{"write", "read"}."read") -> ("Error Out"=w2008:errorcluster, "connection ID out"=w2006:refnum<k5>)  [unwired: 8 in]
        n862 = call <userlib>:"Tick Count (ms)__ogtk.vi"("error in (no error)"=w2008) -> ("error out"=w2007:errorcluster, "millisecond timer value"=w2005:u32)  [unwired: 9 in]
        n863 = while {
          tunnel: w2007 -> [w2033]
          tunnel: w2006 -> [w2032]
          tunnel: w2005 -> [w2021]
          stop <- w2016 stop-if-true
          n864 = Concatenate Strings("latencycheck" ("string"), "\r\n") -> (w2028:string)
          n865 = TCP Read(connection ID=w2032, bytes to read=512, error in (no error)=w2033, 7:T15."CRLF" ("mode (standard)"), 9:2000 ("timeout ms (25000)")) -> (connection ID out=w2025:refnum<k5>, data out=w2023:string, error out=w2015:errorcluster)
          n866 = Tick Count (ms)() -> (millisecond timer value=w2022:u32)
          n867 = Subtract(x=w2022, y=w2021) -> (x-y=w2020:u32)
          n868 = Equal?(x=w2023, y=w2028) -> (x = y?=w2024:bool)
          n869 = case shown="False" w2024 {
            tunnel: w2025 -> [_ w2046]
            tunnel: w2023 -> [w2038 _]
            tunnel: [w2034 FALSE] -> w2018
            tunnel: w2015 -> [_ w2040]
            frame False {
              n870 = Concatenate Strings("synctimer" ("string"), "\r\n") -> (w2035:string)
              n871 = Equal?(x=w2038, y=w2035) -> (x = y?=w2034:bool)
              "Sync Success?" <- w2034
            }
            frame True {
              n872 = Concatenate Strings("latencycheck:" ("string"), "\r\n") -> (w2045:string)
              n873 = TCP Write(connection ID=w2046, data in=w2045, error in (no error)=w2040, 9:1000 ("timeout ms (25000)")) -> (error out=w2039:errorcluster)  [unwired: 2 out]
              n874 = call <vilib>:"Clear Errors.vi"("error in (no error)"=w2039) -> ()  [unwired: 5 in, 2 out]
            }
          }
          n875 = Greater?(x=w2020, y=u32 10000 ("x-y")) -> (0:w2017:bool)
          n876 = Or(x=w2018, y=w2017) -> (x .or. y?=w2016:bool)
        }
        n877 = call <vilib>:"Add State(s) to Queue__JKI_lib_State_Machine.vi"("State(s) in (\"\")"=w2014) -> ("States Out"=w2013:string)  [unwired: 14 in]
      }
      frame "TCP: SendSettingMacro" {
        # "Template Separator\n(You can make a copy of, or modify, this frame)"
        n878 = Unbundle By Name(w2050) -> ("CaseID"=w2049:string, "System Status.TCP/IP"=w2048:bool)
        n879 = case shown="True" w2048 {
          tunnel: w2049 -> [_ _]
          tunnel: ["" "TCP: sendSubjectID\nTCP: sendScaleBarSetting\nTCP: sendScaleMaxMin\nTCP: sendANSI\nTCP: sendRadius\nTCP: send3Dsetting\nTCP: sendFirefly\nTCP: sendPenrero"] -> w2047
          frame False {
          }
          frame True {
          }
        }
        n880 = call <vilib>:"Add State(s) to Queue__JKI_lib_State_Machine.vi"("State(s) in Front (\"\")"=w2047, "State(s) in (\"\")"=w2054) -> ("States Out"=w2053:string)  [unwired: 13 in]
      }
      frame "TCP: sendRunNum" {
        # "Template Separator\n(You can make a copy of, or modify, this frame)"
        n881 = Unbundle By Name(w2060) -> ("IDs.RunID"=w2067:i8)
        n882 = Number To Decimal String(number=w2067, width (-)=i16 3) -> (decimal integer string=w2062:string)
        n883 = call "TcpIDFGV.vi"("Error In"=w2057, "action"=enum16{"write", "read"}."read") -> ("Error Out"=w2059:errorcluster, "connection ID out"=w2064:refnum<k5>)  [unwired: 8 in]
        n884 = Concatenate Strings("!run:", w2062) -> (w2061:string)
        n885 = call "TCP_WriteRead.vi"("error in (no error)"=w2059, "data in"=w2061, "connectin ID in"=w2064) -> ("error out"=w2058:errorcluster)  [unwired: 4 in, 2 out]
        n886 = call <vilib>:"Add State(s) to Queue__JKI_lib_State_Machine.vi"("State(s) in (\"\")"=w2070) -> ("States Out"=w2069:string)  [unwired: 14 in]
      }
      frame "TCP: sendVideoSource" {
        # "Send video source \n(You can make a copy of, or modify, this frame)"
        n887 = call "TcpIDFGV.vi"("Error In"=w2071, "action"=enum16{"write", "read"}."read") -> ("Error Out"=w2073:errorcluster, "connection ID out"=w2079:refnum<k5>)  [unwired: 8 in]
        n888 = case shown="\"FrameGrabber\"" "Video Source" {
          tunnel: [0 1] -> w2077
          frame "Camera", Default {
          }
          frame "FrameGrabber" {
          }
        }
        n889 = Number To Decimal String(number=w2077) -> (decimal integer string=w2075:string)  [unwired: 1 in]
        n890 = Concatenate Strings("!invivo:" ("data in"), w2075) -> (w2074:string)
        n891 = call "TCP_WriteRead.vi"("error in (no error)"=w2073, "data in"=w2074, "connectin ID in"=w2079) -> ("error out"=w2072:errorcluster)  [unwired: 4 in, 2 out]
        n892 = call <vilib>:"Add State(s) to Queue__JKI_lib_State_Machine.vi"("State(s) in (\"\")"=w2084) -> ("States Out"=w2083:string)  [unwired: 14 in]
      }
      frame "TCP: startRun" {
        # "Template Separator\n(You can make a copy of, or modify, this frame)"
        n893 = call "TcpIDFGV.vi"("Error In"=w2087, "action"=enum16{"write", "read"}."read") -> ("Error Out"=w2089:errorcluster, "connection ID out"=w2090:refnum<k5>)  [unwired: 8 in]
        n894 = call "TCP_WriteRead.vi"("error in (no error)"=w2089, "data in"="!acquire:1", "connectin ID in"=w2090) -> ("error out"=w2088:errorcluster)  [unwired: 4 in, 2 out]
        n895 = call <vilib>:"Add State(s) to Queue__JKI_lib_State_Machine.vi"("State(s) in (\"\")"=w2096) -> ("States Out"=w2095:string)  [unwired: 14 in]
      }
      frame "TCP: stopRun" {
        # "Template Separator\n(You can make a copy of, or modify, this frame)"
        n896 = call "TcpIDFGV.vi"("Error In"=w2097, "action"=enum16{"write", "read"}."read") -> ("Error Out"=w2099:errorcluster, "connection ID out"=w2101:refnum<k5>)  [unwired: 8 in]
        n897 = call "TCP_WriteRead.vi"("error in (no error)"=w2099, "data in"="!acquire:0", "connectin ID in"=w2101) -> ("error out"=w2098:errorcluster)  [unwired: 4 in, 2 out]
        n898 = call <vilib>:"Add State(s) to Queue__JKI_lib_State_Machine.vi"("State(s) in (\"\")"=w2106) -> ("States Out"=w2105:string)  [unwired: 14 in]
      }
      frame "TCP: SyncTimer" {
        # "Template Separator\n(You can make a copy of, or modify, this frame)"
        n899 = call "TcpIDFGV.vi"("Error In"=w2112, "action"=enum16{"write", "read"}."read") -> ("Error Out"=w2113:errorcluster, "connection ID out"=w2114:refnum<k5>)  [unwired: 8 in]
        n900 = while {
          tunnel: w2114 -> [w2133]
          shift-right: [w2128] -> w2108
          shift-left: w2113 -> [w2129]
          tunnel: [w2120] -> w2111
          i -> [w2125]
          stop <- w2123 stop-if-true
          n901 = TCP Read(connection ID=w2133, bytes to read=512, error in (no error)=w2129, 7:T15."CRLF" ("mode (standard)"), 9:1000 ("timeout ms (25000)")) -> (connection ID out=w2120:refnum<k5>, data out=w2127:string, error out=w2128:errorcluster)
          "syctimer data out" <- w2127
          n902 = Equal?(x="!synctimer:", y=w2127) -> (x = y?=w2122:bool)
          n903 = Greater?(x=w2125, y=10000) -> (0:w2121:bool)
          n904 = Or(x=w2122, y=w2121) -> (x .or. y?=w2123:bool)
        }
        n905 = TCP Write(connection ID=w2111, data in="!synctimer:", error in (no error)=w2108, 9:1000 ("timeout ms (25000)")) -> (error out=w2107:errorcluster)  [unwired: 2 out]
        n906 = call <vilib>:"Add State(s) to Queue__JKI_lib_State_Machine.vi"("State(s) in (\"\")"=w2119) -> ("States Out"=w2118:string)  [unwired: 14 in]
      }
      frame "TCP: CheckConnection" {
        # "Check TCP/IP connection statuse\n(If connection is lost, throw error)"
        n907 = Unbundle By Name(w2135) -> ("System Status.TCP/IP"=w2134:bool)
        n908 = case shown="True" w2134 {
          frame False {
          }
          frame True {
            # "If TCP/IP is true check, otherwise skip"
          }
        }
        n909 = call <vilib>:"Add State(s) to Queue__JKI_lib_State_Machine.vi"("State(s) in (\"\")"=w2139) -> ("States Out"=w2138:string)  [unwired: 14 in]
      }
      frame "TCP: Close" {
        # "Close TCP connection\n()"
        n910 = call "TcpIDFGV.vi"("Error In"=w2144, "action"=enum16{"write", "read"}."read") -> ("Error Out"=w2146:errorcluster, "connection ID out"=w2147:refnum<k5>)  [unwired: 8 in]
        n911 = TCP Close Connection(connection ID=w2147, error in (no error)=w2146) -> (error out=w2140:errorcluster)  [unwired: 1 in, 1 out]
        n912 = case shown="No Error" w2140 {
          tunnel: [w2152 w2153] -> w2142
          tunnel: w2141 -> [w2151 w2153]
          frame No Error {
            w2150 = FALSE ("System Status.TCP/IP")
            n913 = Bundle By Name(cluster=w2151, "System Status.TCP/IP"=w2150) -> (w2152:T16)
            n914 = global write "GlobalVariables.vi" "TCP connected?"(w2150) -> ()
          }
          frame Error {
          }
        }
        n915 = call <vilib>:"Add State(s) to Queue__JKI_lib_State_Machine.vi"("State(s) in (\"\")"=w2149) -> ("States Out"=w2148:string)  [unwired: 14 in]
      }
      frame "TCP: sendSubjectID" {
        # "Send subject ID"
        n916 = Unbundle By Name(w2161) -> ("CaseID"=w2160:string)
        n917 = Concatenate Strings("!subject:", w2160) -> (w2157:string)
        n918 = call "TcpIDFGV.vi"("Error In"=w2154, "action"=enum16{"write", "read"}."read") -> ("Error Out"=w2156:errorcluster, "connection ID out"=w2158:refnum<k5>)  [unwired: 8 in]
        n919 = call "TCP_WriteRead.vi"("error in (no error)"=w2156, "data in"=w2157, "connectin ID in"=w2158) -> ("error out"=w2155:errorcluster)  [unwired: 4 in, 2 out]
        n920 = call <vilib>:"Add State(s) to Queue__JKI_lib_State_Machine.vi"("State(s) in (\"\")"=w2165) -> ("States Out"=w2164:string)  [unwired: 14 in]
      }
      frame "TCP: sendScaleBarSetting" {
        # "Template Separator\n(You can make a copy of, or modify, this frame)"
        n921 = call "TcpIDFGV.vi"("Error In"=w2166, "action"=enum16{"write", "read"}."read") -> ("Error Out"=w2168:errorcluster, "connection ID out"=w2170:refnum<k5>)  [unwired: 8 in]
        n922 = call "TCP_WriteRead.vi"("error in (no error)"=w2168, "data in"="!autocolor:0", "connectin ID in"=w2170) -> ("error out"=w2167:errorcluster)  [unwired: 4 in, 2 out]
        n923 = call <vilib>:"Add State(s) to Queue__JKI_lib_State_Machine.vi"("State(s) in (\"\")"=w2175) -> ("States Out"=w2174:string)  [unwired: 14 in]
      }
      frame "TCP: sendScaleMaxMin" {
        # "Template Separator\n(You can make a copy of, or modify, this frame)"
        n924 = call "TcpIDFGV.vi"("Error In"=w2177, "action"=enum16{"write", "read"}."read") -> ("Error Out"=w2179:errorcluster, "connection ID out"=w2180:refnum<k5>)  [unwired: 8 in]
        n925 = call "TCP_WriteRead.vi"("error in (no error)"=w2179, "data in"="!color:3;6", "connectin ID in"=w2180) -> ("error out"=w2178:errorcluster)  [unwired: 4 in, 2 out]
        n926 = call <vilib>:"Add State(s) to Queue__JKI_lib_State_Machine.vi"("State(s) in (\"\")"=w2185) -> ("States Out"=w2184:string)  [unwired: 14 in]
      }
      frame "TCP: sendANSI" {
        # "Template Separator\n(You can make a copy of, or modify, this frame)"
        n927 = call "TcpIDFGV.vi"("Error In"=w2186, "action"=enum16{"write", "read"}."read") -> ("Error Out"=w2189:errorcluster, "connection ID out"=w2190:refnum<k5>)  [unwired: 8 in]
        n928 = call "TCP_WriteRead.vi"("error in (no error)"=w2189, "data in"="!ansi:20", "connectin ID in"=w2190) -> ("error out"=w2187:errorcluster)  [unwired: 4 in, 2 out]
        n929 = call <vilib>:"Add State(s) to Queue__JKI_lib_State_Machine.vi"("State(s) in (\"\")"=w2195) -> ("States Out"=w2194:string)  [unwired: 14 in]
      }
      frame "TCP: sendRadius" {
        # "Template Separator\n(You can make a copy of, or modify, this frame)"
        n930 = call "TcpIDFGV.vi"("Error In"=w2197, "action"=enum16{"write", "read"}."read") -> ("Error Out"=w2199:errorcluster, "connection ID out"=w2200:refnum<k5>)  [unwired: 8 in]
        n931 = call "TCP_WriteRead.vi"("error in (no error)"=w2199, "data in"="!radius:1.0", "connectin ID in"=w2200) -> ("error out"=w2198:errorcluster)  [unwired: 4 in, 2 out]
        n932 = call <vilib>:"Add State(s) to Queue__JKI_lib_State_Machine.vi"("State(s) in (\"\")"=w2205) -> ("States Out"=w2204:string)  [unwired: 14 in]
      }
      frame "TCP: send3Dsetting" {
        # "Template Separator\n(You can make a copy of, or modify, this frame)"
        n933 = call "TcpIDFGV.vi"("Error In"=w2206, "action"=enum16{"write", "read"}."read") -> ("Error Out"=w2208:errorcluster, "connection ID out"=w2210:refnum<k5>)  [unwired: 8 in]
        n934 = call "TCP_WriteRead.vi"("error in (no error)"=w2208, "data in"="!3dset:0", "connectin ID in"=w2210) -> ("error out"=w2207:errorcluster)  [unwired: 4 in, 2 out]
        n935 = call <vilib>:"Add State(s) to Queue__JKI_lib_State_Machine.vi"("State(s) in (\"\")"=w2215) -> ("States Out"=w2214:string)  [unwired: 14 in]
      }
      frame "TCP: sendFirefly" {
        # "Template Separator\n(You can make a copy of, or modify, this frame)"
        n936 = call "TcpIDFGV.vi"("Error In"=w2216, "action"=enum16{"write", "read"}."read") -> ("Error Out"=w2218:errorcluster, "connection ID out"=w2220:refnum<k5>)  [unwired: 8 in]
        n937 = call "TCP_WriteRead.vi"("error in (no error)"=w2218, "data in"="!firefly:1", "connectin ID in"=w2220) -> ("error out"=w2217:errorcluster)  [unwired: 4 in, 2 out]
        n938 = call <vilib>:"Add State(s) to Queue__JKI_lib_State_Machine.vi"("State(s) in (\"\")"=w2225) -> ("States Out"=w2224:string)  [unwired: 14 in]
      }
      frame "TCP: sendPenrero" {
        # "Template Separator\n(You can make a copy of, or modify, this frame)"
        n939 = call "TcpIDFGV.vi"("Error In"=w2226, "action"=enum16{"write", "read"}."read") -> ("Error Out"=w2228:errorcluster, "connection ID out"=w2230:refnum<k5>)  [unwired: 8 in]
        n940 = call "TCP_WriteRead.vi"("error in (no error)"=w2228, "data in"="!pentero:0", "connectin ID in"=w2230) -> ("error out"=w2227:errorcluster)  [unwired: 4 in, 2 out]
        n941 = call <vilib>:"Add State(s) to Queue__JKI_lib_State_Machine.vi"("State(s) in (\"\")"=w2235) -> ("States Out"=w2234:string)  [unwired: 14 in]
      }
      frame "---------- UI ----------" {
        # "Do not put any code in this frame.\n(It is a separator no-op. You can make a copy of this frame to create a new UI frame)"
        n942 = call <vilib>:"Add State(s) to Queue__JKI_lib_State_Machine.vi"("State(s) in (\"\")"=w2240) -> ("States Out"=w2239:string)  [unwired: 14 in]
      }
      frame "UI: BGLoaded" {
        # "Do not put any code in this frame.\n(It is a separator no-op. You can make a copy of this frame to create a new UI frame)"
        n943 = property on="Background" class="Bool (strict)"("BoolText.Text"="Loaded!" ("Boolean Text.Text"), "Colors [4]"=cluster{u32, u32}[] [{15764023, 15764023}, {16711680, 16711680}]) -> ()  [unwired: 2 in, 2 out]
        n944 = call <vilib>:"Add State(s) to Queue__JKI_lib_State_Machine.vi"("State(s) in (\"\")"=w2247) -> ("States Out"=w2246:string)  [unwired: 14 in]
      }
      frame "UI: CaliAndiRFLoaded" {
        # "Do not put any code in this frame.\n(It is a separator no-op. You can make a copy of this frame to create a new UI frame)"
        n945 = property on="Cali&iRF alignment" class="Bool (strict)"("BoolText.Text"="Loaded!" ("Boolean Text.Text"), "Colors [4]"=cluster{u32, u32}[] [{15764023, 15764023}, {16711680, 16711680}]) -> ()  [unwired: 2 in, 2 out]
        n946 = call <vilib>:"Add State(s) to Queue__JKI_lib_State_Machine.vi"("State(s) in (\"\")"=w2254) -> ("States Out"=w2253:string)  [unwired: 14 in]
      }
      frame "UI: WFAutoScale" {
        # "Set graph auto scale.\n(UI: WFAutoScale >> T/F)"
        n947 = Equal?(x=w2255, y="F") -> (x = y?=w2256:bool)
        n948 = Equal?(x=w2255, y="T") -> (x = y?=w2258:bool)
        n949 = case shown="True" w2256 {
          frame False {
          }
          frame True {
            w2271 = 0.0 ("Y Scale.Range:Maximum")
            w2272 = 2.0 ("Y Scale.Range:Maximum")
            w2273 = u8 0 ("Y Scale.Scale Fit")
            n950 = property on="Channel 1" class="WFGraph (strict)"("YScale.ScaleFit"=w2273) -> (error out=w2270:errorcluster)  [unwired: 2 in, 1 out]
            n951 = property on="Channel 2" class="WFGraph (strict)"("YScale.ScaleFit"=w2273) -> (error out=w2269:errorcluster)  [unwired: 2 in, 1 out]
            n952 = property on="Channel 3" class="WFGraph (strict)"("YScale.ScaleFit"=w2273) -> (error out=w2268:errorcluster)  [unwired: 2 in, 1 out]
            n953 = property on="Channel 1" class="WFGraph (strict)"(error in=w2270, "YScale.Maximum"=w2272) -> (error out=w2267:errorcluster)  [unwired: 1 in, 1 out]
            n954 = property on="Channel 2" class="WFGraph (strict)"(error in=w2269, "YScale.Maximum"=w2272) -> (error out=w2266:errorcluster)  [unwired: 1 in, 1 out]
            n955 = property on="Channel 3" class="WFGraph (strict)"(error in=w2268, "YScale.Maximum"=w2272) -> (error out=w2265:errorcluster)  [unwired: 1 in, 1 out]
            n956 = property on="Channel 1" class="WFGraph (strict)"(error in=w2267, "YScale.Minimum"=w2271) -> ()  [unwired: 1 in, 2 out]
            n957 = property on="Channel 2" class="WFGraph (strict)"(error in=w2266, "YScale.Minimum"=w2271) -> ()  [unwired: 1 in, 2 out]
            n958 = property on="Channel 3" class="WFGraph (strict)"(error in=w2265, "YScale.Minimum"=w2271) -> ()  [unwired: 1 in, 2 out]
          }
        }
        n959 = case shown="True" w2258 {
          frame False {
          }
          frame True {
            w2274 = u8 2 ("Y Scale.Scale Fit")
            n960 = property on="Channel 1" class="WFGraph (strict)"("YScale.ScaleFit"=w2274) -> ()  [unwired: 2 in, 2 out]
            n961 = property on="Channel 2" class="WFGraph (strict)"("YScale.ScaleFit"=w2274) -> ()  [unwired: 2 in, 2 out]
            n962 = property on="Channel 3" class="WFGraph (strict)"("YScale.ScaleFit"=w2274) -> ()  [unwired: 2 in, 2 out]
          }
        }
        n963 = call <vilib>:"Add State(s) to Queue__JKI_lib_State_Machine.vi"("State(s) in (\"\")"=w2264) -> ("States Out"=w2263:string)  [unwired: 14 in]
      }
      frame "UI: Initialize" {
        w2275 = T29 {"Minimum"=0.0, "Maximum"=4.6, "Increment"=0.1} ("Data Entry Limits")
        w2277 = T7."Disabled and Grayed Out" ("Disabled")
        # "Disable all button on startup"
        # "Initialize the User Interface, here.\n(this is called automatically, by the Macro: Init)"
        n964 = property on="Gain 1" class="DigNum (strict)"("DisabledEnum"=w2277) -> ()  [unwired: 2 in, 2 out]
        n965 = property on="Gain 2" class="DigNum (strict)"("DisabledEnum"=w2277) -> ()  [unwired: 2 in, 2 out]
        n966 = property on="StopButton" class="Bool (strict)"("DisabledEnum"=w2277) -> ()  [unwired: 2 in, 2 out]
        n967 = property on="Sys Reconfig" class="Bool"("DisabledEnum"=w2277) -> ()  [unwired: 2 in, 2 out]
        n968 = property on="StartButton" class="Bool (strict)"("DisabledEnum"=w2277) -> ()  [unwired: 2 in, 2 out]
        n969 = property on="355nm Laser toggle" class="Bool (strict)"("DisabledEnum"=w2277) -> ()  [unwired: 2 in, 2 out]
        n970 = property on="Aiming beam toggle" class="Bool (strict)"("DisabledEnum"=w2277) -> ()  [unwired: 2 in, 2 out]
        n971 = property on="Background" class="Bool (strict)"("DisabledEnum"=w2277) -> ()  [unwired: 2 in, 2 out]
        n972 = property on="Cali&iRF alignment" class="Bool (strict)"("DisabledEnum"=w2277) -> ()  [unwired: 2 in, 2 out]
        n973 = property on="Gain 3" class="DigNum (strict)"("DisabledEnum"=w2277) -> ()  [unwired: 2 in, 2 out]
        n974 = property on="Gain 1" class="DigNum (strict)"("Data Range"=w2275) -> ()  [unwired: 2 in, 2 out]
        n975 = property on="Gain 2" class="DigNum (strict)"("Data Range"=w2275) -> ()  [unwired: 2 in, 2 out]
        n976 = property on="Gain 3" class="DigNum (strict)"("Data Range"=w2275) -> ()  [unwired: 2 in, 2 out]
        n977 = call <vilib>:"Add State(s) to Queue__JKI_lib_State_Machine.vi"("State(s) in Front (\"\")"="UI: CaliAndiRFNotReady" ("State(s) in Front (\"\")"), "State(s) in (\"\")"=w2282) -> ("States Out"=w2281:string)  [unwired: 13 in]
      }
      frame "UI: showDisclaimer" {
        # "Show disclamer window.\n(It is a separator no-op. You can make a copy of this frame to create a new UI frame)"
        n978 = call <vilib>:"Application Directory.vi"() -> ("Application Directory"=w2295:path)
        n979 = Build Path(base path=w2295, name or relative path="Disclamer.png") -> (appended path=w2293:path)
        n980 = disable-structure shown="Disabled" {
          frame Disabled {
            n981 = flat-sequence {
              frame #0 {
                n982 = call "disclaimer.vi"() -> ()  [unwired: 12 in]
              }
              frame #1 {
                n983 = Wait (ms)(milliseconds to wait=u32 250) -> ()  [unwired: 1 out]
              }
              frame #2 {
                n984 = call "SoftwareNote.vi"() -> ()  [unwired: 12 in]
              }
            }
          }
          frame Enabled {
          }
        }
        n985 = property on="Disclamer" class="Pict"() -> ("Draw Area Size"=w2291:T30)  [unwired: 2 in, 2 out]
        n986 = call <vilib>:"Read PNG File.vi"("path to PNG file"=w2293) -> ("image data"=w2290:T31)  [unwired: 8 in, 2 out]
        n987 = Unbundle By Name(w2290) -> ("Rectangle.right"=w2288:i16, "Rectangle.bottom"=w2286:i16)
        n988 = Unbundle By Name(w2291) -> ("Width"=w2289:u32, "Height"=w2287:u32)
        n989 = call <vilib>:"Draw Flattened Pixmap.vi"("image data"=w2290) -> ("new picture"=→"Disclamer":picture)  [unwired: 8 in]
        n990 = Divide(x=w2289, y=w2288) -> (x/y=w2285:dbl)
        n991 = Divide(x=w2287, y=w2286) -> (x/y=w2284:dbl)
        n992 = Max & Min(x=w2285, y=w2284) -> (min(x,y)=w2283:dbl)  [unwired: 1 out]
        n993 = property on="Disclamer" class="Pict"("ZoomFactor"=w2283) -> ()  [unwired: 2 in, 2 out]
        n994 = call <vilib>:"Add State(s) to Queue__JKI_lib_State_Machine.vi"("State(s) in (\"\")"=w2300) -> ("States Out"=w2299:string)  [unwired: 14 in]
      }
      frame "UI: CaliAndiRFNotReady" {
        # "Do not put any code in this frame.\n(It is a separator no-op. You can make a copy of this frame to create a new UI frame)"
        n995 = property on="Cali&iRF alignment" class="Bool (strict)"("BoolText.Text"="No Info" ("Boolean Text.Text"), "Colors [4]"=cluster{u32, u32}[] [{13816530, 13816530}, {16711680, 16711680}]) -> ()  [unwired: 2 in, 2 out]
        n996 = call <vilib>:"Add State(s) to Queue__JKI_lib_State_Machine.vi"("State(s) in (\"\")"=w2308) -> ("States Out"=w2307:string)  [unwired: 14 in]
      }
      frame "UI: BGnotReady" {
        # "Do not put any code in this frame.\n(It is a separator no-op. You can make a copy of this frame to create a new UI frame)"
        n997 = property on="Background" class="Bool (strict)"("BoolText.Text"="No Info" ("Boolean Text.Text"), "Colors [4]"=cluster{u32, u32}[] [{13816530, 13816530}, {16711680, 16711680}]) -> ()  [unwired: 2 in, 2 out]
        n998 = call <vilib>:"Add State(s) to Queue__JKI_lib_State_Machine.vi"("State(s) in (\"\")"=w2315) -> ("States Out"=w2314:string)  [unwired: 14 in]
      }
      frame "UI: Reset" {
        w2317 = cluster{u32, u32}[] [{13816530, 13816530}, {13816530, 13816530}] ("Colors [4]")
        # "Do not put any code in this frame.\n(It is a separator no-op. You can make a copy of this frame to create a new UI frame)"
        n999 = property on="Cali&iRF alignment" class="Bool (strict)"("BoolText.Text"="No Info" ("Boolean Text.Text"), "Colors [4]"=w2317) -> ()  [unwired: 2 in, 2 out]
        n1000 = property on="Background" class="Bool (strict)"("BoolText.Text"="No Info" ("Boolean Text.Text"), "Colors [4]"=w2317) -> ()  [unwired: 2 in, 2 out]
        n1001 = call <vilib>:"Add State(s) to Queue__JKI_lib_State_Machine.vi"("State(s) in (\"\")"=w2323) -> ("States Out"=w2322:string)  [unwired: 14 in]
      }
      frame "UI: SetButtonText" {
        # "Set button text of 355nm laser and aiming beam."
        n1002 = call <vilib>:"Add State(s) to Queue__JKI_lib_State_Machine.vi"("State(s) in (\"\")"=w2328) -> ("States Out"=w2327:string)  [unwired: 14 in]
      }
      frame "UI: DuringAquisition" {
        w2329 = T7."Disabled and Grayed Out" ("Disabled")
        # "Do not put any code in this frame.\n(It is a separator no-op. You can make a copy of this frame to create a new UI frame)"
        n1003 = property on="StopButton" class="Bool (strict)"("DisabledEnum"=T7."Enabled" ("Disabled")) -> ()  [unwired: 2 in, 2 out]
        n1004 = property on="StartButton" class="Bool (strict)"("DisabledEnum"=w2329) -> ()  [unwired: 2 in, 2 out]
        n1005 = property on="Sys Reconfig" class="Bool"("DisabledEnum"=w2329) -> ()  [unwired: 2 in, 2 out]
        n1006 = property on="355nm Laser toggle" class="Bool (strict)"("DisabledEnum"=w2329) -> ()  [unwired: 2 in, 2 out]
        n1007 = property on="Aiming beam toggle" class="Bool (strict)"("DisabledEnum"=w2329) -> ()  [unwired: 2 in, 2 out]
        n1008 = property on="Background" class="Bool (strict)"("DisabledEnum"=w2329) -> ()  [unwired: 2 in, 2 out]
        n1009 = property on="Cali&iRF alignment" class="Bool (strict)"("DisabledEnum"=w2329) -> ()  [unwired: 2 in, 2 out]
        n1010 = property on="Video Source" class="RadioBtnsControl (strict)"("DisabledEnum"=w2329) -> ()  [unwired: 2 in, 2 out]
        n1011 = property on="Quit" class="Bool"("DisabledEnum"=w2329) -> ()  [unwired: 2 in, 2 out]
        n1012 = call <vilib>:"Add State(s) to Queue__JKI_lib_State_Machine.vi"("State(s) in (\"\")"=w2335) -> ("States Out"=w2334:string)  [unwired: 14 in]
      }
      frame "UI: duringIRFAlign" {
        w2336 = T7."Disabled and Grayed Out" ("Disabled")
        # "Set UI to during iRF alignment\n(It is a separator no-op. You can make a copy of this frame to create a new UI frame)"
        n1013 = property on="StartButton" class="Bool (strict)"("DisabledEnum"=w2336) -> ()  [unwired: 2 in, 2 out]
        n1014 = property on="Sys Reconfig" class="Bool"("DisabledEnum"=w2336) -> ()  [unwired: 2 in, 2 out]
        n1015 = property on="355nm Laser toggle" class="Bool (strict)"("DisabledEnum"=w2336) -> ()  [unwired: 2 in, 2 out]
        n1016 = property on="Aiming beam toggle" class="Bool (strict)"("DisabledEnum"=w2336) -> ()  [unwired: 2 in, 2 out]
        n1017 = property on="Background" class="Bool (strict)"("DisabledEnum"=w2336) -> ()  [unwired: 2 in, 2 out]
        n1018 = property on="StopButton" class="Bool (strict)"("DisabledEnum"=w2336) -> ()  [unwired: 2 in, 2 out]
        n1019 = call <vilib>:"Add State(s) to Queue__JKI_lib_State_Machine.vi"("State(s) in (\"\")"=w2341) -> ("States Out"=w2340:string)  [unwired: 14 in]
      }
      frame "UI: duringBGAcquire" {
        w2342 = T7."Disabled and Grayed Out" ("Disabled")
        # "Do not put any code in this frame.\n(It is a separator no-op. You can make a copy of this frame to create a new UI frame)"
        n1020 = property on="StartButton" class="Bool (strict)"("DisabledEnum"=w2342) -> ()  [unwired: 2 in, 2 out]
        n1021 = property on="StopButton" class="Bool (strict)"("DisabledEnum"=w2342) -> ()  [unwired: 2 in, 2 out]
        n1022 = property on="Sys Reconfig" class="Bool"("DisabledEnum"=w2342) -> ()  [unwired: 2 in, 2 out]
        n1023 = property on="355nm Laser toggle" class="Bool (strict)"("DisabledEnum"=w2342) -> ()  [unwired: 2 in, 2 out]
        n1024 = property on="Aiming beam toggle" class="Bool (strict)"("DisabledEnum"=w2342) -> ()  [unwired: 2 in, 2 out]
        n1025 = property on="Cali&iRF alignment" class="Bool (strict)"("DisabledEnum"=w2342) -> ()  [unwired: 2 in, 2 out]
        n1026 = call <vilib>:"Add State(s) to Queue__JKI_lib_State_Machine.vi"("State(s) in (\"\")"=w2347) -> ("States Out"=w2346:string)  [unwired: 14 in]
      }
      frame "UI: ReadyForAquisition" {
        w2348 = T7."Enabled" ("Disabled")
        # "Do not put any code in this frame.\n(It is a separator no-op. You can make a copy of this frame to create a new UI frame)"
        n1027 = property on="StopButton" class="Bool (strict)"("DisabledEnum"=T7."Disabled and Grayed Out" ("Disabled")) -> ()  [unwired: 2 in, 2 out]
        n1028 = property on="StartButton" class="Bool (strict)"("DisabledEnum"=w2348) -> ()  [unwired: 2 in, 2 out]
        n1029 = property on="Sys Reconfig" class="Bool"("DisabledEnum"=w2348) -> ()  [unwired: 2 in, 2 out]
        n1030 = property on="355nm Laser toggle" class="Bool (strict)"("DisabledEnum"=w2348) -> ()  [unwired: 2 in, 2 out]
        n1031 = property on="Aiming beam toggle" class="Bool (strict)"("DisabledEnum"=w2348) -> ()  [unwired: 2 in, 2 out]
        n1032 = property on="Cali&iRF alignment" class="Bool (strict)"("DisabledEnum"=w2348) -> ()  [unwired: 2 in, 2 out]
        n1033 = property on="Video Source" class="RadioBtnsControl (strict)"("DisabledEnum"=w2348) -> ()  [unwired: 2 in, 2 out]
        n1034 = property on="Background" class="Bool (strict)"("DisabledEnum"=w2348) -> ()  [unwired: 2 in, 2 out]
        n1035 = property on="Quit" class="Bool"("DisabledEnum"=w2348) -> ()  [unwired: 2 in, 2 out]
        n1036 = call <vilib>:"Add State(s) to Queue__JKI_lib_State_Machine.vi"("State(s) in Front (\"\")"="LED: Green" ("State(s) in Front (\"\")"), "State(s) in (\"\")"=w2355) -> ("States Out"=w2354:string)  [unwired: 13 in]
      }
      frame "UI: Update" {
        # "Do not put any code in this frame.\n(It is a separator no-op. You can make a copy of this frame to create a new UI frame)"
        n1037 = Unbundle By Name(w2365) -> ("System Status"=→"System Hardware Connection Status":T1, "IDs.RunID"=→"Run #":i8, "CaseID"=→"Case #":string, "FLImDAQ"=→"FLImDAQ":T22, "SysRunning?"=→"Aquisition Status:":bool, "LJ Pinout"=→"LJ Pinout":T4, "IDs.BG ID"=→"BG #":i8, "IDs.Cali ID"=→"Calibration #":i8)
        n1038 = call <vilib>:"Add State(s) to Queue__JKI_lib_State_Machine.vi"("State(s) in (\"\")"=w2368) -> ("States Out"=w2367:string)  [unwired: 14 in]
      }
      frame "UI: Cursor Set" {
        # "Argument"
        # "Set and Unset Cursor Busy.\n(Usage: \"UI: Cursor Set >> Busy|Idle\")"
        n1039 = case shown="\"Idle\", Default" w2370 {
          tunnel: w2372 -> [w2377 w2379]
          tunnel: [w2376 w2378] -> w2371
          frame "Idle", Default {
            n1040 = call <vilib>:"Unset Busy.vi"("error in (no error)"=w2377) -> ("error out"=w2376:errorcluster)  [unwired: 10 in]
          }
          frame "Busy" {
            n1041 = call <vilib>:"Set Busy.vi"("error in (no error)"=w2379) -> ("error out"=w2378:errorcluster)  [unwired: 9 in, 1 out]
          }
        }
        n1042 = call <vilib>:"Add State(s) to Queue__JKI_lib_State_Machine.vi"("State(s) in (\"\")"=w2375) -> ("States Out"=w2374:string)  [unwired: 14 in]
      }
      frame "UI: Front Panel State" {
        # "Argument"
        # "Set Front Panel Open or Closed\n(Usage: \"UI: Front Panel State >> Open|Close\")"
        n1043 = Unbundle By Name(w2383) -> ("Core.Current VI Reference"=w2382:refnum<vi>)
        n1044 = case shown="\"Open\", \"Standard\", Default" w2381 {
          tunnel: w2385 -> [w2393 w2408 w2419 w2432 w2445]
          tunnel: [w2395 w2409 w2421 w2434 w2447] -> w2384
          tunnel: w2382 -> [w2394 w2406 w2420 w2433 w2446]
          frame "Open", "Standard", Default {
            w2388 = T12."Standard" ("State")
            n1045 = property class="VI"(reference=w2394, error in=w2393) -> (reference out=w2391:refnum<vi>, error out=w2392:errorcluster, "FP.State"=w2390:T12)
            n1046 = Not Equal?(x=w2390, y=w2388) -> (x != y?=w2389:bool)
            n1047 = case shown="True" w2389 {
              tunnel: [w2399 w2401] -> w2395
              tunnel: w2392 -> [w2398 w2401]
              tunnel: w2391 -> [w2397 _]
              tunnel: w2388 -> [w2396 _]
              frame True {
                n1048 = invoke class="VI" method="FP.Open"(reference=w2397, error in=w2398, "Activate"=TRUE, "State"=w2396) -> (error out=w2399:errorcluster)  [unwired: 1 in, 4 out]
              }
              frame False {
              }
            }
          }
          frame "Close", "Closed" {
            n1049 = property class="VI"(reference=w2406, error in=w2408) -> (reference out=w2405:refnum<vi>, error out=w2407:errorcluster, "FP.State"=w2403:T12)
            n1050 = Not Equal?(x=w2403, y=T12."Closed" ("Front Panel Window:State")) -> (x != y?=w2402:bool)
            n1051 = case shown="True" w2402 {
              tunnel: [w2410 w2413] -> w2409
              tunnel: w2407 -> [w2410 w2412]
              tunnel: w2405 -> [_ w2411]
              frame False {
              }
              frame True {
                n1052 = invoke class="VI" method="FP.Close"(reference=w2411, error in=w2412) -> (error out=w2413:errorcluster)  [unwired: 1 in, 2 out]
              }
            }
          }
          frame "Hidden", "Hide" {
            w2414 = T12."Hidden" ("State")
            n1053 = property class="VI"(reference=w2420, error in=w2419) -> (reference out=w2417:refnum<vi>, error out=w2418:errorcluster, "FP.State"=w2416:T12)
            n1054 = Not Equal?(x=w2416, y=w2414) -> (x != y?=w2415:bool)
            n1055 = case shown="True" w2415 {
              tunnel: [w2425 w2426] -> w2421
              tunnel: w2418 -> [w2424 w2426]
              tunnel: w2417 -> [w2423 _]
              tunnel: w2414 -> [w2422 _]
              frame True {
                n1056 = invoke class="VI" method="FP.Open"(reference=w2423, error in=w2424, "State"=w2422) -> (error out=w2425:errorcluster)  [unwired: 2 in, 4 out]
              }
              frame False {
              }
            }
          }
          frame "Minimize", "Minimized" {
            w2427 = T12."Minimized" ("State")
            n1057 = property class="VI"(reference=w2433, error in=w2432) -> (reference out=w2430:refnum<vi>, error out=w2431:errorcluster, "FP.State"=w2429:T12)
            n1058 = Not Equal?(x=w2429, y=w2427) -> (x != y?=w2428:bool)
            n1059 = case shown="True" w2428 {
              tunnel: [w2438 w2439] -> w2434
              tunnel: w2431 -> [w2437 w2439]
              tunnel: w2430 -> [w2436 _]
              tunnel: w2427 -> [w2435 _]
              frame True {
                n1060 = invoke class="VI" method="FP.Open"(reference=w2436, error in=w2437, "State"=w2435) -> (error out=w2438:errorcluster)  [unwired: 2 in, 4 out]
              }
              frame False {
              }
            }
          }
          frame "Maximize", "Maximized" {
            w2440 = T12."Maximized" ("State")
            n1061 = property class="VI"(reference=w2446, error in=w2445) -> (reference out=w2443:refnum<vi>, error out=w2444:errorcluster, "FP.State"=w2442:T12)
            n1062 = Not Equal?(x=w2442, y=w2440) -> (x != y?=w2441:bool)
            n1063 = case shown="True" w2441 {
              tunnel: [w2451 w2452] -> w2447
              tunnel: w2444 -> [w2450 w2452]
              tunnel: w2443 -> [w2449 _]
              tunnel: w2440 -> [w2448 _]
              frame True {
                n1064 = invoke class="VI" method="FP.Open"(reference=w2449, error in=w2450, "State"=w2448) -> (error out=w2451:errorcluster)  [unwired: 2 in, 4 out]
              }
              frame False {
              }
            }
          }
        }
        n1065 = call <vilib>:"Add State(s) to Queue__JKI_lib_State_Machine.vi"("State(s) in (\"\")"=w2387) -> ("States Out"=w2386:string)  [unwired: 14 in]
      }
      frame "---------- 355 Laser ----------" {
        # "Template Separator\n(You can make a copy of, or modify, this frame)"
        n1066 = call <vilib>:"Add State(s) to Queue__JKI_lib_State_Machine.vi"("State(s) in (\"\")"=w2457) -> ("States Out"=w2456:string)  [unwired: 14 in]
      }
      frame "355 Laser: Check Dewelling" {
        # "if time laser start time is less than 7.5s before, wait 250ms then check again."
        # "Template Separator\n(You can make a copy of, or modify, this frame)"
        n1067 = Unbundle By Name(w2465) -> ("Laser start tic"=w2462:u32)
        n1068 = Tick Count (ms)() -> (millisecond timer value=w2463:u32)
        n1069 = Subtract(x=w2463, y=w2462) -> (x-y=w2461:u32)
        n1070 = Greater?(x=w2461, y=u32 5000) -> (0:w2459:bool)
        n1071 = case shown="False" w2459 {
          tunnel: ["355 Laser: Check Dewelling" ""] -> w2458
          frame False {
            n1072 = Wait (ms)(milliseconds to wait=u32 250) -> ()  [unwired: 1 out]
          }
          frame True {
          }
        }
        n1073 = call <vilib>:"Add State(s) to Queue__JKI_lib_State_Machine.vi"("State(s) in Front (\"\")"=w2458, "State(s) in (\"\")"=w2468) -> ("States Out"=w2467:string)  [unwired: 13 in]
      }
      frame "355 Laser: Laser enable/disable" {
        # "Laser enable/disable\n(Usage: \"LabJack: Laser enable/disable >> 1|0\")"
        n1074 = Unbundle By Name(w2473) -> ("LJ Pinout.Laser Start/Stop"=w2481:string)
        n1075 = call "LabJack_FGV.vi"("Operation(Read)"=enum16{"Write", "Read"}."Read" ("Operation")) -> ("Read data"=w2483:i32)  [unwired: 9 in, 1 out]
        n1076 = call <vilib>:"LJM_eWriteName.vi"("Handle In"=w2483, "Name"=w2481, "Value"=1.0, "error in"=w2487) -> ("Handle Out"=w2482:i32, "error out"=w2480:errorcluster)  [unwired: 10 in]
        n1077 = call <userlib>:"Wait (ms)__ogtk.vi"("error in (no error)"=w2480, "milliseconds to wait"=u32 250) -> ("error out"=w2479:errorcluster)  [unwired: 8 in, 1 out]
        n1078 = call <vilib>:"LJM_eWriteName.vi"("Handle In"=w2482, "Name"=w2481, "Value"=0.0, "error in"=w2479) -> ("error out"=w2476:errorcluster)  [unwired: 10 in, 1 out]
        n1079 = call <userlib>:"Tick Count (ms)__ogtk.vi"("error in (no error)"=w2476) -> ("error out"=w2475:errorcluster, "millisecond timer value"=w2472:u32)  [unwired: 9 in]
        n1080 = Bundle By Name(cluster=w2473, "Laser start tic"=w2472) -> (w2474:T16)
        n1081 = call <vilib>:"Add State(s) to Queue__JKI_lib_State_Machine.vi"("State(s) in (\"\")"=w2489) -> ("States Out"=w2488:string)  [unwired: 14 in]
      }
      frame "355 Laser: Dewelling" {
        # "Wait some time (ms)\n(355 Laser: Dewelling >> #)"
        n1082 = Fract/Exp String To Number(string=w2493, default (0 dbl)=0) -> (number=w2491:i32)  [unwired: 2 in, 1 out]
        n1083 = Wait (ms)(milliseconds to wait=w2491) -> ()  [unwired: 1 out]
        n1084 = call <vilib>:"Add State(s) to Queue__JKI_lib_State_Machine.vi"("State(s) in (\"\")"=w2497) -> ("States Out"=w2496:string)  [unwired: 14 in]
      }
      frame "355 Laser: Init" {
        # "Initilize 355nm laser\n(Start laser, enable interlock)"
        n1085 = call <vilib>:"Add State(s) to Queue__JKI_lib_State_Machine.vi"("State(s) in Front (\"\")"="355 Laser: CheckControllerStatus", "State(s) in (\"\")"=w2503) -> ("States Out"=w2502:string)  [unwired: 13 in]
      }
      frame "355 Laser: Close" {
        # "Template Separator\n(You can make a copy of, or modify, this frame)"
        n1086 = call <vilib>:"Add State(s) to Queue__JKI_lib_State_Machine.vi"("State(s) in Front (\"\")"="355 Laser: Laser enable/disable\n355 Laser: Dewelling >>1000", "State(s) in (\"\")"=w2509) -> ("States Out"=w2508:string)  [unwired: 13 in]
      }
      frame "355 Laser: CheckControllerStatus" {
        # "if average < 1, laser on\nif average > 9, laser off\nif 1<average<9, interlock open, blink indicator"
        # "take 10 measuremt and look at average"
        # "Check 355 laser controller status\nBy probing Emisison Lamp negative terminal voltage"
        n1087 = Unbundle By Name(w2517) -> ("LJ Pinout.Laser Ready"=w2520:string)
        n1088 = call "LabJack_FGV.vi"("Operation(Read)"=enum16{"Write", "Read"}."Read" ("Operation")) -> ("Read data"=w2521:i32)  [unwired: 9 in, 1 out]
        n1089 = for {
          N: 10 -> [_]
          tunnel: w2521 -> [w2555]
          tunnel: w2520 -> [w2554]
          shift-right: [w2553] -> w2512
          shift-left: w2519 -> [w2552]
          tunnel: [w2550] -> w2510 mode=indexing
          n1090 = call <vilib>:"LJM_eReadName.vi"("Handle In"=w2555, "Name"=w2554, "error in"=w2552) -> ("Value"=w2550:dbl, "error out"=w2553:errorcluster)  [unwired: 10 in, 1 out]
          n1091 = Wait (ms)(milliseconds to wait=u32 50) -> ()  [unwired: 1 out]
        }
        n1092 = case shown="No Error" w2512 {
          selector: w2512 -> [w2529 w2548]
          tunnel: [w2531 FALSE] -> w2514
          tunnel: [w2530 w2548] -> w2513
          tunnel: [w2525 nan] -> w2511
          tunnel: w2510 -> [w2527 _]
          frame No Error {
            n1093 = call-poly <vilib>:"Mean.vi"("X"=w2527) -> ("mean"=w2525:dbl)  [unwired: 1 out]
            n1094 = Less?(x=w2525, y=2.0) -> (x < y?=w2526:bool)
            n1095 = case shown="False" w2526 {
              tunnel: [w2534 TRUE] -> w2531
              tunnel: w2525 -> [w2537 _]
              tunnel: w2529 -> [w2533 w2544]
              tunnel: [w2532 w2544] -> w2530
              frame False {
                n1096 = Greater?(x=w2537, y=9.0) -> (0:w2535:bool)
                n1097 = case shown="False" w2535 {
                  tunnel: [FALSE FALSE] -> w2534
                  tunnel: w2533 -> [_ w2541]
                  tunnel: [errorcluster {"status"=TRUE, "code"=5002, "source"="355 Laser"} ("error out") w2541] -> w2532
                  frame False {
                    n1098 = property on="355 Laser" class="Bool (strict)"("Blinking"=FALSE) -> ()  [unwired: 2 in, 2 out]
                  }
                  frame True {
                    n1099 = property on="355 Laser" class="Bool (strict)"("Blinking"=FALSE) -> ()  [unwired: 2 in, 2 out]
                  }
                }
              }
              frame True {
                n1100 = property on="355 Laser" class="Bool (strict)"("Blinking"=FALSE) -> ()  [unwired: 2 in, 2 out]
              }
            }
          }
          frame Error {
          }
        }
        "laser EM lamp V" <- w2511
        n1101 = Bundle By Name(cluster=w2517, "System Status.355 Laser"=w2514) -> (w2518:T16)
        n1102 = call <vilib>:"Add State(s) to Queue__JKI_lib_State_Machine.vi"("State(s) in (\"\")"=w2524) -> ("States Out"=w2523:string)  [unwired: 14 in]
      }
      frame "355 Laser: CheckPWMStatus" {
        # "Check 355 laser PWM status\n(Read LJ DIO#EF_ENABLE register to determine PWM status)"
        n1103 = Unbundle By Name(w2565) -> ("LJ Pinout.355 PWM"=w2564:string)
        n1104 = call "LabJack_FGV.vi"("Operation(Read)"=enum16{"Write", "Read"}."Read" ("Operation"), "error in (no error)"=w2558) -> ("error out"=w2561:errorcluster, "Read data"=w2562:i32)  [unwired: 8 in]
        n1105 = Concatenate Strings(w2564, "_EF_ENABLE" ("string")) -> (w2560:string)
        n1106 = call <vilib>:"LJM_eReadName.vi"("Handle In"=w2562, "Name"=w2560, "error in"=w2561) -> ("Value"=w2557:dbl, "error out"=w2559:errorcluster)  [unwired: 10 in, 1 out]
        n1107 = Greater Than 0?(x=w2557) -> (x > 0?=w2556:bool)
        n1108 = case shown="True" w2556 {
          frame False {
            # "PWM is off\nset color to dark green"
            n1109 = local write "355nm Laser toggle"(FALSE ("355nm Laser")) -> ()
          }
          frame True {
            # "PWM is on\nset color to light green"
            n1110 = local write "355nm Laser toggle"(TRUE ("355nm Laser")) -> ()
          }
        }
        n1111 = call <vilib>:"Add State(s) to Queue__JKI_lib_State_Machine.vi"("State(s) in (\"\")"=w2569) -> ("States Out"=w2568:string)  [unwired: 14 in]
      }
      frame "355 Laser: Start" {
        # "Template Separator\n(You can make a copy of, or modify, this frame)"
        n1112 = call <vilib>:"Add State(s) to Queue__JKI_lib_State_Machine.vi"("State(s) in Front (\"\")"="LabJack: 355_PWM_Start", "State(s) in (\"\")"=w2577) -> ("States Out"=w2576:string)  [unwired: 13 in]
      }
      frame "355 Laser: Stop" {
        # "Template Separator\n(You can make a copy of, or modify, this frame)"
        n1113 = call <vilib>:"Add State(s) to Queue__JKI_lib_State_Machine.vi"("State(s) in Front (\"\")"="LabJack: 355_PWM_Stop", "State(s) in (\"\")"=w2583) -> ("States Out"=w2582:string)  [unwired: 13 in]
      }
      frame "---------- Utility ----------" {
        # "Template Separator\n(You can make a copy of, or modify, this frame)"
        n1114 = call <vilib>:"Add State(s) to Queue__JKI_lib_State_Machine.vi"("State(s) in (\"\")"=w2588) -> ("States Out"=w2587:string)  [unwired: 14 in]
      }
      frame "Utility: Dewelling" {
        # "Main loop dewell\n(Dewelling >> #)"
        n1115 = Fract/Exp String To Number(string=w2591, default (0 dbl)=0) -> (number=w2589:i32)  [unwired: 2 in, 1 out]
        n1116 = Wait (ms)(milliseconds to wait=w2589) -> ()  [unwired: 1 out]
        n1117 = call <vilib>:"Add State(s) to Queue__JKI_lib_State_Machine.vi"("State(s) in (\"\")"=w2596) -> ("States Out"=w2595:string)  [unwired: 14 in]
      }
      frame "Utility: SetAllChanManualGain" {
        # "Template Separator\n(You can make a copy of, or modify, this frame)"
        n1118 = property on="Auto gain ch1" class="Bool (strict)"("Val(Sgnl)"=FALSE ("Value (Signaling)")) -> ()  [unwired: 2 in, 2 out]
        n1119 = property on="Auto gain ch2" class="Bool (strict)"("Val(Sgnl)"=FALSE ("Value (Signaling)")) -> ()  [unwired: 2 in, 2 out]
        n1120 = property on="Auto gain ch3" class="Bool (strict)"("Val(Sgnl)"=FALSE ("Value (Signaling)")) -> ()  [unwired: 2 in, 2 out]
        n1121 = call <vilib>:"Add State(s) to Queue__JKI_lib_State_Machine.vi"("State(s) in (\"\")"=w2604) -> ("States Out"=w2603:string)  [unwired: 14 in]
      }
      frame "Utility: SetAllChanAutoGain" {
        # "Template Separator\n(You can make a copy of, or modify, this frame)"
        n1122 = property on="Auto gain ch1" class="Bool (strict)"("Val(Sgnl)"=TRUE ("Value (Signaling)")) -> ()  [unwired: 2 in, 2 out]
        n1123 = property on="Auto gain ch2" class="Bool (strict)"("Val(Sgnl)"=TRUE ("Value (Signaling)")) -> ()  [unwired: 2 in, 2 out]
        n1124 = property on="Auto gain ch3" class="Bool (strict)"("Val(Sgnl)"=TRUE ("Value (Signaling)")) -> ()  [unwired: 2 in, 2 out]
        n1125 = call <vilib>:"Add State(s) to Queue__JKI_lib_State_Machine.vi"("State(s) in (\"\")"=w2612) -> ("States Out"=w2611:string)  [unwired: 14 in]
      }
      frame "---------- SysLog ----------" {
        # "Template Separator\n(You can make a copy of, or modify, this frame)"
        n1126 = call <vilib>:"Add State(s) to Queue__JKI_lib_State_Machine.vi"("State(s) in (\"\")"=w2617) -> ("States Out"=w2616:string)  [unwired: 14 in]
      }
      frame "SysLog: OpenLogFile" {
        # "Template Separator\n(You can make a copy of, or modify, this frame)"
        n1127 = call <vilib>:"Add State(s) to Queue__JKI_lib_State_Machine.vi"("State(s) in (\"\")"=w2622) -> ("States Out"=w2621:string)  [unwired: 14 in]
      }
      frame "---------- Graph ----------" {
        # "Template Separator\n(You can make a copy of, or modify, this frame)"
        n1128 = call <vilib>:"Add State(s) to Queue__JKI_lib_State_Machine.vi"("State(s) in (\"\")"=w2627) -> ("States Out"=w2626:string)  [unwired: 14 in]
      }
      frame "Graph: AddCursors" {
        # "Add BG and DC cursor to all graphs\n(You can make a copy of, or modify, this frame)"
        n1129 = property on="Channel 2" class="WFGraph (strict)"() -> ("CrsrList"=w2631:T17)  [unwired: 2 in, 2 out]
        n1130 = property on="Channel 3" class="WFGraph (strict)"() -> ("CrsrList"=w2630:T17)  [unwired: 2 in, 2 out]
        n1131 = property on="Channel 1" class="WFGraph (strict)"() -> ("CrsrList"=w2635:T17)  [unwired: 2 in, 2 out]
        n1132 = for {
          tunnel: w2635 -> [w2648] mode=indexing
          tunnel: u32[] [200, 220, 10, 25] -> [w2644] mode=indexing
          tunnel: [w2647] -> w2633 mode=indexing
          tunnel: u32[] [6618880, 6618880, 16711680, 16711680] -> [w2643] mode=indexing
          tunnel: w2631 -> [w2646] mode=indexing
          tunnel: w2630 -> [w2645] mode=indexing
          tunnel: [w2642] -> w2629 mode=indexing
          tunnel: [w2641] -> w2628 mode=indexing
          n1133 = Bundle By Name(cluster=w2648, "Position.X"=w2644, "Color"=w2643) -> (w2647:T18)
          n1134 = Bundle By Name(cluster=w2646, "Position.X"=w2644, "Color"=w2643) -> (w2642:T18)
          n1135 = Bundle By Name(cluster=w2645, "Position.X"=w2644, "Color"=w2643) -> (w2641:T18)
        }
        n1136 = property on="Channel 1" class="WFGraph (strict)"("CrsrList"=w2633) -> ()  [unwired: 2 in, 2 out]
        n1137 = property on="Channel 2" class="WFGraph (strict)"("CrsrList"=w2629) -> ()  [unwired: 2 in, 2 out]
        n1138 = property on="Channel 3" class="WFGraph (strict)"("CrsrList"=w2628) -> ()  [unwired: 2 in, 2 out]
        n1139 = call <vilib>:"Add State(s) to Queue__JKI_lib_State_Machine.vi"("State(s) in (\"\")"=w2640) -> ("States Out"=w2639:string)  [unwired: 14 in]
      }
      frame "---------- Temp ----------" {
        # "Template Separator\n(You can make a copy of, or modify, this frame)"
        n1140 = call <vilib>:"Add State(s) to Queue__JKI_lib_State_Machine.vi"("State(s) in (\"\")"=w2653) -> ("States Out"=w2652:string)  [unwired: 14 in]
      }
    }
    n1141 = Not(x=w164) -> (.not. x?=w163:bool)
    n1142 = local write "ML?"(w163) -> ()
    "ML?" <- TRUE ("main loop running?")
  }
  n1143 = while {
    tunnel: w38 -> [w2666]
    tunnel: w27 -> [w2665]
    tunnel: [w2664] -> w36
    tunnel: w21 -> [w2663]
    tunnel: [w2662] -> w32
    tunnel: w9 -> [w2660]
    tunnel: w14 -> [w2659]
    tunnel: w5 -> [w2654]
    stop <- w2657 stop-if-true
    # "Data Aquisition Loop"
    n1144 = event shown="[1] <Start digitizer>: User Event" {
      selector: w2665 -> [_ _]
      dyn-events: [_ _] -> w2664
      timeout: 20 -> [_ _]
      tunnel: w2666 -> [w2672 w2677]
      tunnel: [w2667 _] -> w2657
      tunnel: w2663 -> [w2671 w2684]
      tunnel: [w2671 w2683] -> w2662
      tunnel: w2660 -> [_ w2681]
      tunnel: w2659 -> [w2670 w2676]
      tunnel: w2654 -> [_ w2673]
      event Timeout {
        # "use queue to stop data loop\nwhen queue ref is released, error will stop this loop"
        n1145 = event-data() -> ()  [unwired: 1 in, 3 out]
        n1146 = Get Queue Status(queue=w2670) -> (error out=w2668:errorcluster)  [unwired: 2 in, 7 out]
        n1147 = Get Queue Status(queue=w2672) -> (error out=w2669:errorcluster)  [unwired: 2 in, 7 out]
        n1148 = Merge Errors(w2669, w2668) -> (w2667:errorcluster)
      }
      event User Event {
        w2682 = enum16{"Write", "Read"}."Read" ("Operation")
        n1149 = event-data() -> ()  [unwired: 1 in, 4 out]
        n1150 = call "FLImDAQ_FGV.vi"() -> ("Read data"=w2679:T5)  [unwired: 10 in, 1 out]
        n1151 = Unbundle By Name(w2679) -> ("Waveform to Avg"=w2678:i32)
        n1152 = call "Digitizer1_FGV.vi"("Operation"=w2682) -> ("Read data"=w2674:refnum<k15>)  [unwired: 9 in, 1 out]
        n1153 = call "Digitizer2_FGV.vi"("Operation"=w2682) -> ("Read data"=w2680:refnum<k15>)  [unwired: 9 in, 1 out]
        n1154 = while {
          tunnel: w2684 -> [w2731]
          tunnel: [w2730] -> w2683
          tunnel: w2680 -> [w2724]
          tunnel: w2674 -> [w2723]
          tunnel: w2681 -> [w2721]
          shift-right: [w2710] -> _
          shift-left: u32 0 ("millisecond timer value") -> [w2709]
          tunnel: w2678 -> [w2706]
          tunnel: w2677 -> [w2703]
          tunnel: w2676 -> [w2701]
          tunnel: w2673 -> [w2688]
          i -> [w2705]
          stop <- w2696 stop-if-true
          w2693 = enum16{"write", "read"}."read" ("action")
          w2711 = 65536
          # "send data for processing"
          # "acquire data and send it to processing loop"
          n1155 = Tick Count (ms)() -> (millisecond timer value=w2710:u32)
          n1156 = Multiply(x=w2706, y=w2705) -> (x*y=w2685:i32)
          "Fetch Record #" <- w2685
          n1157 = Subtract(x=w2710, y=w2709) -> (x-y=→"Aquisition loop timing(ms)":u32)
          n1158 = property class="niScope"(reference=w2723, "Fetch Record Number"=w2685) -> (reference out=w2735:refnum<k15>, error out=w2734:errorcluster, "Records Done"=w2686:i32, "Vertical Range"=w2719:dbl, "Vertical Offset"=w2717:dbl)  [unwired: 1 in]
          n1159 = call-poly <instrlib>:"niScope Fetch (poly).vi"("timeout"=1.0, "error in"=w2734, "channels"="0,1", "instrument handle"=w2735) -> ("error out"=w2722:errorcluster, "wfm"=w2707:i16[][])  [unwired: 4 in, 2 out]
          "error out" <- w2722
          n1160 = property class="niScope"(reference=w2724, error in=w2722, "Fetch Record Number"=w2685) -> (reference out=w2728:refnum<k15>, error out=w2725:errorcluster, "Vertical Range"=w2713:dbl, "Vertical Offset"=w2712:dbl)
          n1161 = Divide(x=w2707, y=w2711) -> (x/y=w2720:dbl[][])
          n1162 = Subtract(x=w2686, y=w2685) -> (x-y=→"Record Backlog":i32)
          n1163 = Multiply(x=w2720, y=w2719) -> (x*y=w2718:dbl[][])
          n1164 = call "V1FGV.vi"("action"=w2693) -> ("Error Out"=w2695:errorcluster, "V1 out"=w2692:dbl)  [unwired: 9 in]
          n1165 = call-poly <instrlib>:"niScope Fetch (poly).vi"("timeout"=1.0, "error in"=w2725, "channels"="0,1", "instrument handle"=w2728) -> ("error out"=w2699:errorcluster, "wfm"=w2714:i16[][])  [unwired: 4 in, 2 out]
          "error out 2" <- w2699
          n1166 = call "V2FGV.vi"("Error In"=w2695, "action"=w2693) -> ("Error Out"=w2694:errorcluster, "V2 out"=w2691:dbl)  [unwired: 8 in]
          n1167 = Add(x=w2718, y=w2717) -> (x+y=w2702:dbl[][])
          n1168 = call "V3FGV.vi"("Error In"=w2694, "action"=w2693) -> ("V3 out"=w2690:dbl)  [unwired: 8 in, 1 out]
          n1169 = Divide(x=w2714, y=w2711) -> (x/y=w2716:dbl[][])
          n1170 = Enqueue Element(queue=w2703, element=w2702) -> (error out=w2698:errorcluster)  [unwired: 2 in, 2 out]
          n1171 = Bundle("V1 out"=w2692, "V2 out"=w2691, "V3 out"=w2690) -> (w2689:T32)  [unwired: 1 in]
          n1172 = Multiply(x=w2716, y=w2713) -> (x*y=w2715:dbl[][])
          n1173 = Add(x=w2715, y=w2712) -> (x+y=w2700:dbl[][])
          n1174 = Enqueue Element(queue=w2688, element=w2689) -> (error out=w2687:errorcluster)  [unwired: 2 in, 2 out]
          n1175 = Enqueue Element(queue=w2701, element=w2700) -> (error out=w2697:errorcluster)  [unwired: 2 in, 2 out]
          n1176 = Bundle(w2705, w2702, w2700) -> (w2704:cluster{i32, dbl[][], dbl[][]})  [unwired: 1 in]
          n1177 = Merge Errors(w2687, w2697, w2698, w2699) -> (w2696:errorcluster)
          "aquisition loop Error Out" <- w2696
          n1178 = Send Notification(notification=w2704, notifier=w2731) -> (notifier out=w2730:refnum<notifier>)  [unwired: 1 in, 1 out]
          n1179 = case shown="Error .." w2696 {
            tunnel: w2721 -> [_ w2738]
            frame No Error {
            }
            frame Error {
              # "Send user event to signal aquisition has stoped"
              n1180 = Generate User Event(priority (normal)=usereventprio."high priority", user event=w2738, event data cluster=TRUE ("event data")) -> ()  [unwired: 1 in, 2 out]
            }
          }
        }
      }
    }
    n1181 = Unbundle By Name(w2657) -> ("status"=w2656:bool)
    n1182 = Not(x=w2656) -> (.not. x?=w2655:bool)
    n1183 = local write "Aq L?"(w2655) -> ()
    "Aq L?" <- TRUE ("Aq L?")
  }
  n1184 = Control Help Window(0:w3, 1:TRUE ("Show")) -> ()
  n1185 = property on="Cali&iRF alignment" class="Bool (strict)"("DisabledEnum"=T7."Disabled and Grayed Out" ("Disabled")) -> ()  [unwired: 2 in, 2 out]
  n1186 = property on="Background" class="Bool (strict)"("DisabledEnum"=T7."Disabled and Grayed Out" ("Disabled")) -> ()  [unwired: 2 in, 2 out]
  n1187 = Unregister For Events(event registration refnum=w12, error in=w23) -> (error out=w24:errorcluster)
  n1188 = Destroy User Event(user event=w9, error in=w24) -> ()  [unwired: 1 out]
  n1189 = Release Notifier(notifier=w17, error in (no error)=w15) -> (error out=w16:errorcluster)  [unwired: 1 in, 2 out]
  n1190 = call <vilib>:"Simple Error Handler.vi"("error in (no error)"=w16) -> ()  [unwired: 4 in, 5 out]
  n1191 = Release Notifier(notifier=w32, error in (no error)=w31) -> (error out=w30:errorcluster)  [unwired: 1 in, 2 out]
  n1192 = Unregister For Events(event registration refnum=w36, error in=w34) -> (error out=w35:errorcluster)
  n1193 = call <vilib>:"Simple Error Handler.vi"("error in (no error)"=w30) -> ()  [unwired: 4 in, 5 out]
  n1194 = Destroy User Event(user event=w25, error in=w35) -> ()  [unwired: 1 out]
